vi "MAIN - PECT - Autonics - Pulses - encoder  - DATN.vi"() -> ()   [LabVIEW 2018]
uses:
  Control 1.ctl
  <vilib>/DAQmx/read.llb/DAQmx Read (Counter U32 1Chan 1Samp).vi
  <vilib>/DAQmx/write.llb/DAQmx Write (Analog 1D Wfm NChan NSamp).vi
  <vilib>/DAQmx/create/channels.llb/DAQmx Create Channel (AO-Voltage-Basic).vi
  <vilib>/DAQmx/configure/timing.llb/DAQmx Timing (Sample Clock).vi
  <vilib>/DAQmx/miscellaneous.llb/DAQmx Fill In Error Info.vi
  <vilib>/NI/Modbus Library/API/Wrapper/Create Serial Master.vi
  <vilib>/DAQmx/create/channels.llb/DAQmx Create Channel (CI-Count Edges).vi
  <vilib>/Instr/_visa.llb/VISA Configure Serial Port (Instr).vi
  <vilib>/DAQmx/create/channels.llb/DAQmx Create Channel (AI-Voltage-Basic).vi
  <vilib>/DAQmx/configure/trigger.llb/DAQmx Start Trigger (Digital Edge).vi
  <vilib>/Utility/file.llb/Write Delimited Spreadsheet (DBL).vi
  Global_data.vi
  <vilib>/NI/Modbus Library/API/Master/Modbus Master.lvclass
  <resource>/objmgr/daqmx.rc
  <vilib>/Platform/NI_3dgraph.lvlib
  <vilib>/NI/Modbus Library/API/Wrapper/API Main.lvlib
panel:
  in  "COM 2":refnum<visa-resource-name>="COM12"
  out "Record path 2":path=path "H:/ECT - HUY/Data Collection/PECT_default.tdms" caption="selected path"
  out "element":dbl
  out "Z UP Limit":bool
  out "X L Limit":bool
  out "Y Back Limit":bool
  out "Limit Sensor":bool[](array[boolean])
  out "exception status":u8=1
  out "Get data Count":u32
  out "Numeric":i32=2806
  in  "low cutoff freq: fl":dbl=40.0 format="%0.2f"
  out "Step Y Number":i16=40
  out "X complete":bool
  out "Y complete":bool
  out "Z complete":bool
  out "Init pulses":i32
  out "Enum":T1(ring)
  in  "Stop Scan":bool
  out "Count Y step":i32=40
  in  "file path (dialog if empty)":path=path "filename.csv"
  out "Init pulses":i32
  in  "2D Array In":dbl[][](array[numeric])
  out "Output":dbl[][](array[numeric])=[[-0.0001790493709009043, -0.00021608679972030288, -0.00017178819100872444, -0.00011604105280902267, -0.0001994752461753511, -0.00021272668316708356, -0.00020639924249934213, -0.00014664339243822874, -0.00017436953505067972, -0.00019232423942228908, -0.00020273889745070755, -0.00020023639620674223, -0.00021020175039261797, -0.00024359074063426845, -0.00025876701562411054, -0.0002315828160822644, -0.000218566532529974, -0.00022261110447328696, -0.00022419728135687593, -0.00021114867784790235], [-0.0001963216140493263, -0.00023418906975044163, -0.00019071104323735346, -0.00013561106555918905, -0.00021894092056332169, -0.0002380097564790417, -0.00022843365448356728, -0.00016484725168345368, -0.00018622702377611884, -0.0002031771821091096, -0.00021081005970256892, -0.00021079969316724172, -0.0002271961406782536, -0.00025867959672668146, -0.0002805477174689687, -0.00025169216832681383, -0.00024361837001232386, -0.0002460942661830067, -0.00025163155596480587, -0.00023850761662319413], [-0.0002081151685617141, -0.00024400248184640837, -0.00020530435414019364, -0.00015627208737854694, -0.00023343018819932046, -0.00025538735407167404, -0.0002426185756957697, -0.00017673621895774542, -0.0001884261364834142, -0.00020296298573773547, -0.00020689734150807198, -0.00020789870881424144, -0.00023303031169973065, -0.0002620433904484054, -0.0002927385048416735, -0.00026513120745070336, -0.0002623455059006857, -0.0002622931063832219, -0.0002723410056474345, -0.00026120095337865343], [-0.00021457669052360028, -0.00024580131506114853, -0.00021534259616615235, -0.00017707145978625594, -0.00024277432324072614, -0.0002634501756083648, -0.0002474815580328412, -0.00018035729110340779, -0.00017981645877632527, -0.00019103188878050962, -0.00019061251357036652, -0.00019092090894159974, -0.0002261842240830498, -0.00025290078244219645, -0.00029425058621379736, -0.0002719206490032662, -0.00027423707068698067, -0.00027095537529682294, -0.00028540039652625703, -0.00027818437178321], [-0.0002165532745462377, -0.00024080481503230104, -0.00022087843392969066, -0.00019612739674833984, -0.00024735703614447817, -0.00026179399751959966, -0.00024256467997271856, -0.0001746401468614477, -0.00016065367790241147, -0.00016820409511847725, -0.00016363767940926702, -0.0001613497984716203, -0.00020647740181520442, -0.00023164618907714658, -0.00028488226638064863, -0.00027270018072409613, -0.000279710414873696, -0.00027273738980523356, -0.0002908735183031882, -0.00028908854550584433], [-0.00021620251694465416, -0.00023191698381073642, -0.0002230430950540133, -0.00021189455575721262, -0.000248364593678687, -0.00025152551858054987, -0.00022906405584130745, -0.00016001345604591943, -0.00013303439830161627, -0.0001381008470128873, -0.00013039961934990015, -0.00012384473248759544, -0.00017604836265911004, -0.0002001991370624047, -0.0002659011078593801, -0.00026867397840984845, -0.0002805644526617879, -0.0002698382980896863, -0.00029061166615720457, -0.0002947373856622016], [-0.0002157254797925199, -0.00022212977202190273, -0.00022315741434436424, -0.0002226726523806592, -0.00024690632677282307, -0.00023481366928883914, -0.00020881322768553142, -0.00013812478894460224, -0.00010058736075877969, -0.00010585283298349471, -9.708551728018332e-05, -8.517212615390558e-05, -0.0001387897057735744, -0.00016136384157795173, -0.00023898033700647282, -0.0002608466807478317, -0.0002788558845781622, -0.00026484809900805505, -0.0002871755028366991, -0.0002961480206756994], [-0.00021603641939044876, -0.0002137231836458718, -0.00022219074041363376, -0.00022690682897293785, -0.00024332666516588709, -0.00021415534240340744, -0.00018362219034633118, -0.00011110986228331579, -6.715165937727641e-05, -7.697170186800155e-05, -7.038763051885923e-05, -5.229359285039217e-05, -9.933000506378957e-05, -0.00011790253758049707, -0.00020572727094640524, -0.0002493148562135129, -0.00027541277335358435, -0.00025964181137286095, -0.0002827092296243134, -0.0002940627952659853], [-0.0002169035043912259, -0.00020781952269694447, -0.00022081576894823676, -0.00022401076191313866, -0.00023740842840563013, -0.0001917459427821051, -0.00015533101101162725, -8.141641520546632e-05, -3.677306791602386e-05, -5.649535159940166e-05, -5.6193755228333385e-05, -3.1374570531067514e-05, -6.222214101951097e-05, -7.321569423801837e-05, -0.00016804225033060192, -0.00023388406793614126, -0.00027083358556014275, -0.0002553354757163593, -0.0002787410131176154, -0.00028917189047822194], [-0.00021821840400503695, -0.00020555322517243173, -0.00022034774503409873, -0.00021534561977678158, -0.00022979264904391533, -0.00017033179451306918, -0.00012640397324480395, -5.262818969476758e-05, -1.398636303178314e-05, -4.9120187782888784e-05, -5.9371588115307225e-05, -2.752973568791086e-05, -3.26114629992328e-05, -3.1644664187363905e-05, -0.00012894743083449733, -0.00021544938621673951, -0.00026614129881038454, -0.0002531053772280908, -0.0002768499554673797, -0.0002827767249597747], [-0.00021971567038365364, -0.00020713831401349483, -0.00022165114634856327, -0.0002038973398694431, -0.0002210396548240753, -0.0001527773117743509, -9.958363826534627e-05, -2.845518478239613e-05, -2.6082336154050964e-06, -5.736457030775313e-05, -8.184897875371244e-05, -4.306583216132521e-05, -1.5057604216061476e-05, 2.2469734134167307e-06, -9.237523956017249e-05, -0.00019543032274441964, -0.00026224558475180636, -0.00025371208640000836, -0.0002780424531135554, -0.0002765116974136287], [-0.00022052625489159868, -0.00021153638649906194, -0.00022415935129582384, -0.00019290682443156605, -0.00021179517790951077, -0.000140448560702563, -7.68519230142442e-05, -1.139633755409264e-05, -4.163431709398868e-06, -8.029008212839112e-05, -0.00012117111044296271, -7.601679390248275e-05, -1.1402969221721744e-05, 2.4607611376235503e-05, -6.186919659878845e-05, -0.0001751738305670672, -0.00025898183190682655, -0.0002563885732456842, -0.0002814375012646017, -0.00027118440513041776], [-0.00021988279893717967, -0.00021701712244094618, -0.00022686972936503732, -0.00018527605280643528, -0.00020245299908791797, -0.00013432743404399178, -6.010979957391232e-05, -3.243898764096996e-06, -1.8127979503059985e-05, -0.00011355463987814014, -0.0001706470877882284, -0.00012079385206513905, -2.117789106222904e-05, 3.3133968422815324e-05, -4.030060753122157e-05, -0.000156731644411396, -0.00025622278267901574, -0.00025973560929374966, -0.00028533901671389666, -0.0002663448542542593], [-0.00021869524322359803, -0.00022292426583044034, -0.00022957159776307474, -0.00018383638416337618, -0.0001945769406340673, -0.0001355721125065627, -5.1955433580346336e-05, -5.643698180804457e-06, -4.291334196600185e-05, -0.00015151877239863703, -0.00022183959462050186, -0.00017019364465732482, -4.275491119068702e-05, 2.5883392461202408e-05, -3.089693044187013e-05, -0.00014317907781097663, -0.00025452421274259167, -0.0002632516325736184, -0.00028859636972583796, -0.0002622101624978803], [-0.00021807632184133938, -0.0002284186202907209, -0.0002323572455590235, -0.0001900311787604277, -0.00018990549150125526, -0.00014456579006633455, -5.46658082891437e-05, -1.9712568408037506e-05, -7.552321975018862e-05, -0.00018753529480355913, -0.00026537002704973313, -0.00021653468959309443, -7.321263061649177e-05, 2.4565443021117017e-06, -3.6057369009415835e-05, -0.00013757609722403995, -0.0002547341878125775, -0.00026658745573897216, -0.000290396337119048, -0.0002587860129133193], [-0.00021824693795097824, -0.00023255751295601923, -0.00023399679294544822, -0.00020236475540265017, -0.00018868118663900764, -0.00016001554143172964, -6.873145959066136e-05, -4.4853397061619775e-05, -0.00011128138135851808, -0.00021465512057469716, -0.000292593471797456, -0.00025183562991200337, -0.0001079597385926145, -3.4452551596194855e-05, -5.556996295917865e-05, -0.00014129442097626788, -0.0002562315642660627, -0.00026846214110181395, -0.00028935633732405167, -0.0002549654006845474], [-0.0002190124687307584, -0.0002336622211642379, -0.0002332963769903964, -0.0002178223751308139, -0.00019078123902312172, -0.0001796474326783027, -9.356994101829101e-05, -7.90461361291862e-05, -0.00014567379324155125, -0.0002281437284970527, -0.0002977797118965701, -0.00027021284524483564, -0.00014255262148564225, -8.114311690595594e-05, -8.78966978550659e-05, -0.00015415177964126035, -0.0002578570700149576, -0.00026786253133153325, -0.00028423282585513746, -0.00024932257209576026], [-0.0002209894909040635, -0.00023258605736042274, -0.00023086429244803877, -0.00023391976265087818, -0.00019676517724666418, -0.00020170765223306072, -0.0001285461921752386, -0.00012121792800615701, -0.00017673068398968775, -0.00022815716173888757, -0.0002815327615322853, -0.0002711249085974501, -0.00017565725777078135, -0.00013480518097056665, -0.00013190373585706197, -0.00017625062963520528, -0.0002599023668556832, -0.0002652779776636336, -0.0002763846957686009, -0.00024273056924111434], [-0.00022448103990486967, -0.00022995484575597924, -0.00022743601940196714, -0.0002481970708736233, -0.00020664541522020206, -0.00022476654008557993, -0.0001720715687212734, -0.0001699835813927554, -0.00020468330736781067, -0.00021885354686507642, -0.0002498421058764067, -0.0002581606172256971, -0.0002075110135537385, -0.00019290046149774386, -0.0001853412547840414, -0.00020658123717641648, -0.0002627214515831056, -0.0002619127314163819, -0.00026816486335987447, -0.0002368600699934201], [-0.00022802990418745867, -0.00022622419022567952, -0.0002228884128917209, -0.00025791375153528303, -0.00021898606478551724, -0.00024649601851316205, -0.00022058652422207118, -0.00022214184915811137, -0.00023037764919299486, -0.000205995517291265, -0.0002113554698303403, -0.00023710405402949976, -0.00023905235376544837, -0.00025198658293546297, -0.00024399485024785734, -0.00024167752450870387, -0.0002651814590316536, -0.00025759189670814583, -0.00026058977742285817, -0.00023226638767936438], [-0.0002300235694701249, -0.00022125297023187392, -0.00021732519949127418, -0.0002611085228502331, -0.00023120009393905704, -0.00026436343821099103, -0.00026961587606469124, -0.0002743180137223314, -0.0002556005725403328, -0.00019656950892984765, -0.00017604240959999146, -0.00021504501881012845, -0.0002713622800732665, -0.0003089994852245627, -0.0003027606077411855, -0.00027720026736847807, -0.00026616966575180104, -0.0002522647713825805, -0.0002540660232651379, -0.00022905691282559034], [-0.00023031743114585324, -0.00021680314617144973, -0.00021203134821502073, -0.0002583345727852635, -0.00024209408782833487, -0.00027807224975191, -0.00031614712423959183, -0.00032422132876758214, -0.00028371709390885656, -0.00019828078315496482, -0.00015446067853002506, -0.00020121901701677415, -0.0003068498770553863, -0.0003622575261073985, -0.00035804543010948923, -0.00030981177381165636, -0.00026605710122575964, -0.0002471325457118192, -0.00024995322491891056, -0.0002283275116831034], [-0.00022925437043681916, -0.00021401448875409037, -0.0002088160831638262, -0.00025150958339171647, -0.0002509707154453953, -0.0002881907102463919, -0.0003576459341527987, -0.0003696771078116846, -0.0003171003697626006, -0.00021620692345035095, -0.00015457114485214422, -0.00020271610595858428, -0.0003466357604870324, -0.0004104672349350977, -0.00040669711287723287, -0.00033683898800164654, -0.00026552925347518835, -0.0002434535026422614, -0.0002489311645275244, -0.00023087596507603142], [-0.0002264612182456818, -0.00021276085301088522, -0.00020767484086169075, -0.00024205196843881532, -0.0002559667863855121, -0.0002942275945028369, -0.0003908887088360669, -0.00040764857374859945, -0.00035487226071887704, -0.0002503856107330272, -0.00017811286436661064, -0.0002216305231266466, -0.0003888450233332074, -0.00045060196307922067, -0.00044463481359120066, -0.00035502106061481575, -0.0002638439938361884, -0.00024050401004175898, -0.00024963464684412545, -0.00023542214933805396], [-0.00022185157032744967, -0.00021183543416352854, -0.00020739389445804599, -0.00023168051739573883, -0.00025599774849148493, -0.0002953195608101783, -0.00041319213849610147, -0.00043504694261567575, -0.00039361464277166015, -0.00029609294256662325, -0.0002216759940034561, -0.0002560863217725626, -0.0004293861275892121, -0.00047988354297975617, -0.0004689864061062383, -0.0003621240268398204, -0.00025980701284888767, -0.00023720275290790589, -0.0002498913303349351, -0.00023971721343348656], [-0.00021693350273486924, -0.00021145578995785362, -0.0002081366037133001, -0.00022290009811798493, -0.00025163705106371215, -0.00029243134032067367, -0.0004244182852297879, -0.0004511395398208171, -0.0004298355191403678, -0.00034709338188631655, -0.0002791656300998686, -0.0003018670029816817, -0.0004647697640870717, -0.0004975110739241333, -0.0004793376586334462, -0.0003591041475856944, -0.0002544362664846818, -0.00023447160214393973, -0.00024951846271172376, -0.00024363904996959392], [-0.00021329358353667366, -0.00021184599040914576, -0.00021003291024809193, -0.00021724072743727323, -0.0002443000969422626, -0.00028670062840463473, -0.00042560628093420323, -0.0004562722685524474, -0.0004597014113322034, -0.00039567051251991354, -0.00034218831377467486, -0.00035226127247373236, -0.0004915854197046193, -0.0005035696601653908, -0.00047688331048914394, -0.0003483540322680844, -0.0002492522603439124, -0.00023275086686351098, -0.0002491402431873957, -0.00024770821903495697], [-0.0002111396353729235, -0.00021141958914673055, -0.0002117295808062563, -0.00021403939548415504, -0.00023465741620782958, -0.0002780322951085844, -0.00041675502640222024, -0.00045031625597639555, -0.00047806778777350744, -0.0004331240508939618, -0.000399951477056998, -0.00039841333258215823, -0.0005057534016851654, -0.0004977962905883442, -0.00046237570541058336, -0.00033129712796658474, -0.00024399196409514382, -0.00023102257587082238, -0.000248294776308949, -0.0002506553417561917], [-0.0002099507444262268, -0.0002092158988426249, -0.00021186994635026286, -0.0002112926091797961, -0.0002232120564579377, -0.00026642921614820035, -0.0003983369808760436, -0.0004339299808601262, -0.00048159860180152763, -0.00045248659421314157, -0.00044336761498752885, -0.00043214549596420297, -0.0005048678971218534, -0.0004809285840771671, -0.00043700613799681556, -0.0003102589439363604, -0.00023838864446115195, -0.00022810695668517775, -0.00024679485465158024, -0.0002515946310250091], [-0.00021067038348659365, -0.00020606210782104627, -0.00021080963190575445, -0.0002083997893175182, -0.00021257105479688052, -0.00025352476878359037, -0.00037331291966480676, -0.00040993579354319746, -0.0004706887564761208, -0.00045244163459400716, -0.00046794050450717044, -0.0004492170481778541, -0.0004901664343216188, -0.0004559537249311319, -0.00040456079458894845, -0.0002889715853185166, -0.00023366889282603123, -0.00022448506679441718, -0.00024621160093700467, -0.00025164985053700503], [-0.00021366771338320652, -0.00020303500058891939, -0.00020923510335117343, -0.0002050845727041466, -0.0002047091969661673, -0.000241372618557922, -0.00034476877382140676, -0.0003817668060293851, -0.00044809290861421314, -0.0004352568307386161, -0.0004727370419142802, -0.0004488493531815277, -0.0004648618686007768, -0.00042650700417049686, -0.0003688275214315945, -0.00027044749710170533, -0.0002307677151872061, -0.00022096729112685773, -0.00024799835519775937, -0.00025155341466853894], [-0.0002173084769872, -0.00020026823278414523, -0.0002070542311710319, -0.00020015250188109603, -0.0002000513255038163, -0.00023053307114026707, -0.0003145428960598818, -0.0003514169088703672, -0.0004168005893498, -0.0004049406521434125, -0.00045892801090032485, -0.00043201284544968493, -0.00043222145004994, -0.0003943985377895462, -0.00033206395965079336, -0.0002553862802279327, -0.00022864313887302132, -0.00021671670797258902, -0.0002513135661791916, -0.0002504859997362087], [-0.00021973461338017225, -0.00019724665283585296, -0.00020386728125797345, -0.00019303995213347785, -0.00019775389133368237, -0.00022113133999670208, -0.00028392228670897843, -0.00032062204951827534, -0.0003801517417093541, -0.0003667313828948429, -0.0004294578127631808, -0.000401957035489061, -0.0003950886551043458, -0.0003608958802723376, -0.0002961293070477822, -0.00024331685442430598, -0.00022617809942428353, -0.00021102885268738103, -0.0002543656101950207, -0.0002472402816616325], [-0.0002206887087533825, -0.00019500358276167314, -0.00020086006895508185, -0.00018551371218804118, -0.00019833298545421894, -0.0002139552840322318, -0.00025547719890561295, -0.00029169894301897276, -0.00034299697181030576, -0.0003275896561808281, -0.00039026103052590584, -0.0003647320171096934, -0.00035746465701116427, -0.0003281200463100698, -0.00026407214123304323, -0.00023474498730902127, -0.0002235404145244195, -0.0002051469041781228, -0.000256505003176994, -0.00024213742773926926], [-0.0002200062764148962, -0.00019375515469029908, -0.00019918211441145514, -0.00017991991813800373, -0.00020152554963176646, -0.00020951090642230656, -0.00023129959162584632, -0.0002663889238850078, -0.00030955488127189235, -0.00029309743662717797, -0.0003476285707827778, -0.00032647388485934105, -0.00032274144912027534, -0.0002972445447394015, -0.0002388416732305998, -0.0002294946477340975, -0.00022115126064498232, -0.00020067986068869094, -0.00025731397996606176, -0.00023589062632908483], [-0.00021686501048460982, -0.0001927440667472552, -0.00019806643691439203, -0.00017708949207530245, -0.0002058442692531113, -0.00020618400807497113, -0.00021149103316543856, -0.0002446761750965164, -0.00028122237605033434, -0.0002654526859166579, -0.0003058249429885723, -0.00029101730155135785, -0.000291745117435337, -0.00026848333783359955, -0.00022112253118916798, -0.00022569318997046374, -0.00021784905484434, -0.00019767179850903316, -0.000255268465696977, -0.0002284943150350112], [-0.00021043663370824, -0.00019038513747410106, -0.00019675034047064027, -0.00017654974493035679, -0.0002090745294200981, -0.00020230231875758425, -0.00019566018647480983, -0.00022577217944666841, -0.00025804974232601294, -0.00024379879870907277, -0.0002671600070910888, -0.00025998657099316445, -0.00026429413659799506, -0.00024140387303679157, -0.0002098830622664534, -0.00022164186657965684, -0.00021293451613360603, -0.00019578932957465926, -0.00024893013102892866, -0.00021929410847857517], [-0.0002021357888212106, -0.0001870778760571564, -0.00019551363356000266, -0.000178176974235068, -0.00021082247374670446, -0.00019815233667355887, -0.00018409509890723527, -0.00021030691659366246, -0.00024044554621526285, -0.00022741798909153496, -0.0002343581826668769, -0.00023512599364226318, -0.00024112221561539, -0.00021724126955392428, -0.000204939399155446, -0.00021717071560331536, -0.00020731246535632408, -0.0001957224564036516, -0.0002394008241276193, -0.00020983643831130536], [-0.00019382942194914182, -0.00018317870523813437, -0.0001941112103125784, -0.00018154963028758908, -0.0002110898918876586, -0.00019433174451707544, -0.00017680372114179353, -0.00019922649032049974, -0.00022822032632894076, -0.00021510680810691435, -0.00020900005958195828, -0.00021705235159035809, -0.00022264956117902177, -0.00019770591605515302, -0.00020531190524905422, -0.0002122949737994994, -0.00020212454072031719, -0.00019755405791488725, -0.00022795337113398761, -0.00020207182781544972], [-0.0001860175705082779, -0.0001783739737073655, -0.0001910117451761513, -0.00018471750733600224, -0.00020913083625901524, -0.00019010122188476558, -0.00017207907477439187, -0.0001915344510088294, -0.00021925744913525898, -0.0002041423647054525, -0.00019054980596271143, -0.00020373106516728863, -0.00020773161302148867, -0.00018257527716223493, -0.00020792284781900178, -0.00020584489308989734, -0.000196989713765576, -0.00019930193401179568, -0.00021503376289837978, -0.00019561464459860213], [-0.00017879376008740275, -0.0001717064584350822, -0.00018476309314842052, -0.00018559894976801113, -0.00020480590122671713, -0.00018486588023933215, -0.00016786158341463436, -0.00018632062834771958, -0.0002113369243466768, -0.0001927692658922637, -0.0001773979918470673, -0.000192720077801755, -0.00019471455939610964, -0.00017140872935831122, -0.0002092132971061693, -0.00019705222472525888, -0.00019122525071702326, -0.00019850372670889883, -0.0002003325890270278, -0.0001897144334209195], [-0.00017343641024908027, -0.0001645933515064986, -0.00017635294578014458, -0.00018396783905104928, -0.00019949500913999697, -0.00018033933777524512, -0.00016440626646809994, -0.0001839362261671692, -0.00020391295827511952, -0.00018227037554012504, -0.00016925239197810617, -0.00018410608388137045, -0.00018403838738988154, -0.00016503978419010398, -0.00020830391074392815, -0.00018691686106615292, -0.00018556973370605252, -0.00019506772040221027, -0.00018574873069300904, -0.00018561174053887373], [-0.00017072220231029167, -0.00015819074237620814, -0.00016763614819010307, -0.00018045455462836063, -0.00019466693943955872, -0.00017771660432387183, -0.00016193896298990346, -0.00018494468575313595, -0.00019698459277234757, -0.00017454903012389424, -0.00016588496465524613, -0.00017817091981232706, -0.00017615332756484511, -0.00016375340095344665, -0.00020522285615905828, -0.00017730056045200775, -0.00018138934379164674, -0.00018951734167179345, -0.00017358717597895645, -0.00018419831111197126], [-0.00016915541325304186, -0.00015219351624800453, -0.000159387643616336, -0.00017499789685608905, -0.00019022581352073735, -0.00017628500034547884, -0.00015987065781666518, -0.00018775833623527194, -0.00018928909091247247, -0.0001699845375634102, -0.00016548833479338235, -0.00017429041320676276, -0.00017007185805722504, -0.00016547036080744384, -0.00019907210230285348, -0.00016847439743328252, -0.0001782680546483853, -0.00018176685618924958, -0.00016420877832335964, -0.00018438800922252266], [-0.00016699278247163732, -0.00014632730804036223, -0.00015232752566938373, -0.00016791096343255624, -0.00018508281548767526, -0.0001747089667313538, -0.00015781921803309854, -0.00019041650760125324, -0.0001799236005517093, -0.00016849412127567173, -0.00016551579334978146, -0.0001714686137914978, -0.00016480792515188684, -0.0001678295020885283, -0.00018984750127565286, -0.00016082647855846302, -0.00017569466438790288, -0.00017270321628911137, -0.0001574938738205245, -0.00018481938214680652], [-0.00016410001152501047, -0.00014186259211697652, -0.00014802534339525275, -0.0001607067167921014, -0.00017926766205520264, -0.00017362990827877317, -0.00015709070779591425, -0.00019241246169750953, -0.00016995278281397436, -0.00017066850882714937, -0.000165319202652333, -0.0001703036409766573, -0.00016109745107906193, -0.00016983565748885515, -0.00018004226780877347, -0.00015609624105985404, -0.00017472749272075955, -0.00016484129434302108, -0.00015467782742988045, -0.00018573758749646646], [-0.00016084986376483854, -0.00014033310805317, -0.0001475633763562273, -0.0001551088133728666, -0.00017301756284093285, -0.00017348401648135253, -0.00015918266819851812, -0.00019316370053601255, -0.00016069312051794453, -0.00017571765849012586, -0.00016438158502175663, -0.00017070108696826125, -0.0001596368322853963, -0.0001707002480070413, -0.00017208685775431734, -0.00015536636226637715, -0.00017603568890164553, -0.00016091901728864863, -0.0001565167845689712, -0.0001870328244625366], [-0.00015639969111759348, -0.00014129264741064712, -0.00015004387540913482, -0.00015140032271324447, -0.00016517213699152912, -0.00017305218302528583, -0.00016357685144966633, -0.00019107583144396811, -0.00015203980741492103, -0.00018086043613242501, -0.00016068854804591332, -0.00017020492358917234, -0.00015921944021283184, -0.00016847929553197305, -0.0001660848191834801, -0.00015743309256275803, -0.00017859765998816737, -0.00016138241415626468, -0.00016150211035736994, -0.00018695987427767152], [-0.0001504756550961793, -0.00014427879543442088, -0.000153722090473438, -0.00014937719908233657, -0.0001550955403737276, -0.00017103835956116913, -0.0001691974521458063, -0.000184640068940407, -0.00014319975198578104, -0.00018196067900595574, -0.00015228770627697188, -0.00016604089893557626, -0.00015756368737504176, -0.0001616084349536709, -0.0001612433447031117, -0.00016013398959609758, -0.00018075365158499827, -0.00016507700159299442, -0.00016674765418513843, -0.00018358679723059178], [-0.00014464095866733445, -0.00014888851792758603, -0.00015847136364592444, -0.0001497133019401787, -0.00014464187544306444, -0.00016794480540712094, -0.00017567288627944044, -0.0001741000659076595, -0.00013436338150374372, -0.00017652875428644799, -0.00013900091737155222, -0.00015657036525163273, -0.00015343911368784907, -0.00015071842497925772, -0.00015741003278019194, -0.00016256346628940217, -0.00018202343394861827, -0.0001717513783275823, -0.00017089798421427577, -0.0001768366253569898], [-0.00014021021504910525, -0.0001550240847418352, -0.00016372606648647203, -0.0001522709920078521, -0.0001358951182032081, -0.00016434583840006442, -0.00018207259631463843, -0.00015999238209924403, -0.00012533789422008133, -0.00016301045477310448, -0.00012087633606610963, -0.00014015025580808166, -0.00014529433732743229, -0.00013644834938181596, -0.00015362968705793373, -0.00016368063193316143, -0.0001822704530242622, -0.00018047156328695156, -0.00017338649061151255, -0.00016766064947300145], [-0.0001371883010907824, -0.00015998602159566187, -0.00016734360622347455, -0.00015560208178362796, -0.0001298119700644633, -0.00015933515494750972, -0.0001858539978381677, -0.00014170567666968968, -0.00011371780323028192, -0.00013914038658818968, -9.647965896794272e-05, -0.00011427184123393407, -0.00012966121739446494, -0.0001180767767005736, -0.00014713504793646345, -0.00016115426427446705, -0.0001803058414129692, -0.00018818343053249136, -0.00017271968582245265, -0.0001560928612509508], [-0.00013512164576080093, -0.0001614900884085481, -0.00016759861043179163, -0.000157979487867152, -0.00012671329854465826, -0.00015213002775576329, -0.00018404700490480715, -0.00011851980504043111, -9.675349740125017e-05, -0.00010372273216048208, -6.52605838859649e-05, -7.744379778600909e-05, -0.00010362010717435838, -9.453986064667831e-05, -0.00013461268718219753, -0.00015307911859663466, -0.00017501861748123876, -0.00019230678326665612, -0.00016836300504778634, -0.000142559856841612], [-0.0001346116757000703, -0.0001593100492798174, -0.00016448382508829802, -0.0001589892764972834, -0.00012773083849505762, -0.00014372431447308605, -0.00017597402246963614, -9.147320172413903e-05, -7.327284950731094e-05, -5.856542512870308e-05, -2.8501290426535472e-05, -3.1721359869363655e-05, -6.641378896274364e-05, -6.570773037198677e-05, -0.00011457455983197515, -0.00013994496313747898, -0.00016751755682483868, -0.00019234482792972706, -0.0001618195614770581, -0.00012966197619128372], [-0.0001358810317147463, -0.00015426651546611957, -0.00015855271914321997, -0.00015870014973728107, -0.00013282044152148828, -0.00013535896029822497, -0.00016136206945210722, -6.217036253441596e-05, -4.28250031337396e-05, -6.911738209184823e-06, 1.1299140246548087e-05, 1.8919184375547002e-05, -1.9148134360130742e-05, -3.169628646025775e-05, -8.617115885197618e-05, -0.00012248153230588754, -0.00015926364746193453, -0.00018897323032828796, -0.00015519428865971158, -0.00011944154031763923], [-0.00013731686752789865, -0.00014627964208726446, -0.00015027761599318602, -0.0001561476147983465, -0.00014009720845709235, -0.0001267299036625518, -0.00013922967793058953, -3.039275564033217e-05, -4.800175297657583e-06, 4.779986232539453e-05, 5.1773779457146146e-05, 6.996490226551452e-05, 3.588152175987118e-05, 8.456214243815832e-06, -4.783196571215599e-05, -0.0001002032683363515, -0.00014956492442800076, -0.0001818339405597301, -0.00014877456642661824, -0.00011212799639204532], [-0.0001376237380223827, -0.00013620350359520167, -0.0001406759823552109, -0.00014998399133876739, -0.00014698075062368442, -0.00011719445859587237, -0.0001092923113923984, 3.4081056138387383e-06, 4.000069373872109e-05, 0.00010125505621800049, 8.941129165612044e-05, 0.00011539334598236785, 9.465593105455368e-05, 5.506887886252282e-05, 6.908492349612383e-07, -7.254467161760779e-05, -0.00013791887622742298, -0.00017074905773294298, -0.00014176288017819783, -0.00010725469375568245], [-0.00013684129874163772, -0.00012698036323311075, -0.000132538051196774, -0.00014153492407491426, -0.00015275428679373433, -0.00010805310205338516, -7.428502884131334e-05, 3.711880536450517e-05, 8.707049226566906e-05, 0.00014701132803420988, 0.00011778600817575861, 0.00014679779218529886, 0.00014938321354322943, 0.000104728249110864, 5.593465342915854e-05, -4.108305711105972e-05, -0.0001252784085827366, -0.0001581946848339174, -0.00013534108131697462, -0.00010508260295318504], [-0.00013486006254005353, -0.00012096183850079587, -0.0001284688841031844, -0.00013319707694759222, -0.00015681708165782987, -0.00010022993223313646, -3.777363450107804e-05, 6.886985228148068e-05, 0.0001305497962792463, 0.000178931463008139, 0.0001302367976741374, 0.00015665895648558567, 0.00019134426189420899, 0.000152542215341403, 0.00011270759217153759, -7.922193309237158e-06, -0.00011291844425178992, -0.0001470663246446076, -0.0001305050341417497, -0.00010547597809917701], [-0.0001311917136155357, -0.00011854515329906903, -0.00012830876444580586, -0.00012558771260558557, -0.0001578354397061294, -9.311920335685654e-05, -2.2467428044768006e-06, 9.730838899234956e-05, 0.00016601561593673417, 0.00019310586813440014, 0.00012301885372871697, 0.0001412577706695825, 0.0002141013235983872, 0.00019401821707107705, 0.00016632126846071252, 2.5995111192238587e-05, -0.0001004789302455518, -0.00013803753706143063, -0.0001268936652260872, -0.0001073229082476819], [-0.00012502312180468454, -0.00011885542800798773, -0.0001306913781935863, -0.00011893601811575026, -0.000154286146253884, -8.596917367130995e-05, 2.9223055931967487e-05, 0.00012115187445066455, 0.00018960122856041817, 0.0001882953455529194, 9.544702246854463e-05, 0.00010118693214517666, 0.00021364861223296082, 0.00022463720363575038, 0.00021152984273965086, 5.8667624762502243e-05, -8.783296028221609e-05, -0.00013123195884452363, -0.00012400711212480833, -0.00010945628234779702], [-0.0001175920332645141, -0.00012148737676645482, -0.00013456166538736332, -0.00011480034659066586, -0.00014734510054162375, -7.994882108361412e-05, 5.2326165625653925e-05, 0.00013784480361868356, 0.00019766883933897833, 0.00016453875269898527, 4.889895892876313e-05, 4.00079406305022e-05, 0.00018837645832830117, 0.00023897285383033678, 0.00024170411497220073, 8.584659561846307e-05, -7.671413863280171e-05, -0.00012811153417364302, -0.0001235341461005221, -0.0001119768155519521], [-0.00011073888193134651, -0.0001258082596827005, -0.00013809825972990568, -0.00011467686350870136, -0.00013829246388562255, -7.649994609324785e-05, 6.32311393845477e-05, 0.00014402391747898, 0.0001885336120149815, 0.00012482410366557, -1.1157888753554612e-05, -3.4046454265641846e-05, 0.00014121391719891692, 0.00023386620967224755, 0.0002514772885735539, 0.0001029067884977912, -6.943047489586622e-05, -0.0001292679444411457, -0.0001268980133788157, -0.0001153221424620033], [-0.0001047296327158706, -0.00012976066616450684, -0.0001386300101499649, -0.00011766051924777879, -0.00012778594145599134, -7.579233846657582e-05, 6.042314947392671e-05, 0.00013852499167196775, 0.00016471695179091743, 7.605424596430002e-05, -7.455380871402087e-05, -0.00010798154346389373, 8.038151411852296e-05, 0.0002103319053651572, 0.00023973892810755758, 0.00010767759168635489, -6.63601107989166e-05, -0.00013354374606004867, -0.00013345454360122293, -0.00011859203794866574], [-9.95799413894792e-05, -0.00013100088621080877, -0.00013450100391171511, -0.00012167540813057785, -0.00011658134532758699, -7.746443078980939e-05, 4.430580123484379e-05, 0.00012109722076506825, 0.00013044586732132747, 2.6667987409374067e-05, -0.00012944174678540012, -0.0001680972211710232, 1.6810185072864067e-05, 0.00017168769132371552, 0.00020771637388542104, 9.880088373222067e-05, -6.738213989441501e-05, -0.00013845368909545623, -0.00014119522952489236, -0.00012061112048289066], [-9.657607873522073e-05, -0.0001295733477046073, -0.00012678719732973735, -0.00012540393435989984, -0.00010736999655015268, -8.297224301626743e-05, 1.5047283961667351e-05, 9.078985883825309e-05, 8.9043074027996e-05, -1.714903043647034e-05, -0.00016688788682481769, -0.0002045664848381347, -4.037690713844244e-05, 0.00012110947595051977, 0.00015688544821593556, 7.470254902255773e-05, -7.331717117388045e-05, -0.0001432173403470762, -0.00014938412487555328, -0.00012185824697459602], [-9.648024881366533e-05, -0.00012618216368176505, -0.00011745312447093009, -0.00012799814353481667, -0.00010265822171590805, -9.284721177416078e-05, -2.559555604009396e-05, 4.761410115322086e-05, 4.351312901748616e-05, -5.183177973138928e-05, -0.0001816447248019215, -0.0002121404980918208, -8.494162415797861e-05, 6.216843859732299e-05, 9.03882717625485e-05, 3.558141340474774e-05, -8.495694364270799e-05, -0.0001472992804255214, -0.00015723401108144394, -0.00012252351822082674], [-9.798274395027458e-05, -0.00012012058928547419, -0.00010773306872560381, -0.0001278954727353815, -0.00010248893268937145, -0.00010567994414527326, -7.29133422679145e-05, -5.343614721634374e-06, -3.34998281340676e-06, -7.545898315405343e-05, -0.0001724715863591561, -0.00019089947508595453, -0.0001129926387609722, -7.860923886791882e-07, 1.3593592848294006e-05, -1.541821269138155e-05, -0.00010092692719796022, -0.00014873599166442125, -0.0001624429621619912, -0.00012176291289599933], [-9.956054467338306e-05, -0.00011125253368178371, -9.84869306676333e-05, -0.00012352211607181453, -0.00010588061072737236, -0.0001193775915704267, -0.00012156932428064073, -6.392611006315711e-05, -5.023683125419259e-05, -8.968279518152197e-05, -0.00014341854747669872, -0.00014706836363469894, -0.0001255587348114838, -6.415241069209279e-05, -6.85002889604519e-05, -7.401802233430489e-05, -0.00011911506258907752, -0.00014613492164287922, -0.00016308904972539041, -0.0001187178378218301], [-0.00010046649651081381, -0.00010103445879613634, -9.11728416933405e-05, -0.00011520486639218612, -0.00011167871735503869, -0.00013310879396772127, -0.0001675627054012769, -0.0001252935222823444, -9.881491628845052e-05, -0.0001006492300604199, -0.00010497717222184011, -9.378473155756926e-05, -0.0001296546307104473, -0.00012725380185244634, -0.00015274883191985188, -0.00013663899179380823, -0.00013882945491881446, -0.00014046307570532608, -0.00015991326050426857, -0.00011396952604226379], [-0.0001003908235543971, -9.096601183869457e-05, -8.625232294776249e-05, -0.00010453770268752278, -0.00011844702690064039, -0.00014539622919146865, -0.00020748140420947386, -0.00018631100758152372, -0.0001508429979253656, -0.00011541775088221191, -6.990052883895995e-05, -4.638242344691228e-05, -0.0001343830594482849, -0.0001901775080197718, -0.00023601955119829932, -0.00019894139653670734, -0.00015898819130751723, -0.0001334199910609183, -0.00015444472833785888, -0.0001085005950533062], [-9.82123928779978e-05, -8.092596930924303e-05, -8.178698781297414e-05, -9.219155657304995e-05, -0.00012268080467640885, -0.0001534844794750488, -0.00023703525866675644, -0.00024212010321908277, -0.00020587160050468747, -0.00013855929073426643, -4.878143641363214e-05, -1.7119304092788612e-05, -0.00014732834405463066, -0.00025145212939360617, -0.00031325051547472296, -0.00025477349707582995, -0.00017647672967285172, -0.00012531745519792428, -0.0001470238897666662, -0.00010203628781936189], [-9.296292003102904e-05, -7.062624132176537e-05, -7.527188690815978e-05, -7.838447685164229e-05, -0.00012145371849307807, -0.00015490988650294045, -0.0002534847895567776, -0.00028833462643155887, -0.0002612997299488093, -0.00017173774379877424, -4.856910627587703e-05, -1.4358685621180395e-05, -0.000172757474707394, -0.00030870698201744193, -0.00037893276344845225, -0.0002983875395885117, -0.00018822634806106749, -0.00011593176872355324, -0.0001375920237718202, -9.395020697693622e-05], [-8.541932390006973e-05, -6.126544170090287e-05, -6.63930839994685e-05, -6.521844037912783e-05, -0.00011453874798678272, -0.00014981734594458201, -0.00025712887368429214, -0.0003227312783483441, -0.0003145060844013739, -0.00021495735149216696, -7.252843584162373e-05, -4.158287122739933e-05, -0.00021256164470404536, -0.0003607488714504198, -0.00042963696623985956, -0.0003270717570537929, -0.0001931942002099795, -0.0001068556010837031, -0.0001277457084613888, -8.522220142128008e-05], [-7.707818583529286e-05, -5.3661437228656045e-05, -5.537811085587312e-05, -5.468921195421125e-05, -0.00010310543687560084, -0.000139011996614348, -0.0002492776316964495, -0.00034388470011407525, -0.00036145113630563913, -0.00026486273472690544, -0.00011821358212680752, -9.531135234633163e-05, -0.0002642860691946126, -0.00040507882653841726, -0.00046233875609616795, -0.0003393811426188626, -0.00019098540199815467, -9.946751118664401e-05, -0.00011895321507680856, -7.635493534177348e-05], [-6.772956150725637e-05, -4.675188350633172e-05, -4.212379414546101e-05, -4.624638851629184e-05, -8.783301321514149e-05, -0.00012277528789541269, -0.00023102479110356268, -0.00035042058265023594, -0.00039579962921777734, -0.00031369873448511623, -0.0001765929198475763, -0.00016531958778844696, -0.000319405717586008, -0.00043738733207363337, -0.00047359016511180387, -0.000334247250694069, -0.00018051650046799553, -9.246291566412587e-05, -0.00011039688916631568, -6.726788734949182e-05], [-5.701933613285956e-05, -3.9502128986823246e-05, -2.7893505107297323e-05, -3.92097495182861e-05, -6.973464320232485e-05, -0.00010157601759623255, -0.00020395409588214002, -0.0003416468082047541, -0.0004123628122863418, -0.0003531332274445201, -0.00023606755337511089, -0.00023781706184499742, -0.0003678807213612998, -0.00045394839671960424, -0.00046226291379085, -0.00031282142563628275, -0.00016169332294851957, -8.447875845913472e-05, -0.00010094728702140371, -5.744919239702301e-05], [-4.5890334780158276e-05, -3.180105040159753e-05, -1.559471053136363e-05, -3.411402275537746e-05, -5.116874220684013e-05, -7.78360541527686e-05, -0.00017142251318347929, -0.00031927234103750965, -0.00040904133763754527, -0.0003769210963750977, -0.0002859293776891914, -0.0003004299637531047, -0.00040113091355390915, -0.00045338446779802713, -0.00043082625744443777, -0.00027912633366135656, -0.00013684639632967344, -7.547141691572473e-05, -9.095443749381968e-05, -4.72805382863619e-05], [-3.469938587103219e-05, -2.3583992532001663e-05, -7.502280703749684e-06, -3.0199265075516943e-05, -3.3101305170219614e-05, -5.3733106268060576e-05, -0.0001362383793520397, -0.00028576615598670425, -0.00038592639173447123, -0.0003805701400914404, -0.0003172411807605413, -0.0003426736937746297, -0.00041265612506535126, -0.0004355115649202247, -0.00038342323926192703, -0.00023784293355944008, -0.00010890291332864635, -6.500279994623576e-05, -8.068385700324421e-05, -3.680488753171618e-05], [-2.29178629788801e-05, -1.4130826072463257e-05, -4.680724047780027e-06, -2.626913664384445e-05, -1.5197842712501991e-05, -3.0564607996908313e-05, -0.00010025844724554159, -0.00024308773434895958, -0.000345121292687673, -0.0003621970758800122, -0.00032433394428275225, -0.0003577763916138392, -0.0003992871398899433, -0.00040129906027053415, -0.0003246747927500987, -0.0001927657463495422, -8.014709043894022e-05, -5.2274975672103596e-05, -7.011824607974435e-05, -2.5662043645893404e-05], [-1.0187643536187924e-05, -3.659629807393344e-06, -6.804671206559962e-06, -2.0754580528706268e-05, 3.690799992127e-06, -8.71330931921134e-06, -6.495975542112134e-05, -0.0001935547133350233, -0.00029030128542601764, -0.0003228209364162203, -0.00030596028673975095, -0.00034404579224587076, -0.0003614636089203753, -0.0003527993682758898, -0.0002594055150362262, -0.00014676106529186786, -5.2854601797436285e-05, -3.638703467989668e-05, -5.877755855961814e-05, -1.3659715191367133e-05], [3.128959488736538e-06, 6.380492219059189e-06, -1.2637659253623285e-05, -1.3151381848220886e-05, 2.407351549743933e-05, 1.11985573658345e-05, -3.227936749661091e-05, -0.00014023496557769195, -0.0002270053521084784, -0.0002666675708141216, -0.00026583527189333843, -0.0003053002904970237, -0.0003037398923508485, -0.00029391357333577277, -0.00019266402441533992, -0.00010200993270183256, -2.9563611422391695e-05, -1.7551869899976036e-05, -4.7015247696111095e-05, -1.0198652534987307e-06], [1.667738967411382e-05, 1.4524070598662467e-05, -1.9986920933261557e-05, -4.0341851117713795e-06, 4.624732240485728e-05, 2.905836410442217e-05, -3.5799150538071145e-06, -8.588815104646104e-05, -0.0001608861512834847, -0.0001997323070541783, -0.0002106996450962923, -0.000248673679556919, -0.00023309848178103276, -0.00022915160072008514, -0.00012838829039780314, -5.983116877330413e-05, -1.1642826071502077e-05, 3.3134606720816584e-06, -3.493825606996903e-05, 1.2054436207102615e-05], [3.004398987871068e-05, 2.0214585662908097e-05, -2.5697816131681206e-05, 6.551176488771987e-06, 7.009769597039056e-05, 4.583782142041255e-05, 2.0824397499502947e-05, -3.278598496370133e-05, -9.631182502277749e-05, -0.00012843801015309, -0.00014798193943661025, -0.00018221675989681108, -0.0001566658951171196, -0.00016230452589776484, -6.842467332343616e-05, -1.981533706373398e-05, 1.559079493233112e-06, 2.5944748713247617e-05, -2.1499170110364507e-05, 2.5296178129442792e-05], [4.295340180268149e-05, 2.3187882335507642e-05, -2.730529661305707e-05, 1.8193506416065014e-05, 9.470782640946286e-05, 6.248449397097504e-05, 4.079094050257574e-05, 1.6577291772514394e-05, -3.710447523691887e-05, -5.9043790254117295e-05, -8.515168032477254e-05, -0.0001138886685537327, -8.140204314424984e-05, -9.708657371826357e-05, -1.443089744099929e-05, 1.8069257856270088e-05, 1.128094326186685e-05, 4.961627384511211e-05, -5.901923490377048e-06, 3.811537668805924e-05], [5.427341691318678e-05, 2.294834567218365e-05, -2.4269795002248434e-05, 2.906807135103287e-05, 0.000117192737121765, 7.837702855726693e-05, 5.5482667941942135e-05, 5.919704543974787e-05, 1.3004926536165987e-05, 2.305322343175778e-06, -2.9283795754201855e-05, -5.156276832292417e-05, -1.4138934868429542e-05, -3.8228354859320274e-05, 3.16079449810408e-05, 5.240275570747577e-05, 1.808500670089433e-05, 7.173748660962986e-05, 1.0941141723883052e-05, 4.9380316809238475e-05], [6.23362612884315e-05, 1.9584549567694745e-05, -1.738418622310861e-05, 3.706949316328867e-05, 0.00013451801808737028, 9.209319951961233e-05, 6.42809380241114e-05, 9.213606552491149e-05, 5.125902265078544e-05, 5.0919614513839084e-05, 1.4690896680097723e-05, -7.200695462741824e-07, 3.989579609767549e-05, 1.0421253604699782e-05, 6.766188254592187e-05, 8.090649597976979e-05, 2.2249777539933707e-05, 8.948588388116643e-05, 2.7399396416622618e-05, 5.789300145506854e-05], [6.674725407563274e-05, 1.4253594094066138e-05, -7.830736353749146e-06, 4.1482014158822356e-05, 0.00014453777003205215, 0.00010233511042052022, 6.76321318176503e-05, 0.00011373711017685813, 7.691996279594535e-05, 8.448629499516191e-05, 4.4914181156711225e-05, 3.619756792041379e-05, 7.829740595200266e-05, 4.697303627080457e-05, 9.30047408217588e-05, 0.00010207532947874992, 2.4742668153367176e-05, 0.00010110391899965585, 4.210028311419506e-05, 6.284725232370489e-05], [6.742413840521953e-05, 8.652276420495486e-06, 2.5888186730767954e-06, 4.2367381588115025e-05, 0.00014621140070691582, 0.00010803832750986599, 6.627173015242432e-05, 0.0001238916934743501, 9.057359638555904e-05, 0.00010274705629527078, 6.18346305165194e-05, 5.890217367737413e-05, 0.00010079344564996665, 7.060702567748822e-05, 0.0001073905845654019, 0.0001146192508746785, 2.6299059248519746e-05, 0.00010576240639711271, 5.3722464578607326e-05, 6.393009133981095e-05]]
  out "No.data":i32
  in  "Tab Control 2":T2(tab)
  out "Waveform Chart":dbl(graph)
  out "Record path":path=path "H:/ECT - HUY/Data Collection/PECT_default.tdms" caption="selected path"
  out "Feature extraction scan":dbl[](graph)=[-0.00020273889745070755, -0.00021081005970256892, -0.00020689734150807198, -0.00019061251357036652, -0.00016363767940926702, -0.00013039961934990015, -9.708551728018332e-05, -7.038763051885923e-05, -5.6193755228333385e-05, -5.9371588115307225e-05, -8.184897875371244e-05, -0.00012117111044296271, -0.0001706470877882284, -0.00022183959462050186, -0.00026537002704973313, -0.000292593471797456, -0.0002977797118965701, -0.0002815327615322853, -0.0002498421058764067, -0.0002113554698303403, -0.00017604240959999146, -0.00015446067853002506, -0.00015457114485214422, -0.00017811286436661064, -0.0002216759940034561, -0.0002791656300998686, -0.00034218831377467486, -0.000399951477056998, -0.00044336761498752885, -0.00046794050450717044, -0.0004727370419142802, -0.00045892801090032485, -0.0004294578127631808, -0.00039026103052590584, -0.0003476285707827778, -0.0003058249429885723, -0.0002671600070910888, -0.0002343581826668769, -0.00020900005958195828, -0.00019054980596271143, -0.0001773979918470673, -0.00016925239197810617, -0.00016588496465524613, -0.00016548833479338235, -0.00016551579334978146, -0.000165319202652333, -0.00016438158502175663, -0.00016068854804591332, -0.00015228770627697188, -0.00013900091737155222, -0.00012087633606610963, -9.647965896794272e-05, -6.52605838859649e-05, -2.8501290426535472e-05, 1.1299140246548087e-05, 5.1773779457146146e-05, 8.941129165612044e-05, 0.00011778600817575861, 0.0001302367976741374, 0.00012301885372871697, 9.544702246854463e-05, 4.889895892876313e-05, -1.1157888753554612e-05, -7.455380871402087e-05, -0.00012944174678540012, -0.00016688788682481769, -0.0001816447248019215, -0.0001724715863591561, -0.00014341854747669872, -0.00010497717222184011, -6.990052883895995e-05, -4.878143641363214e-05, -4.856910627587703e-05, -7.252843584162373e-05, -0.00011821358212680752, -0.0001765929198475763, -0.00023606755337511089, -0.0002859293776891914, -0.0003172411807605413, -0.00032433394428275225, -0.00030596028673975095, -0.00026583527189333843, -0.0002106996450962923, -0.00014798193943661025, -8.515168032477254e-05, -2.9283795754201855e-05, 1.4690896680097723e-05, 4.4914181156711225e-05, 6.18346305165194e-05]
  in  "3D Surface":refnum<k7>(container)
  in  "View Mode":bool caption="Scan"
  out "Hall sensors signal lf":dbl[][](graph)=[[0.019023592427, -1.240089336102, -1.360639755342, -1.299913532044, -1.209001369365, -1.121407388206, -1.040965236869, -0.965870848645, -0.895061113312, -0.830372318078, -0.763718364285, -0.704087388671, -0.653959991749, -0.602318456821, -0.555863619915, -0.516786141333, -0.476903269132, -0.439823146985, -0.410861345938, -0.374489959081, -0.350263842724, -0.318531493265, -0.297269206671, -0.275813625079, -0.253745945739, -0.232999104156, -0.219790710486, -0.2038439905, -0.191440985495, -0.172627075683, -0.159450894869, -0.151268131906, -0.139831593012, -0.133130747358, -0.11969683992, -0.112577191054, -0.10658508809, -0.097274777443, -0.093086748381, -0.085806020591, -0.081779069424, -0.072694267268, -0.071534505276, -0.064801442333, -0.062868505631, -0.060484550355, -0.055297836735, -0.051206453854, -0.045117702849, -0.045729799459, -0.037836973923, -0.03944775467, -0.033326787638, -0.038674579835, -0.033294572147, -0.031458281988, -0.026625939622, -0.026883664603, -0.026497077221, -0.023790965388, -0.025111805642, -0.021568087884, -0.024080905804, -0.020730481844, -0.018861975695, -0.017412273188, -0.019925091347, -0.014770592585, -0.016155864175, -0.01438400515, -0.013095380443, -0.012579930449, -0.013804123864, -0.013449752224, -0.010775855975, -0.011355737138, -0.013417536657, -0.010485915357, -0.013610830346, -0.008875134527, -0.009390584385, -0.009841603068, -0.010067112387, -0.014190711431, -0.001046738733, -0.008166390931, -0.00662004123, -0.009229506261, -0.006426747503, -0.007071059886, -0.009519446818, -0.006426747516, -0.006587825607, -0.004815966536, -0.006040160087, -0.006684472463, -0.010453699225, -0.008230822129, -0.00732878484, -0.004912613394, -0.005556925813, -0.005460278957, -0.005331416334, -0.009970465505, -0.003817282364, -0.003044107424, -0.003430694975, -0.004912613424, -0.003946144842, -0.007328784837, -0.005234769549, -0.006458963064, -0.000209132668, -0.004397163544, -0.001916560848, -0.005975728785, -0.002045423251, -0.004397163532, -0.002045423315, -0.00768315657, -0.003237401238, -0.005556925809, -0.003559557418, -0.002850813838, 0.000402963758, -0.002915245029, -0.003301832496, -0.002947460665, -0.00278638226, -0.005234769595, -0.000724582741, 0.002239254105, -0.002367579548, -0.002496441994, -0.001916560833, -0.00181991401, -0.005556925778, -0.001594404681, -0.002238717023, -0.004751535108, -0.004815966488, -0.002238717028, -0.006104591168, 4.8592146e-05, -0.00233536393, -0.004332732277, -0.003334048045, -0.003623988624, -0.002496442022, 0.00120835439, -1.5839306e-05, -0.000660151653, 0.000886198253, -0.00658782531, -0.000692367315, -0.003495126164, 0.000950629297, -0.001626620085, -0.006040159934, -0.006265669365, -0.001852129635, 0.00256141024, -0.004075007299, -0.002142070103, -0.002432010763, -0.002754166961, -0.001916560852, -0.00046685795, -0.002850813808, -0.000660151663, -0.002979676309, -0.002013207698, -0.001401110967, -0.002109854539, -0.00426830105, -0.00304410736, -0.001529973409, -0.001497757828, -0.002850813731, -0.001497757833, -0.00124003276, 0.002400332231, -0.002979676099, 0.001337216769, -0.003334048113, -0.000370211114, 0.001015060622, -0.000950092214, -0.000466858002, -0.002528657632, -0.002754166879, -0.000531289236, 0.00336680099, -0.000756798578, 0.000338532492, -0.002045423332, -0.003269616827, -0.000176917394, -0.000370211141, -0.003817282335, -0.001626620272, 0.000789551231, -0.002560873231, -0.005170338333, 0.003399016514, -0.002818598151, 0.000918413707, -0.002818598188, 0.000660688683, -0.00307632305, -0.001401110961, -0.005234769553, -0.000885661014, -0.003720635535, -0.002786382584, 0.00072511993, 0.001498294898, -0.003527341796, -0.001143386018, -0.0024642264, -0.005299200869, 0.000467394948, -0.001207817259, -0.001368895323, -0.003656204303, 0.005847403897, 0.000757335553, -0.005718003738, -0.003849497979, 0.000628473066, -0.00069236725, 0.000725119947, -0.000692367341, -0.00020913293, -0.002818598205, -0.002818598201, 8.0807522e-05, 0.002561410549, -0.00049907358, -0.005363632017, -0.003044107452, 0.000402963715, 1.637639e-05, -0.00352734181, -0.001143385997, -0.003237401115, -0.001272248467, 0.000435179376, 0.000950629262, -0.000176917428, -0.021278147315, 1.235166367438, 1.353752742414, 1.284617617828, 1.20530232852, 1.1214768634, 1.039391084729, 0.960559130021, 0.888975746498, 0.822418040907, 0.760338340873, 0.70122250384, 0.64374968366, 0.599839685248, 0.551709440149, 0.511955282752, 0.471685681175, 0.435571908263, 0.400778983191, 0.371881529791, 0.346044567877, 0.315697416016, 0.293178672267, 0.275137906117, 0.254519889081, 0.237348948166, 0.214959073762, 0.198464663974, 0.18197025527, 0.17153238773, 0.159064935553, 0.150366713193, 0.137641536952, 0.12324114809, 0.118118862337, 0.108550819411, 0.102204339923, 0.096469957749, 0.085194487084, 0.085001193347, 0.075755307879, 0.075529798507, 0.06696044151, 0.064061035017, 0.057456831639, 0.052173468964, 0.049725081467, 0.045150462709, 0.040028178493, 0.036967694184, 0.039319434703, 0.035131403667, 0.031201097652, 0.028237260385, 0.027270791752, 0.025563363689, 0.029397022794, 0.022953898227, 0.022148507717, 0.021761920205, 0.021761920351, 0.020505510977, 0.014771130366, 0.018250417508, 0.016961792619, 0.014835561693, 0.012741546251, 0.013579152429, 0.012322743184, 0.01145292145, 0.010873040304, 0.008489084303, 0.006749440937, 0.007973634425, 0.008972318628, 0.020151139308, 0.006491715868, 0.006556147116, 0.006588362742, 0.003463447636, 0.004011113199, 0.007168243915, 0.003817819515, 0.003882250626, 0.007973634392, 0.005331953547, 0.006137344066, 0.001433863584, 0.002593625858, 0.002368116497, 0.004687641266, 0.002947997683, 0.004268838105, 0.002174822801, 0.001143923004, 0.000241885654, 0.004075544481, 0.000660688687, 1.6376284e-05, 0.004623209934, 0.003076860204, 0.001466079161, 0.000596257439, 0.000757335776, -0.006201237808, 0.003785603856, 0.001884882274, 0.001498294796, 0.001111707336, -0.000370211077, 0.00513865994, 0.00246476336, -0.003978360414, 0.002432547781, 0.000370748137, -0.00388171345, -0.00037021114, -0.001433326567, 0.001079491715, 0.000886198121, -0.002367579519, -0.001175601632, 0.000982844965, 0.000241885638, 0.000757335534, 0.002174822789, -0.000821229802, 0.000918413686, -0.00362398861, -0.004429379072, 0.002335901012, -0.00159440457, -0.000950092291, -0.002109854581, 0.000982844855, -0.000531289252, -0.000466858012, -0.001723266993, -0.002496442, -0.002496442016, -0.00220650142, 0.002368116789, -0.001078954757, -0.002786382491, -0.007489862324, -0.001433326594, -0.000885660918, -0.005041475904, 0.004397700696, -0.000402426748, 0.001111707375, 0.001981529107, -0.002883029443, -0.001497757665, 0.000725119925, -0.000595720318, 0.001433863598, -0.003140754406, 0.000789551156, -0.001948776438, -0.001626620307, -0.003334048051, 0.001208354309, -0.002947460477, -0.000885661041, 0.003463447649, -0.001497757743, -0.001272248473, 0.001369432346, -0.005363632058, -0.003398479319, -0.001401110948, -0.007361000196, 0.004043329054, -0.00268973567, 1.6376302e-05, -0.001497757753, -0.002915245039, 8.0807617e-05, -0.002045423336, 0.000757335587, -0.003108538123, -0.001884345243, 0.000531826212, -0.007328784565, -0.002625304479, -0.001240032863, -0.002206501421, -0.003011891914, -0.002721951354, -0.002174285743, 0.001401648029, -0.002625304507, 0.001272785479, -0.001240032878, -0.002979676301, -0.004687104119, -0.001465542214, -0.001465542209, 1.6376292e-05, 0.002561410251, -0.003559557415, -0.003881713557, -0.00220650106, -0.002593088866, 0.003076860421, -0.001240032779, -0.002786382549, -0.003044107542, -0.001755482788, 0.001594941705, -0.001658835879, 0.000821766889, -0.003366263734, -0.000434642325, -0.0008212298, -0.003076323158, -0.002303148292, -0.001723267164, -0.001336679741, -0.003237401193, -0.002657520008, -0.002174285813, -0.001240032856, -0.007006628042, 0.002947997818, -0.003785066771, -0.001272248479, -0.003462910571, 0.000145238783, -0.00024134863, 0.003560094558, -0.001980992109, -0.00384949802, -0.000660151675, -0.003334048121, -0.001304464104, 0.000789551204, -0.005170338248, -0.002496442018, -0.005202553783, -0.003849497681, -0.000692367311, -0.003108538743, -0.002754166931, -0.002786382581, -0.004912613332, -0.002238717063, -0.00500926027, -0.002625304467], [0.01583424586, -1.425328478161, -1.516756053374, -1.41447185543, -1.298560480895, -1.197274923311, -1.093830905428, -0.997925297361, -0.91335953559, -0.844676016538, -0.770676921619, -0.703733017634, -0.643908739109, -0.58943223361, -0.539788054237, -0.493011053039, -0.457541711548, -0.420493802852, -0.381674033221, -0.35036048944, -0.324555807603, -0.296882619655, -0.272882006439, -0.254229179608, -0.230003053874, -0.213895256448, -0.19746530225, -0.186093196192, -0.167214854818, -0.152331246921, -0.145114951889, -0.135321408381, -0.123594928303, -0.112351681801, -0.10896904307, -0.101656100073, -0.089865187445, -0.085870451861, -0.076592356172, -0.071244564752, -0.064028267664, -0.064285992638, -0.061902037308, -0.05375148726, -0.051270885092, -0.047308364587, -0.042798178576, -0.044827762273, -0.041638416419, -0.03484092169, -0.039447754627, -0.030427382332, -0.029944148007, -0.031748222632, -0.028848817174, -0.02791456429, -0.022373478259, -0.028848817016, -0.019925091386, -0.023823181, -0.022341262675, -0.020827128636, -0.02002173814, -0.015962570467, -0.01663909842, -0.011033580875, -0.015930354828, -0.010485915039, -0.014029633409, -0.012934302411, -0.013997417804, -0.013707477154, -0.01744448863, -0.009229506238, -0.008939565645, -0.008778487567, -0.008263037689, -0.011226874506, -0.008778487661, -0.011645677629, -0.009744956198, -0.011194658993, -0.008198606528, -0.005975728857, -0.006072375431, -0.009068428238, -0.012128911894, -0.00349512595, -0.007876450276, -0.004397163547, -0.002045423137, -0.00533141645, -0.009422800026, -0.005266985227, -0.010163759081, -0.002754166916, -0.003172970021, -0.004332732289, -0.004493810364, -0.001143385966, -0.005750219535, -0.005750219297, -0.00961609376, -0.004139438595, -0.010131543521, -0.007489862862, -0.00336626366, -0.008134175265, -0.004461594788, -0.005685788259, -0.007876450339, -0.00571800392, -0.003011891789, -0.003366263705, -0.00494482898, -0.003430694846, -0.005943513145, -0.00658782541, -0.006104591327, -0.004977044557, -0.004139438578, 0.001305001231, -0.006845550453, -0.003495126174, -0.00075679847, -0.006555609836, -0.003495126125, -0.005589141318, -0.002142070099, -0.00922950619, -0.006169022524, -0.002238717057, -0.004364947916, -0.003817282372, -0.006523394249, -0.005975728783, -0.001143385833, -0.001014523524, -0.001240032865, 0.002754704343, -0.004236085363, -0.00932615295, 0.000821766976, -0.003076323148, -0.002528657488, -0.002625304429, 0.001466079178, -0.003044107524, -0.005234769599, 0.002658057198, -0.00288302938, -0.006942197319, -0.006297885026, -0.001433326563, -0.003849497972, -0.007199922294, -0.001207817179, -0.006555609878, -0.008263037555, -0.005041475872, -0.005395847709, -0.005395847684, -0.003430694924, -0.003785066737, 0.005815188357, -0.002432010714, -0.002947460587, -0.004171654208, -0.001336679608, -0.005331416433, 0.002561410541, -0.002013207728, -0.005009260272, -0.006555609918, -0.000209133029, -0.002109854576, -0.003140754361, -0.006587825628, -0.001078954732, -0.007167706612, -0.0076187254, -0.000241348429, 0.000209670021, -0.003849498023, -0.00114338598, -0.000821229818, 0.000435179464, -0.002528657535, -0.000209133029, -0.00214207017, -0.00368841986, -0.003785066684, -0.000112486116, -0.004042791729, -0.003076323148, -0.001304464086, 0.001208354238, -0.002432010745, -0.004977044527, -0.000112486146, -0.001723267116, -0.007006628521, -0.004590457193, -0.000692367295, -0.004912613389, -0.006007944381, -0.003688419896, 0.000531826287, 0.001208354231, -0.006974412924, -0.005589141378, -0.004429379132, -0.002883029419, -0.003108538709, -0.000756798563, -0.000660151492, -0.005299200725, -0.002979676308, -0.000756798448, -0.004751535293, -0.003720635545, 0.000886198123, -0.002109854597, -0.002560873171, 0.000274101241, -0.002045423337, -0.001626620268, -0.007457647292, -0.006040159924, -0.001207817244, -0.009455015596, -0.00120781723, -0.000692367337, 0.004043328855, -0.007135490928, -0.00069236728, -0.004493810379, -0.003752851151, -0.000176917382, -0.003076323164, 8.0807579e-05, -0.003108538687, -0.002303148302, -0.00362398861, -0.001529973396, 0.001079491746, -8.0270575e-05, 0.000467395007, -0.004880397786, -0.001111170374, -0.022244615487, 1.421180453883, 1.5051026997, 1.405749073783, 1.293315884603, 1.18184923562, 1.087779165259, 1.000023427189, 0.906855482273, 0.832018328264, 0.761401459629, 0.699547286946, 0.640495897497, 0.585342622398, 0.536084831264, 0.49610516685, 0.450262255867, 0.410024880772, 0.378711250946, 0.347300978449, 0.318049159122, 0.295530414968, 0.268920285118, 0.244017587485, 0.229005095445, 0.211318705969, 0.190893988012, 0.177041262271, 0.160289129745, 0.152074142294, 0.13123062551, 0.128588943409, 0.115767121119, 0.11260998912, 0.0988539143, 0.089801322278, 0.086869699806, 0.083100471296, 0.073725723377, 0.069215535391, 0.063191213206, 0.057875634746, 0.053784250249, 0.049918375223, 0.050659334659, 0.046439087874, 0.039641590951, 0.032876310408, 0.032972956899, 0.036033441088, 0.028269476108, 0.030814510127, 0.027786241652, 0.020763235976, 0.021729704649, 0.022245154672, 0.022341801416, 0.01776718317, 0.019539042381, 0.01680071452, 0.015930892745, 0.014191249212, 0.017155086459, 0.01296705561, 0.008263574987, 0.013643583697, 0.016800714596, 0.008714593701, 0.008070281284, 0.009713277906, 0.01122741226, 0.010164296604, 0.010132081084, 0.00581518784, 0.010454237204, 0.022116292076, 0.009681062313, 0.003850035167, 0.001369432386, 0.00201374471, 0.003141291394, 0.008231359553, 1.6376293e-05, 0.005589678482, -0.002238717039, 0.002110391583, -0.00046685797, 0.006749440955, 0.003044644515, 0.001079491761, 0.004526563128, 0.002722488329, 0.005042013264, -0.00346291027, -0.001046739106, -0.001626620295, 0.001240569888, -0.00291524493, 0.001691588569, 0.001627157312, 0.002947997679, 0.002754703968, -0.003946144803, 0.000274101237, -0.005846866021, -0.002657519905, 0.000499610573, -0.003140754188, -8.0270532e-05, 0.000757335668, -0.00446159468, -0.001111170408, 0.003431232106, 0.000789551216, 0.00558967864, 0.001691588611, 0.002786919577, -0.001594404665, -0.004558241601, -0.003946144725, 0.004075544433, 0.001981529096, -0.004912613265, -0.001336679677, 0.004301053819, -0.000789014043, -0.001078954751, -0.002818598188, -0.001336679743, -0.006136806859, -0.005492494572, 0.000467394985, -0.001948776437, -0.00101452353, -0.000466857972, -0.002947460655, -0.000950092285, 0.001562726062, -0.002593088875, 0.00211039176, 0.00033853256400000003, -0.002496441946, 0.0008539824, -0.004171654179, -0.00645896303, 1.6376293e-05, 0.002786919646, -0.001240032676, -0.005041475756, 0.002529194612, -0.004171654007, -0.000627936, -0.003301832475, 0.000531826274, -0.003398479296, -0.008037528393, 0.004977581758, -0.000756798558, -0.001529973447, -0.000531289232, -0.000273564208, 0.001594942162, 0.005364169546, -0.000499073623, 0.001272785502, -0.003108538627, -0.00777980337, -0.000627936033, -0.002399795171, -0.000434642383, 4.8591945e-05, -0.001465542199, -0.002818598217, -0.00107895476, 0.002142607245, -0.000434642376, -0.001594404592, -0.006007944418, 0.001176138738, -0.005846866133, -0.008295253379, -0.001014523504, 0.000306316894, -0.000950092305, -0.003462910401, -0.002883029432, -0.005943513134, 0.000467394956, -0.003913929194, 0.000950629256, -1.5838898e-05, -0.004075007319, -0.000337995521, -0.001401110947, -0.003462910467, -0.00285081381, -0.002689735718, -0.004719319722, -0.003301832422, 0.004945366217, -0.000273564275, -0.006265669166, -0.009358368757, -0.000499073609, -0.005041475885, -0.009358368788, -0.004429379127, -0.002270932658, -0.00030577989, -0.003301832461, -0.002432010756, 0.004236622741, -0.000434642352, -0.002174285793, 0.000789551281, 0.000757335826, -0.006201238027, -0.001401110916, -0.002947460678, -0.003849498008, -0.004268301019, 0.001756019834, -0.002238717076, -0.003752851107, 0.002271469711, -0.000273564244, -0.001980992037, -0.01225777437, -0.003849498007, -0.002077638973, -0.000660151373, -0.004203869732, -0.000144701808, -0.00204542324, -0.003849497963, -0.003688419882, 0.001079491973, -0.001304464102, -0.001143386011, -0.00156218908, -0.002303148251, -0.000885661008, -0.004364947701, -0.002560873235, -0.001336679743, -0.003334048044, -0.000692367236, -0.002206501458, -0.004075007336, 0.000209670042], [0.017767183157, -1.557347572873, -1.626610874127, -1.501195970196, -1.371689672172, -1.244696153819, -1.133778146403, -1.028658907289, -0.93458957034, -0.848509665605, -0.776862305559, -0.703378646582, -0.639462992642, -0.573711040411, -0.529607936096, -0.48247656253, -0.441079554351, -0.40013355913, -0.365469596842, -0.336314495589, -0.307223822948, -0.277843207225, -0.255839959194, -0.234062218707, -0.213734178577, -0.192922902963, -0.181067562734, -0.161609340244, -0.147756631086, -0.139606083743, -0.128266190734, -0.120083427318, -0.110483176586, -0.103395742926, -0.095148547327, -0.088222191265, -0.078460861586, -0.073177501434, -0.068925040717, -0.062610780813, -0.060001316204, -0.056167658295, -0.050401063438, -0.050239985363, -0.044151234412, -0.048629204648, -0.040317576266, -0.035581880875, -0.034454334306, -0.030427382367, -0.025884980317, -0.030073010503, -0.025595039917, -0.025820549234, -0.026883664578, -0.024241984018, -0.01828209491, -0.018894191628, -0.021342578521, -0.020988206756, -0.017637782421, -0.015382689372, -0.015124964375, -0.011710108938, -0.013063164869, -0.011452383385, -0.014931670692, -0.013063164889, -0.010872502868, -0.010550346602, -0.017444488869, -0.013063164882, -0.008230822124, -0.011484599599, -0.010228190495, -0.009906034312, -0.007779803295, -0.004493810316, -0.005943513235, -0.011033580909, -0.012161127394, -0.010453699795, -0.011967833825, -0.006169022423, -0.008037528426, -0.007554294056, -0.004815966518, -0.008552978292, -0.006587825594, -0.007232137939, -0.009068428223, -0.005718003919, -0.003785066752, -0.010131543553, -0.007199922348, -0.008907350102, -0.005556925756, -0.00500926029, -0.004654888426, -0.003269616856, -0.007071059712, -0.004107222808, -0.004815966393, -0.005621356955, -0.004429379113, -0.004719319672, -0.005105907094, -0.002528657625, -0.004848182193, -0.002657520098, -0.005234769518, -0.004526025969, -0.001916560834, -0.003752851133, -0.000756798559, -0.005460278954, -0.005009260246, -0.011387952359, -0.009100643344, -0.000499073412, -0.004590457137, -0.001143385816, -0.005138122737, -0.003269616821, -0.007135491049, -0.003334048069, -0.007489862845, -0.005460278884, -0.002786382573, -0.007232137836, -0.00040242675, -0.002335363912, -0.001240032811, -0.001691051516, -0.001111170317, 0.000596257784, -0.000434642223, -0.00768315628, -0.005428063176, -0.005395847579, -0.005331416449, -0.004300516647, -0.001819914017, -0.00133667972, -0.003623988557, -0.005879081953, -0.002689735718, -0.001304464007, -0.004590457218, -0.000337995267, -0.004912613437, -0.005009260243, -0.009293937357, -0.009100643354, -0.00037021095, -0.003301832394, 1.6376444e-05, -0.000789014209, 0.000596257436, -0.004558241574, -0.006233453748, -0.006394531897, -0.001723267055, -0.006297884981, -0.004751535292, -0.001272248466, -0.003591773057, 0.001756019731, -0.000499073613, -0.000917876682, -0.009906034241, -0.001433326347, -0.00433273225, -0.003913929101, -0.00446159468, -0.003044107441, -0.003978360443, -0.002142070217, -0.001980992069, -0.002786382515, -0.002303148288, -0.001787698383, -0.001465542207, -0.000789014188, -0.001658835867, -0.000982307681, -0.005589141414, -0.005428063214, -0.006974412527, -0.000305779822, -0.003140754378, 0.004172191387, -0.003044107529, 0.001788235365, -0.000337995506, -0.007071059866, 0.000950629375, -0.002560873222, 0.000209670017, -0.002915245033, -0.003398479348, -0.002850813758, -0.003849498011, -0.002464226391, -0.000917876656, 1.6376278e-05, 0.000918413798, -0.004493810344, -0.005041475899, -0.004493810326, -0.007522078431, -0.002786382471, -0.000370210981, -0.002528657608, -0.001884345239, -0.005395847692, -0.002109854557, 0.000274101322, -0.0029796763, -0.006362316247, -0.007876450258, -0.004300516658, -0.005170338365, -0.006072375668, -0.00520255401, -0.002689735733, -0.000434642042, 0.000177454504, -0.002077638961, -0.004558241524, -0.000627936072, -0.00127224846, -0.004010576062, -0.000209133056, -0.004010576104, -0.001980991999, -0.010163759124, -0.00236757947, 0.001015060631, -0.003785066733, -0.003430694957, 0.001820451154, -0.000724582973, -0.001207817235, -0.00181991394, -0.008617409196, -0.005782435088, -0.001175601542, -0.0006923673, -0.005105907083, -0.023629887299, 1.554425158807, 1.623560385771, 1.4978541357, 1.365124925156, 1.243478042613, 1.126889113748, 1.024056382486, 0.928891050565, 0.842810598067, 0.764945189029, 0.70196346543, 0.637177680593, 0.578641758236, 0.52793426267, 0.478418758102, 0.434766516403, 0.397879572996, 0.362087967895, 0.327713856832, 0.292953162578, 0.274944612111, 0.248624425161, 0.226814431482, 0.208515944797, 0.193696748831, 0.177298987353, 0.162254283629, 0.150463360447, 0.14083088501, 0.123498873318, 0.114156339419, 0.107133331723, 0.094118216538, 0.087352934255, 0.080136633372, 0.074337820178, 0.070504160474, 0.066283913283, 0.059196475415, 0.056812519175, 0.048114300192, 0.046181362701, 0.037998594312, 0.038095241036, 0.031136666396, 0.031233313283, 0.035195834945, 0.03374613197, 0.029525885214, 0.023082760742, 0.024854620047, 0.0220196452, 0.017316164447, 0.014835561656, 0.01489999289, 0.014964424115, 0.013579152406, 0.018218201843, 0.011485137039, 0.008650162678, 0.011517352722, 0.012838193124, 0.016059755425, 0.013965740025, 0.007264890896, 0.004687641216, 0.00713602842, 0.004301053745, 0.004365484962, 0.0007895512, 0.005009797336, 0.007587046944, 0.002947997698, 0.005493031658, 0.020569942235, 0.007039381529, 0.000467394976, 0.001949313474, 0.001820451138, 0.001788235452, 0.000789551467, 0.002690272858, 0.003463447596, 0.005493031665, -0.002013207682, 0.003205722663, 0.001884882242, 0.002239254034, 0.002690272695, 0.002110391565, 0.001176138608, -0.000821229764, -0.000885660992, 0.001820450971, -0.000853445369, -0.000692367274, 0.001788235372, -0.002270932681, 0.001240569813, -0.003978360228, 0.002786919587, -0.002947460663, -0.003140754332, -0.001078954763, -0.000466858004, -0.000627936119, 0.000274101373, 0.000531826222, -0.000885661055, -0.002560873043, -0.002432010774, -0.000402426744, 0.003785603829, -0.002303148245, -0.004944828945, -0.001852129602, -0.006040159967, -0.001111170394, 0.003205722677, -0.005750219492, -0.001916560846, -0.000821229632, -0.001207817116, 0.000370748114, 0.000821766847, -0.00191656082, -0.004236085407, -0.001497757785, -0.001787698318, -0.000176917407, 1.6376292e-05, 0.001143923055, -0.000821229816, 0.002658057259, -0.000853445419, -0.002270932694, -0.004977044517, -0.00191656069, -0.001433326467, 0.000628473123, -0.003398479357, -0.004654888354, -0.0036562043, 4.8591926e-05, -0.005073691529, -0.002206501423, 0.001530510488, 8.0807574e-05, -0.005428063286, 0.001176138594, -0.000499073584, -0.002464226378, -0.004493810391, -0.003559557388, 0.00410776035, -0.001562189064, -0.003334048021, -0.002818598197, 0.00272248833, -0.000756798443, -0.005331416436, -0.004558241589, -0.002721951358, -0.00159440466, -0.003591772966, -0.004526025988, 0.000241885638, 0.001498294831, -4.8054939e-05, -0.006716688078, -0.003398479308, -0.001723267, -0.008939565381, -0.001626620139, -0.002657520005, -0.001111170346, -0.003527341819, -0.003044107407, -0.001658835867, -0.00162662031, -0.000209133003, 0.000531826283, 0.000660688794, 0.002722488392, -0.002560873234, -0.007618725347, -0.003205185437, -0.003011891793, -0.000176917265, -0.00069236731, -0.003334048061, -0.002786382542, 0.002690272791, -0.000660151686, -0.006491178704, -0.004912613399, -0.002367579543, -0.003044107416, -0.001143385991, -0.00201320765, 0.000241885663, -0.003269616885, -0.001143386006, 4.8591941e-05, -0.002657520111, -0.001304464032, 0.00056404214, -0.000917876633, -0.003205185584, -0.005846866338, -0.004622672735, -0.000466857989, -0.004010576034, 0.000499610629, -0.000595720453, -0.002689735632, -0.000337995529, 0.002529194635, -0.00365620425, -0.007747587855, -0.002754166955, -0.004171654146, -0.004364947852, -0.003656204256, -4.8054914e-05, 0.000725120025, -0.000853445359, -0.002399795148, -0.00101452353, -0.000337995501, -0.000305779896, -0.002109854594, -0.000821229798, -0.004010576069, -0.004783750853, -0.006169022494, 0.001466079216, -0.002625304502, 0.000274101249, -0.004139438485, -0.00114338598, -0.00024134846, -0.000337995428, -0.004010576039, -0.010808071469, -0.003172969992, -0.000821229806, -0.00359177293, -0.00111117038], [0.018830298789, -1.652383263437, -1.714333640582, -1.562695344243, -1.41576047536, -1.282484943572, -1.156651161861, -1.052949410855, -0.948152308163, -0.859269654705, -0.779020747132, -0.705891459377, -0.637143472797, -0.581990439336, -0.519846620026, -0.471845424735, -0.445009854088, -0.387988286202, -0.351971268505, -0.32542562832, -0.290632795721, -0.267437571799, -0.244467855275, -0.222851191976, -0.202104348285, -0.179327920386, -0.169341084483, -0.154682985865, -0.142602134913, -0.125237924071, -0.118182706513, -0.107519340742, -0.106456225543, -0.093698844816, -0.086385901624, -0.076076906321, -0.069408274852, -0.058970416554, -0.061998683735, -0.056554245568, -0.050239985403, -0.064124914495, -0.043829078236, -0.042830394207, -0.039093382847, -0.040414223089, -0.035034215326, -0.028913248311, -0.029460913891, -0.027527976915, -0.023307731175, -0.023597671726, -0.020215031872, -0.016252510997, -0.023629887034, -0.019764013242, -0.01628472657, -0.01531825811, -0.016155864183, -0.014899455027, -0.013127596121, -0.014448436432, -0.011387952723, -0.01522161104, -0.006201238109, -0.009422800008, -0.024080905866, -0.011226874619, -0.009809387424, -0.012612146138, -0.009455015634, -0.004526025616, -0.004236085254, -0.009680524978, -0.007038844195, -0.011581246335, -0.006942197344, -0.008391900151, -0.00826303774, -0.005943513205, -0.011871186912, -0.008295253347, -0.010582562243, -0.005170338384, -0.003752851132, -0.007264353592, -0.005750219484, -0.002947460495, -0.004912613012, -0.006781118993, -0.005685788189, -0.019506288146, -0.006040160036, -0.006297884988, -0.006942197373, -0.003591773058, -0.001078954727, -0.002206501445, -0.002625304484, 0.000950629273, -0.002689735711, -0.001594404667, -0.004912613401, -0.006716688016, -0.005653572662, -0.004042791638, -0.002174285774, -0.005041475902, -0.001562188887, -0.003527341823, -0.004526026016, -0.005911297369, -0.004364947835, -0.008810703104, -0.003913929226, -0.004042791673, -0.017283410625, -0.002947460667, -0.003172970026, -0.007232137805, -0.007618725297, -0.004075007318, -0.003913929225, -4.8054742e-05, 0.003399016531, -0.008230822061, -0.005556925644, -0.004461594713, -0.004526025999, -0.003495126167, -0.004429378936, -0.004880397781, -0.005299200828, -0.002464226371, -0.005556925769, -0.003495126169, -0.003849497889, -0.001014523402, -0.004364947763, -0.001787698295, -0.003849497877, -0.014899454823, -0.000112486146, -0.00172326705, -0.000821229793, -0.002786382567, -0.002142070186, -0.002786382579, -0.004139438556, -0.000305779888, -0.003076323154, -0.003334048108, -0.005460278907, -0.00413943852, -0.003495126109, -0.001175601407, -0.00162662028, -0.003430694942, 0.000402963996, -4.8054934e-05, -0.003688419928, -0.001852129487, -0.004912613439, -0.004977044631, -0.000112486165, -0.001884345244, -0.017347841706, -0.003462910567, -0.001819913987, -0.002560873227, -0.003752851129, -0.000853445379, 0.000467394988, -0.005331416358, -0.002013207699, -0.002335363921, -0.003591773066, -0.001884345234, -0.003269616739, -0.001240032866, -0.00220650134, 0.001723804291, -0.004139438434, -0.000692367233, -0.001240032754, -0.006748903659, -0.00436494789, -0.002013207714, -0.001691051452, 0.000274101259, -0.003495125992, -0.018668682225, -0.003656204282, 0.002207038537, -0.001433326552, -0.002915244946, 4.8591991e-05, -0.005750219267, -0.001819913977, -0.001046739159, -0.004880397819, -0.005073691429, -0.005911297555, 0.000370748103, 0.0020137447, -0.002045423278, -0.001691051551, 0.000531826271, -0.002303148279, -0.003172970036, -0.003140754367, -0.001852129583, -0.003076323072, -0.010453699221, -0.001046739128, -0.002947460681, -0.012708792985, -0.000853445361, -0.00529920065, -0.000917876642, -0.00362398863, -0.002528657614, -0.005202553941, -0.001787698358, -0.002657520119, -0.002013207745, -0.003623988679, -0.001497757795, 0.002303685366, -0.001465542182, -0.000885660896, -0.000982307882, -0.000273564274, -0.007135490995, -0.00217428573, -0.003495126172, -0.003752851148, -0.002818598192, -0.002270932629, 0.002915782081, 0.000370748197, -0.014641730032, -0.00091787664, -0.000499073594, -0.00297967626, -0.000209132966, -0.003172970019, -0.004107222968, -0.006748903327, 0.000725119912, -0.023146653033, 1.651620404158, 1.708513635483, 1.562511337269, 1.416702454025, 1.278754341768, 1.16049017106, 1.046704062761, 0.943291488919, 0.853087416707, 0.770357429962, 0.701641308153, 0.632989639029, 0.573326168981, 0.522232086198, 0.472201132002, 0.413665251292, 0.38415569862, 0.351650092892, 0.318339099998, 0.286091228309, 0.262283860884, 0.237059007334, 0.215377877156, 0.199366701973, 0.182904508854, 0.166828904347, 0.15194527947, 0.13396895434, 0.12304785423, 0.118537665634, 0.104910453013, 0.094343725976, 0.086773052906, 0.075078779778, 0.065639601247, 0.065027503846, 0.068184635718, 0.053590956623, 0.054782934653, 0.049274062861, 0.031362175924, 0.037128772355, 0.036355597359, 0.030621216414, 0.032103135056, 0.02843055403, 0.025176776203, 0.02189078285, 0.023308270139, 0.024886835621, 0.020859882798, 0.021922998576, 0.019442395481, 0.016865145751, 0.009938787771, 0.015254364657, 0.009584415525, 0.009906571621, 0.009842140421, 0.008199143726, 0.009584415444, 0.007522615756, 0.007393753327, 0.010840824671, 0.011227412164, -0.005653572506, 0.00397889754, 0.004880934871, 0.006878303289, 0.004945366087, 0.004365484999, 0.010196512465, 0.003431231985, 0.0068460878, 0.019120239257, 0.004655425507, 0.001433863559, -0.000627936105, 0.001627157258, 0.001079491733, 0.00291578204, -0.000144701762, 0.000886198105, 0.000692904302, 0.002980213305, 0.003302369497, 0.002658057139, 0.001111707501, 0.006395069381, 0.005718541135, -0.01470616117, 0.001240569852, -0.000821229801, 0.000918413693, -0.002077638904, -0.000563504846, 0.004945366105, -0.003301832483, -0.003301832446, -0.000241348661, 0.001240569864, 0.001756019781, -0.000273564285, -0.006233453565, -0.001594404665, -0.000144701726, -0.004075007307, 0.000628473221, 0.003527878905, -0.000499073579, -0.001916560798, 0.001562726102, -0.000144701742, 0.000789551271, -0.002206501415, -0.011903402312, -0.000466858016, -0.004815966398, -0.00146554219, -0.001401110966, -0.001948776469, -0.00066015171, -0.000531289253, 0.001240569964, 0.000338532516, -0.003913929122, -0.005460278764, -0.002432010721, -0.001884345162, -0.002077638966, -0.001594404621, 0.000725119921, -0.002206501433, -0.000982307896, -0.002238717045, -0.003140754369, -0.00059572045, -0.004590457205, 0.000660688732, -0.001175601586, -0.015028317323, -0.006040159942, 0.003076860424, 0.0033668011, 0.000145238777, -0.000950092224, -0.002689735705, 0.000241885636, -0.002270932687, -0.003237401234, -0.002625304493, -0.000950092257, -0.00265752008, -0.001658835823, -0.002818598188, -0.002689735682, -0.002432010751, 0.000725119967, -0.000337995522, 0.002625841925, -0.007296568849, -0.003398479309, -0.002045423253, 0.000338532629, -0.003011891906, -0.014835023713, 0.002207038422, -0.001433326591, -0.003140754368, -0.003817282338, 0.00085398251, 0.001530510418, 0.001401647954, 4.8591924e-05, -0.004429379104, -0.005041475862, -0.003656204233, -0.002109854565, -0.000917876611, 0.002722488382, -0.001111170376, 0.00278691959, -0.001852129545, -0.001819913975, -0.003076323129, -0.004622672792, -0.003913929269, -0.003656204146, 0.002786919617, -0.001014523478, -0.01154903063, 4.8591949e-05, 0.000564041833, -0.002432010773, 0.000821766962, 0.004913151022, -0.004429379071, -0.00384949777, -0.005428063154, -0.002496441992, -0.005718003793, -0.001240032877, -8.0270489e-05, -0.000337995502, 0.000338532495, -0.002367579533, -0.002915245062, -0.000595720394, -0.000337995487, -0.004010576045, -0.004461594713, -0.005814650527, -0.005009260091, 0.003334585191, -0.001207817202, -0.007361000042, 0.000145238793, -0.002689735704, -0.001980992033, -0.000563504855, -0.001980992083, -0.000789014186, -0.001980992054, -0.000144701825, -0.0001124862, -0.004461594696, 8.0807615e-05, 0.002851350873, -0.001240032848, -0.001465542139, -0.001948776488, -0.002496441969, -0.01019597465, 0.001079491726, -0.006201237943, -0.00194877634, -0.001497757785, -0.002528657485, 0.00120835436, -0.001529973446, -0.015930354743, -0.001723267165, 0.001143923096, -0.000499073579, -0.003752851135, -0.002335363907, -0.00181991398, -0.002399795069, -0.005492494558], [0.010969687155, -1.713560468962, -1.764750870322, -1.610728638707, -1.446268551246, -1.308096270275, -1.176077116303, -1.064546998367, -0.95775253564, -0.862007975129, -0.786237028385, -0.703733017599, -0.636692455011, -0.576094991987, -0.519943266737, -0.47332734059, -0.424971767716, -0.38425127943, -0.349426237515, -0.31753281021, -0.282965485782, -0.263732778758, -0.235898507601, -0.210738128112, -0.193921586593, -0.17836145244, -0.159160954547, -0.146113635646, -0.139058418071, -0.125076846147, -0.108292515258, -0.094053216266, -0.092184711334, -0.085967098699, -0.076978943444, -0.072049955051, -0.061193293736, -0.062707427622, -0.050497710274, -0.051045375784, -0.044473390522, -0.040607516774, -0.039641048307, -0.035646312005, -0.03745038641, -0.028558876597, -0.028494445413, -0.026013842947, -0.024886296371, -0.025659471081, -0.020794913069, -0.022147968958, -0.019538503974, -0.023211084213, -0.018378741699, -0.012064480396, -0.00884291866, -0.016381373469, -0.014351789573, -0.010904718356, -0.012418852481, -0.008585193849, -0.014061849, -0.013932986509, -0.008230822135, -0.013610830378, -0.007908665968, -0.008295253402, -0.009873818677, -0.008359684608, -0.011033580847, -0.009616093678, -0.012579930423, -0.00481596653, -0.006716688065, -0.007973097136, -0.005138122753, -0.002689735696, -0.008649624875, -0.002270932573, -0.006877766156, -0.000370210931, -0.004268300919, -0.007522078501, -0.004300516496, -0.011098011964, -0.000853445389, -0.005234769566, -0.002496441877, -0.003978360488, -0.007328784792, -0.004654888432, -0.003044107508, -0.008649624972, -0.00210985457, -0.00114338584, -0.005073691536, -0.003495126155, -0.00581465074, -0.001787698384, -0.007489862771, -0.001723267133, -0.005653572641, -0.005170338372, -0.004429379122, -0.003527341764, 0.001562726285, -0.005170338373, -0.004880397752, 0.000853982479, -0.002238717035, -0.003785066735, -0.004622672837, -0.002850813798, -0.002464226395, -0.001819913991, -0.007199922242, -0.002270932685, -0.005105907116, -0.002947460615, -0.000273564269, -0.001046739087, -0.00504147588, -0.000563504855, 0.001723804448, -0.003591773063, -0.004815966562, -0.003752851081, -0.006781119307, -0.00088566106, -0.000112486158, -0.002174285367, -0.003946144794, -0.001304464058, -8.0270446e-05, 0.000177454459, -0.00178769836, -0.002399795126, -0.002206501439, -0.00288302943, -0.003495126209, -0.003140754395, -0.000402426722, -0.000789014183, -0.003978360464, -0.004364947924, -0.001819913974, -0.006813334891, -0.001207817252, -0.000756798582, -0.006330100549, -0.003495126144, -0.001014523449, -0.002850813786, 0.002078175998, -0.000724582947, 0.003978897805, -0.005138122593, -0.002625304373, -0.000144701725, -0.001594404677, -0.001980992108, -0.0005312892, -0.005202554004, -0.001207817248, -0.007071059458, -0.004590457241, -0.002367579532, -0.003237401241, 4.859193e-05, -0.000789014185, -0.00059572042, -0.005105907063, -0.002496442003, -0.002464226256, -0.000821229793, 0.001820451048, -0.003720635544, -0.00330183244, -0.002109854539, 0.00011302321, -0.00114338566, 0.001756019783, -0.002947460656, -0.000144701748, -0.002818598196, 0.002496979051, -0.00217428583, -0.00594351314, -0.002013207646, -0.005266985231, -0.006072375518, -0.000370211066, -0.000627936096, -0.003366263715, -0.001272248437, -0.000209132946, -0.001497757762, -0.001658835918, -0.003785066486, -0.002432010786, -0.000756798446, -0.003076323126, -0.003752851065, -0.000917876423, -0.003011891876, -0.005589140478, -0.004042791682, -0.001852129562, 0.001015060549, -0.002593088882, 0.000435179513, -0.003559557403, 0.000306316888, -8.027053e-05, -0.005750219435, -0.000176917095, -0.004203869831, -0.00095009226, -0.002206501428, 0.000628473079, -0.002496441839, -0.00536363185, -0.000241348562, -0.001948776467, -0.001240032747, -0.002947460671, -0.001948776502, -0.003720635494, -0.000982307908, -0.00066015172, 0.000274101575, -0.000466857914, -0.001014523484, -0.00072458293, -0.002496442024, -0.001497757775, -0.005041475873, -0.00568578821, 0.00162715755, 0.000853982531, -0.002077638921, -0.001852129504, -0.003559557426, -0.003462910574, 0.00056404183, -0.000144701646, -0.00581465074, -0.000370211071, -0.005363632017, -0.023790965415, 1.70722500023, 1.761476547076, 1.603425472925, 1.447533001311, 1.305622322076, 1.179497483851, 1.062360924535, 0.954695863752, 0.866779103884, 0.775962965336, 0.702704426761, 0.632860776241, 0.570587834987, 0.514049302175, 0.464823741727, 0.41943185627, 0.379935446316, 0.343499530431, 0.313281241746, 0.28264415337, 0.252941322239, 0.229971564967, 0.213702663871, 0.194051121146, 0.168149745612, 0.158936072874, 0.145856524037, 0.127268102395, 0.120019584715, 0.108003153612, 0.099304933353, 0.08867377509, 0.084646821552, 0.077140579967, 0.06979541693, 0.062385822443, 0.05813335974, 0.052495625216, 0.047244478337, 0.041767822325, 0.04096243183, 0.038224103574, 0.035066972457, 0.031040019501, 0.029332591468, 0.023114976441, 0.024403601231, 0.025660010725, 0.021214254665, 0.015189933502, 0.016639636433, 0.017316164452, 0.01225831203, 0.011485137013, 0.013063702477, 0.014223465066, 0.008199143743, 0.012065018301, 0.008263575219, 0.004462131855, 0.008489084445, 0.005654109794, 0.003978897536, 0.008907887376, 0.004462131819, 0.004623209886, 0.007812556282, 0.003302369546, 0.003527878866, 0.007007165823, 0.005428600399, 0.000789551402, 0.003302369472, 0.004494347399, 0.014964424126, 0.006266206615, 0.003721172528, 0.002786919594, 0.000950629248, 0.001079491736, 0.007103813032, 0.004752072435, -0.000176917414, 0.005686325524, -0.000692367158, 0.003592310108, -0.004622672603, -4.8054925e-05, 0.000628473049, -1.5839313e-05, -0.001916560865, 0.001015060498, -0.001787698362, -0.00075679858, 0.004075544488, -0.002850813816, -0.001078954774, 0.001079491741, 0.001884882357, -0.004364947698, -0.000756798557, 0.004590994322, -0.002142070204, -0.001658835927, 0.000145238797, 0.001627157582, 0.001047276155, -0.001304463941, -0.002174285677, 0.003205722735, 0.002078176051, -0.00504147568, 0.00136943232, -0.002367579503, 0.001917097856, -0.005975728685, 0.002658057103, -0.001304464105, -0.005105907008, 0.001401647957, -8.0270539e-05, -0.005428063315, -0.000853445423, -0.000756798584, -0.002560873211, -0.000370211132, -4.8054852e-05, 0.002174822866, -0.004526025899, 0.000209670013, 0.003366801149, -0.000660151692, 0.000950629321, -0.005266984897, -0.00484818218, 0.002980213434, 0.00027410126, -0.001819914019, 0.000113023163, -0.002689735698, -0.003172969974, -0.002915244963, -0.003849497986, -0.006781119159, -0.001175601621, -0.002883029417, -0.00172326715, 0.001015060489, -0.000563504667, -0.001755482642, 0.00172380443, -0.0026253045, -0.000692367316, -0.000595720328, -0.002303148279, 0.001305001468, -0.008971780833, -0.001529973363, -0.001143385921, 0.000628473134, -0.002142070141, -0.001658835893, -0.000466857991, -0.002560873252, -0.006136806917, -0.004719319704, 0.001852666706, -0.000563504831, -0.003398479325, 0.001433863673, 0.000950629257, -0.005041475835, 0.00136943231, 0.000499610601, -0.003527341816, -0.002303148293, -0.004300516624, -0.001884345185, -0.000337995483, -0.004526025974, 0.000241886192, -0.000821229789, -0.001014523512, -0.004751535163, 0.001466079502, 0.001820451125, -0.002174285729, -0.004429379133, 0.001176138612, -0.00736100043, -0.004687104052, -0.001078954765, 0.000660688678, -0.001884345176, -0.000917876679, -0.003656204161, -0.002979676317, -0.001240032889, -0.003559557393, -0.00536363209, 0.003270154063, -0.000756798526, -0.004075007127, -0.002560873214, 0.000306316892, 0.00281913567, -0.000273564267, -0.001626620257, 0.001691588633, -0.003495126174, 0.001981529338, -0.006233453783, -0.003366263702, -0.00024134867, -0.001787698411, -0.00636231622, -0.002367579539, -0.000627936088, 0.001111707658, -0.00017691735, 0.001691588531, -0.00629788488, -0.002367579522, -0.005460278946, -0.006136806954, 0.000628473174, -0.002657520091, -0.001111170367, -0.001336679735, -0.000434642287, 0.000564042618, -0.003623988661, -0.001143385916, 0.003785603895, -0.004783750926, 0.002915782332, -0.005911297579, -0.001240032823, -0.001852129609, -0.00156218904, -0.001626620297, -0.000789014175, 0.001208354547, -0.003656204281, -0.006330100597, -0.003044107423, -0.003269616861, -0.001497757809, -0.001433326588], [0.018024908132, -1.747676665083, -1.789814514225, -1.634632530414, -1.469914725205, -1.327200064007, -1.19044523491, -1.070829024682, -0.968061504527, -0.87154377359, -0.779890566795, -0.711303671442, -0.634566228341, -0.572196909277, -0.51849356629, -0.469332610186, -0.419430688861, -0.383993554777, -0.344948271729, -0.307868134643, -0.286219259986, -0.254680197907, -0.228875508164, -0.208579683135, -0.183612594702, -0.166022877496, -0.157936761677, -0.133807274894, -0.131004517417, -0.117570610009, -0.106069638423, -0.09537405658, -0.090058481075, -0.084517396316, -0.075335947338, -0.062997368109, -0.06122550946, -0.05442801506, -0.053139390677, -0.048693635948, -0.040929672971, -0.037611464619, -0.037547033333, -0.036419486767, -0.028977679628, -0.029847501282, -0.029976363722, -0.022856712531, -0.024531924484, -0.020021737933, -0.021181500486, -0.020279463162, -0.009068428109, -0.014802808223, -0.015608198599, -0.013095380471, -0.015672629878, -0.010163759198, -0.013804124098, -0.006104591265, -0.009551662455, -0.010679209128, -0.011967833844, -0.009326153116, -0.010840287145, -0.007296569174, -0.009938249806, -0.004397163286, -0.008520762729, -0.007618725364, -0.00700662864, -0.009293937472, -0.006942197316, -0.008875134505, -0.00336626328, -0.006974413012, -0.007844234663, -0.003301832305, -0.005975728811, -0.006394531878, -0.001755482776, -0.005556925777, -0.002560873217, -0.006330100618, -0.003495126146, -0.004622672879, -0.004526025947, -0.002947460634, -0.004880397815, -0.004203869799, -0.003527341807, -0.004300516652, -0.003495126104, 0.001659373053, -0.003785066769, -0.006104591232, -0.007071059874, -0.0023031483, -0.007908665882, -0.005363631754, -0.004268301032, 0.00136943261, 0.006201775501, -0.006813334954, -0.004880397666, -0.004783750906, -0.002560873207, -0.001691051493, -0.004912613447, -0.001980992064, -0.000660151617, -0.006104591252, -0.004526026018, -0.001465542181, -0.00330183236, -0.002947460672, -0.003527341776, -0.003495126105, 0.000209670015, -0.004107222961, -0.002206501417, -0.006072375579, -0.001272248395, -0.002560873226, -0.000337995127, -0.004880397826, -0.004397163496, 0.002851351036, -0.001433326536, -0.001626619872, -0.005105907139, -0.001787698409, -0.002399795153, -0.003462910594, 0.000306316895, 0.003076860302, -0.00636231618, -0.003269616863, -0.000434642328, -0.006587825532, -0.002109854609, 0.001079491747, -0.0018843452, -0.001626620307, -0.000660151581, -0.004944829039, -0.003623988661, -0.001884345233, -0.002818598192, -0.001852129256, -0.001852129577, -0.005202553892, 0.004139975767, -0.002883029246, -0.003623988619, -0.006909981635, -0.003205185602, -0.000241348606, -0.003752851169, -0.001658835915, -0.003044107514, -0.002979676298, -1.5839145e-05, -0.000692367287, -4.8054803e-05, -0.003205185619, -0.002399795054, -0.007167706634, -0.001980992066, -0.00165883591, -0.008971781118, -0.006362316263, 8.0807675e-05, -0.005524710049, -0.005975728513, -0.002754166925, -0.001787698332, 0.003882250917, -0.000692367314, -0.002174285765, -0.000627936104, 0.00033853291, -0.000402426725, -0.003076323123, -0.005685788292, 0.000435179405, -0.002657520052, 0.001272785578, -0.000756798532, -0.001401110958, -0.00046685798, 0.000499610639, -0.003656204258, -0.002850813828, 0.000950629234, -0.00278638251, -0.008069744009, -0.003108538753, -0.005718003634, -0.001401110502, -0.002045423346, 0.000145238957, 0.003592310253, 0.000596257488, -0.000241348302, -0.006587825579, -0.001980992059, -0.001819913891, -0.002528657556, -0.002206501386, -0.001207817204, -0.00259308888, -0.003720635541, -1.5839248e-05, -0.004236085353, 0.001691588931, 0.004011113453, -0.00288302942, -0.000531289201, -0.001175601583, -0.006104591217, -0.003205185641, -0.001787698389, -0.001046739162, -0.003559557068, -0.000724582891, -0.001111170338, 0.005299738137, 0.00130500129, -0.000982307864, -0.003366263562, -0.004139438507, -0.001916560756, -0.002174285766, -0.000821229799, -0.000531289176, -0.001368895353, 0.002078176042, -0.003978360495, -0.003591773035, -0.00233536391, -0.000144701698, -0.004429379044, -0.002303148172, 0.00043517935, -8.0270392e-05, -0.002045423338, -0.001884345249, -0.003011891889, -0.002174285346, -0.022341262689, 1.741180538844, 1.79800936827, 1.629198161689, 1.463479838211, 1.314642748194, 1.190708576832, 1.071606849425, 0.962556506461, 0.86665024086, 0.782792698432, 0.70334874077, 0.632345325045, 0.570233462325, 0.515305713969, 0.463084095387, 0.416081426474, 0.373170156572, 0.336734241621, 0.306419306721, 0.272947241618, 0.248785503483, 0.226975509713, 0.206454143573, 0.183903194172, 0.168085314247, 0.151204319758, 0.142216157319, 0.123112285537, 0.114542927098, 0.102784221305, 0.093699413364, 0.089382519004, 0.075336504702, 0.072694823179, 0.060485100488, 0.057907850431, 0.051883528433, 0.052721134601, 0.0410268628, 0.034358229004, 0.03464816928, 0.034293797466, 0.032393075651, 0.026497616684, 0.026626479269, 0.022921682709, 0.027657379385, 0.018024908108, 0.014545621723, 0.01825041751, 0.012258312006, 0.016381911713, 0.010325374718, 0.012065018243, 0.009004534275, 0.010550884035, 0.015028855837, 0.007554831367, 0.005299737991, 0.00594405037, 0.004687641188, 0.001176138685, 0.00391446626, 0.000531826377, 0.004043328765, 0.008070281299, 0.003237938343, 0.005106444216, 0.00655614717, 0.005074228627, -0.001240032859, 0.002368116573, 0.0013372169, -0.001111170237, 0.014416758825, 0.001659372901, 0.009842140545, 0.001820451013, 0.001756019875, -0.000370211114, 0.001143923084, 0.005170875478, -0.001658835854, 0.004172191308, -0.001755482772, 0.001949313475, 0.000918413711, 0.000789551185, 0.000692904311, -0.003495126161, -0.001723267117, 0.000338532612, 0.001433863621, 0.005009797536, -0.000627936045, -0.002818598168, 0.003205722683, -0.003688419463, -0.00246422599, -0.001465542204, -0.002689735686, 0.004107760222, 0.003334585154, -0.00314075435, -0.001401110946, 0.000306316891, 0.003366800809, -0.004300516665, -0.001111170327, -0.001819914002, -0.002045423319, -0.005556925635, 0.002078176006, 0.001015060541, -0.001240032881, -0.000370211148, -0.00059572044, 0.001594941703, 0.000402963793, -0.003398479237, -0.006072375448, -0.003462910585, -0.003205185638, -0.004397163018, 0.000660688669, -0.007586509663, 0.00449434755, -0.00043464238, 0.000725120223, -0.005879081942, 0.004107760109, -8.027047e-05, 0.0005318262, -0.000917876672, -0.000660151714, -0.000563504849, -0.001562189002, 0.001659373028, -0.00626566921, -0.005395847638, -0.003398479284, 0.000467394978, 0.0008539824, 0.001917097968, -0.001368895338, -0.003752851144, -0.000756798566, -0.002754166799, -0.002496441752, -0.003623988681, -0.00404279169, 0.00401111329, -0.002174285795, -0.000176917265, -0.00500926002, -0.00359177293, -0.000982307738, -0.000176917371, -0.005492494436, -0.004300516676, -0.004236085422, -0.002915245021, -0.001755482756, -0.003108538786, -0.001014523459, -0.000209133036, -0.00662004083, -0.001078954776, -0.000982307854, -0.002109854535, -0.004300516668, 0.000274101258, 0.002303685332, -0.004042791423, -0.001852129581, -0.004075007243, 0.006556147215, -0.002077638958, -0.001078954755, -0.000112486195, -0.005299200757, 0.001079491752, -0.005492494548, -0.001529973429, -0.001884345201, -0.002496441993, -0.00146554208, 0.000628473151, -0.003205185597, 0.001949313824, -0.00075679856, 0.000209670102, -0.000595720394, -0.001819913988, -0.004558241503, -0.00491261334, 0.000660688699, -0.001046739016, -0.004332731908, -0.001465542186, -0.005975728786, 0.00265805728, -0.002270932643, -0.000982307891, -0.00297967622, -0.001562188886, -0.000434642301, -0.008714055773, -0.003946144854, -0.001304463908, -0.004977044538, -0.002754166929, 0.001820451035, -0.003495126177, -0.002689735692, -0.002754166958, -4.805493e-05, 0.000499610568, -0.002721951316, -0.001433326573, -0.004526025915, -0.000531289214, -0.003430694767, -0.002915244587, 0.000918413946, -0.003785066771, 0.002142607485, 0.001047276125, -0.004977044644, -0.00362398866, -0.002528657643, -0.000885660985, -0.001980992071, 0.001208354306, 0.002464763683, -0.005685788174, -0.002593088868, -0.002657520051, -0.006169022559, -0.003752851049, -0.003334048117, -0.007618724967, -0.002850813812, 0.004397700577, -0.002721951265, -0.004236085356, -0.002367579472, 0.000435179356, -0.001594404421], [0.016736283259, -1.776026288653, -1.822513226019, -1.652576556417, -1.484347266862, -1.335608310309, -1.199272285001, -1.077594283891, -0.978853705811, -0.876955983428, -0.784497389221, -0.707598883428, -0.640300597066, -0.570296191185, -0.514305542748, -0.469461472587, -0.419108533172, -0.37684169621, -0.341275695307, -0.307578194368, -0.292243575015, -0.249686781207, -0.228198980687, -0.201331173902, -0.187703976141, -0.16415437244, -0.150462742022, -0.137963087969, -0.124947983731, -0.114574558646, -0.105135385745, -0.091540398952, -0.082777752992, -0.07865415521, -0.07198552381, -0.06370611157, -0.058841554131, -0.054041427809, -0.049112438969, -0.043120334722, -0.045826446263, -0.0390611673, -0.041638416153, -0.029621991866, -0.031039479031, -0.038062483131, -0.025240668038, -0.025015158792, -0.022309047013, -0.020730481727, -0.022760065619, -0.013836339596, -0.016027001704, -0.012322205581, -0.014448436412, -0.018443172861, -0.015092748794, -0.01766999811, -0.011806755716, -0.012000049489, -0.008810703153, -0.007940881577, -0.008778487647, -0.0071032755, -0.004751535338, -0.008810703148, -0.006909981669, -0.013385320878, -0.007812019066, -0.006620041179, -0.019377425835, -0.008714056394, -0.006877766189, -0.008585193883, -0.0057502193, -0.003946144733, -0.005589141416, -0.009229506256, -0.005846866368, -0.00639453189, -0.011838971254, -0.005170338392, -0.001014523493, -0.008391900209, -0.006233453789, 0.00088619823, -0.003495126198, -0.00703884418, -0.007361000442, -0.003269616751, -0.002850813821, -0.003785066752, -0.010614777761, -0.007361000343, -0.007908665925, -0.017992153514, -0.003495126197, -0.005621356919, -0.005750219508, -0.005105906957, 1.637633e-05, -8.0270515e-05, -0.005073691444, -0.001884345221, -0.002077638977, -0.002528657624, -0.004526025963, -0.00268973567, -0.002399795112, -0.003881713569, -0.002013207638, -0.000917876629, -0.00607237556, -0.005492494569, 0.000402963747, -0.003817282349, -0.001755482763, -0.002786382354, -0.003108538665, -0.001787698376, -0.013804123979, -0.003301832437, 0.001272785498, -0.006426747526, -0.004815966427, -0.002560873265, -0.000627936089, -0.004848182134, -0.006781119271, 0.000596257578, -0.003269616826, -0.003881713579, -0.00465488842, -0.004558241629, -0.001207817082, -0.005299200804, -0.000789014148, -0.00539584767, -0.001691051542, -0.002464226338, -0.001562189049, -0.001916560823, -0.00352734158, -0.001529973287, -0.003623988594, -0.012000049367, -0.000692367259, 0.000467394966, -0.000789014177, -0.003591773011, -0.001658835895, -0.00043464233, -0.006458962943, -0.005718003908, 0.000306316862, -0.003656204264, -0.000627936037, -0.000337995473, -0.001111170204, -0.006136806929, -0.000241348635, -0.000241348643, -0.002850813753, -0.000434642334, 0.003914466299, -0.004526025985, -0.002496441999, -0.012966517643, -0.004075007232, -0.000337995529, -0.01393298637, -0.004300516587, -0.001465542189, -0.001046739112, -0.007457647113, -0.001852129591, -0.000950092287, -0.004558241551, -0.008939565643, -0.001014523494, -0.00497704464, -0.001401110966, -0.003817282323, -0.001723267147, 0.0027224884, 0.0015949418, -0.003334047407, -0.001014523538, -0.002206501452, 0.001176138659, -0.000370211136, 0.003656741488, -0.010936933443, -0.00629788465, 0.002174822852, -0.007876450193, -0.002657520046, 0.000209670019, -0.00346291047, -0.002335363827, -0.000241348632, 0.002271469716, -0.005492494559, -0.000724582955, 0.000435179469, 0.000370748098, -0.002303148278, -0.000370211007, 1.6376393e-05, 0.003109075916, 0.001917098083, 0.004204406919, -0.005943513114, -0.003366263732, -0.003237401145, -0.003011891903, -0.001014523519, -0.003076323027, 0.000274101328, -0.002013207671, -0.012676577289, -0.003011891892, -0.000305779897, -0.003011891908, -0.005782435093, -0.002528657547, 0.005267522692, -0.005589141328, -0.004622672882, -0.002593088824, -0.001980992101, -0.00049907352, -0.002721951186, -0.000402426516, -0.005589141367, -0.003623988449, -0.003849497957, -0.003430694946, 0.001240569832, 0.002819135209, -0.001143385962, -0.002432010688, -0.00468710389, -0.004171653992, -0.000660151668, -0.012289989848, -0.005782434952, -0.004815966529, -0.001562189003, -0.005879081953, -0.020794913047, 1.771914495127, 1.817242258522, 1.647625636528, 1.483389224317, 1.331233889502, 1.197022871079, 1.074989504908, 0.969289598624, 0.873383329659, 0.786690801016, 0.701705739801, 0.629864716137, 0.573132874922, 0.516787635385, 0.459347076608, 0.418175445159, 0.369723080362, 0.337894005425, 0.301715820945, 0.266053092273, 0.246337114126, 0.218921598183, 0.207162888179, 0.180971570415, 0.163736202971, 0.146565268075, 0.13406560126, 0.122822344824, 0.111031423048, 0.100561342738, 0.091251025452, 0.082037355442, 0.07159949187, 0.065381875786, 0.063223428987, 0.05839108479, 0.048726397148, 0.046471303307, 0.047405556491, 0.038030809818, 0.035099188023, 0.028301691692, 0.026755341822, 0.026723126079, 0.015125502464, 0.01944239545, 0.020344432862, 0.019506826742, 0.015383227201, 0.012193880774, 0.017896045832, 0.008102496851, 0.008521300043, 0.012773761871, 0.006974950178, 0.00971327795, 0.007039381476, 0.004139975606, 0.006298422154, 0.007683693862, 0.006556147171, 0.006266206562, 0.008038065823, 0.006459500253, 0.002045960324, 0.005299737916, -0.002593088642, -0.000176917277, 0.00072512006, -0.008520762611, 0.003560094455, -1.5839336e-05, -0.002689735533, 0.00162715736, 0.010776393408, 0.003495663209, 0.002271469654, 0.005170875573, 0.000660688703, 0.001562726015, 0.000306316884, 0.00433326959, -0.000756798482, -0.00088566104, 0.000950629274, 0.007458184574, -0.002464226375, 0.002851350901, 0.004977581747, -0.004268300959, 0.000241885618, -0.007683156529, 0.000499610685, 0.000596257441, -0.012869870941, -0.001240032773, 0.001852666757, -0.001755482742, 0.000338532524, 0.003237938423, 0.000982844877, -0.00465488834, 0.001208354438, -0.004332732289, -0.00439716343, -0.001980992089, 0.001272785514, -0.001626620296, -0.000499073601, 0.00011302319, 0.000145238779, -0.003044107473, -0.000627936068, 0.006105128423, 0.002754704251, -0.001819914024, -0.005331416306, 0.002690272893, -0.001175601605, -0.017605566811, -0.004010576067, -0.000756798598, 0.001530510569, -0.0031085386, -0.000692367314, -0.00043464232, -0.00243201077, -0.001948776439, 0.000531826343, -0.004944829054, 0.000564041886, -0.001916560853, -0.002721951342, -0.001755482724, 0.001369432409, 0.001337216768, -0.000466857914, 0.000338532547, 0.001594941687, -0.004268301024, -0.000144701788, -0.013546398954, -0.001111170311, 0.003044644539, -0.01138795252, -0.001884345101, -0.000176917422, -0.002625304487, -0.00459045693, -0.002464226377, -0.001497757785, -0.000370211149, -0.001948776482, 0.000306316881, -0.003076323116, -0.002850813822, 0.001079491784, -0.00017691741, -0.004107222904, -0.004332732246, 0.005267522609, -0.004010576099, -0.005331416449, 0.000692904471, -0.004654888454, -0.001240032869, -0.01093693355, 0.000757335615, 0.000145238936, -0.012515499095, -0.003559557329, -0.000144701823, -0.001980992119, -0.005266984899, -0.003720635472, 0.000628473076, -0.002496442015, -0.001691051542, -0.001143385984, -0.001368895318, -0.003269616796, 0.001530510483, -0.001755482733, 0.002496979324, -0.00194877647, 0.004204406837, 0.000789551196, -0.000337995397, -0.006169022139, -0.003140754237, -0.003140754355, -0.011420168147, 0.001949313631, -0.000305779871, -0.012193343063, -0.005621356895, -0.00330183249, 0.000628473056, -0.001529973401, -0.004912613443, -0.00017691742, -0.002270932657, -0.001626620302, 0.000370748149, -0.000789014142, -0.002979676268, -0.002335363916, -0.004622672856, -0.005621356935, 0.000113023148, 0.000338532643, -0.006555609732, 0.000113023288, 0.004268838148, -0.00117560164, -0.001562188997, -0.009648309123, -0.001626620228, -0.000563504846, -0.01583370792, -0.006684472351, -0.002142070113, -0.004880397743, -0.005943512973, -0.001304464111, -0.001240032853, -0.002270932685, -0.005395847667, -0.002174285534, 0.000596257577, -0.005170338311, -0.004944828915, -0.000531289242, 0.002496979125, -0.003366263629, -0.00101452346, -0.002883029441, -0.003656204215, -0.002528657596, -0.005041475746, -1.58393e-05, -0.009358368634, -0.001948776242, -0.001562189054, -0.01232220539, -0.008069743697, -0.004558241429, -0.003269616814, -0.002335363743], [0.022180723367, -1.804730281325, -1.842583469148, -1.668716514748, -1.496073706684, -1.347077029179, -1.205457663136, -1.07318075768, -0.977693947084, -0.877986880501, -0.798833304932, -0.710627144902, -0.636177006101, -0.572132478138, -0.515755243204, -0.464113687924, -0.416885658358, -0.376197384821, -0.335348028089, -0.307352685237, -0.274750510615, -0.250685464505, -0.225170714774, -0.204391655619, -0.179746723037, -0.165700721597, -0.148497590178, -0.137415422661, -0.12121097352, -0.108002574686, -0.099787594935, -0.090863871365, -0.068763962634, -0.077429962007, -0.069569352924, -0.067217613074, -0.056167658313, -0.050433279017, -0.049048007658, -0.046760699013, -0.038900089196, -0.036322839863, -0.035839605794, -0.033777806275, -0.022985574942, -0.025272883751, -0.02652929278, -0.024274199678, -0.017831076233, -0.018958622856, -0.018572035487, -0.018153232344, -0.013804123813, -0.012032265108, -0.009841603029, -0.015962570398, -0.00858519389, 0.004043328786, -0.016961254379, -0.008037528431, -0.017283410658, -0.013353105445, -0.007167706726, -0.012741008594, -0.00935836878, -0.005814650732, -0.005879081999, -0.007167706711, -0.004075007246, -0.003688419893, -0.012257774124, -0.006684472444, -0.005846866349, -0.004719319666, -0.007940881598, -0.005234769594, -0.006748903649, -0.007232137871, -0.003462910452, -0.005943513162, -0.008456331446, -0.001626620199, 0.010164296733, -0.007554294146, -0.003817282292, -0.011710108877, -0.00674890358, -0.000337995134, -0.004203869702, -0.006909981716, -0.003205185607, -0.002174285746, -0.005138122737, 0.003946682538, -0.002883029386, -0.003785066699, -0.006877766177, -0.00517033827, -0.00104673873, -0.005685788235, -0.002786382565, -0.006555609963, -0.005073691441, -0.003011891928, -0.000466857854, -0.003205185626, -0.000917876566, 0.010679746623, -0.006007944409, -0.002754166931, -0.010002681036, -0.00507369147, -0.003752851111, -0.001304464047, -0.005234769603, -0.003978360336, -0.000885660985, -0.002142070205, -0.00562135695, -0.003591773038, -0.004848182139, -0.000531289061, -0.001078954737, -0.002754166957, -0.005460278869, 0.001466079219, -0.006297884966, -0.006297884624, -0.00159440465, 0.001949313449, -0.007328784716, -0.000917876666, 0.009294474922, -0.006942196984, -0.003108538776, -0.006587825378, -0.002238716988, -0.00133667962, -0.005846866235, -0.002593088845, -0.002657519964, -0.002142070105, -0.00426830098, 0.001756019784, -0.002786382532, -0.00349512614, -0.003398479216, -0.002238717019, -0.002206501357, -0.00484818217, -0.000660151338, -0.003205185621, -0.001723267069, 0.00140164795, -0.001272248435, -0.003913929213, -0.001304464095, 0.012483821392, -0.001723267106, -0.004139438574, -0.011838971321, -0.007135491008, -0.002850813714, -0.005073691415, -0.003044107489, -0.004397163429, -0.00372063541, -0.001111170289, -0.003011891902, -0.001755482705, -0.005943513166, -0.001594404649, -0.002657520018, -0.003688419866, -0.003881713607, -0.003366263649, -0.004687104062, -0.001465542188, 0.000596257457, 0.005557462904, -0.002270932682, -0.003205185553, 0.011613999568, -0.006201238166, -0.001272248485, -0.013675261471, -0.003527341784, -0.004912613402, -0.003559557352, -0.003172969955, -0.000756798445, -0.001884345214, -0.003076323154, -0.001336679728, -0.003527341741, -0.002496441924, -0.003172970007, -0.004912613378, -0.001594404659, -0.004622672876, 0.000564041857, -0.003656204158, -0.005202553839, -0.002915245059, 0.003431232043, -0.003205185601, -0.002883029441, 0.009906571812, -0.00504147591, -0.002045423349, -0.009906034265, -0.004107222966, -0.000982307895, -0.002399795103, -0.001691051548, -0.005363632041, 0.000274101276, -0.003366263654, -0.001626620297, 0.001337216722, -0.00278638255, -0.003785066779, 0.00101506053, -0.002915245054, -0.002528657612, -0.002818598164, -0.003430694951, -0.007908665856, -0.002335363898, -0.000112485941, -0.001980992034, -0.003978360477, 0.012580468234, -0.005943513155, -0.002689735701, -0.011742324377, -0.002077638971, -4.8054954e-05, -0.003076323009, -0.006716687853, -0.003913929254, -0.000660151665, -0.006877765763, -0.002850813803, 0.001659372975, -0.004364947883, -0.003076323154, -0.000982307867, -0.009873818087, -0.00314075438, -0.021020422313, 1.788376815825, 1.841565263797, 1.667116237115, 1.497467545748, 1.342090617902, 1.205366760183, 1.0958653239, 0.973155488511, 0.876733766264, 0.776832789923, 0.703767545057, 0.634374914165, 0.57045897234, 0.511890851449, 0.462375350292, 0.413922976591, 0.372880215441, 0.335477830774, 0.301941330664, 0.268147109417, 0.247754602824, 0.22069345868, 0.198625742172, 0.176783537053, 0.160417992218, 0.141410766275, 0.13435554199, 0.117925568518, 0.116862452633, 0.095696782461, 0.08567772157, 0.089608028596, 0.06770140089, 0.066187266435, 0.048823044053, 0.049435140999, 0.047921006432, 0.046342441177, 0.037450928552, 0.035292481855, 0.034390444362, 0.028656063406, 0.025917735515, 0.025176776291, 0.018218201829, 0.017090655162, 0.018411495693, 0.015093286559, 0.013128133917, 0.014223464825, 0.013353643083, 0.013385858663, 0.013321427416, 0.011968371339, 0.004655425718, 0.005621894163, 0.021761920389, 0.003624525831, 0.010196512313, -0.003011891828, -0.002818597796, 0.006395068992, 0.006362853428, 0.001949313506, 0.005106444318, 0.007554831537, 0.004429916192, 0.001272785492, -0.000337995442, 0.0010794918, 0.003044644642, 0.004301053747, -0.001658835701, -0.001433326487, 0.018089339541, 0.001466079262, 0.000789551144, 0.004301053919, 0.001466079167, -0.003495126194, 0.002819135191, 0.010937471576, -0.003366263713, -0.000950092307, -0.008198606524, 0.003817819487, 0.000918413639, 0.001466079221, -0.003881713407, 0.002561410352, 0.001176138713, 0.00275470412, -0.001465542178, -0.000273564214, -0.003430694944, 0.001884882258, 0.002529194603, 0.002432547817, -0.001078954748, -0.002270932662, 0.000467394982, -0.001368895336, 0.000209670007, 0.004043328757, -0.00220650143, 0.002271469816, 0.016124186892, -0.002399795129, -0.003656204224, -0.0106147778, -0.000370211162, 0.00198152911, -0.001594404544, -0.001658835906, -0.003913929182, 0.00053182636, -0.002432010731, -0.000176917255, -0.000853445323, -0.000789014076, -0.002367579484, 0.002432547817, 4.8591916e-05, -0.002303148269, -0.003237401238, -0.000273564242, -0.002142070199, 0.003270153983, 0.001691588502, -0.00819860633, -0.001787698341, 0.014996639846, -0.007715372226, 0.001272785481, -0.009229506249, -0.002303148303, -0.000627936084, -0.002077638892, -0.003172970011, -0.00268973571, -0.001143385815, -0.003205185555, -0.000692367285, 0.002625841662, -0.002142070189, -0.001368895305, -0.000499073614, -0.002689735703, -0.00204542334, 0.000241885683, -0.002625304459, -0.0025608731549999998, 0.004172191588, 0.000306316874, -0.001014523351, 0.001015060499, 0.011291843382, -0.004268301033, -0.001143385994, -0.009132859242, -0.004977044531, -0.002464226384, -0.001175601499, -0.001240032876, -0.000885661038, 0.001111707361, 0.00143386365, 8.0807677e-05, -0.000853445413, 0.006362853635, 0.001788235383, -0.001143385928, -0.004268301011, -0.006104591281, -0.000627936087, -0.008939565526, 0.000145238762, -0.001401110942, -0.000917876669, -0.004075007317, -0.001336679574, 0.010615315481, -0.001916560855, -0.002850813797, -0.013030949208, -0.002947460685, -0.005524709904, -0.004010576037, -0.003849497986, 0.000564042035, 0.001111707527, -0.004461594744, -0.000563504805, 4.8591944e-05, -0.000176917179, -0.00275416695, 0.003205722631, 0.001852666617, -0.003817282412, -0.004654888416, -0.001755482766, -0.001980992097, -0.001626620305, 0.002722488352, 0.001691588671, -0.001852129622, 0.013450290104, -0.002560873255, -0.001111170363, -0.01026040596, -0.000756798578, -0.002625304504, -0.003849497988, -0.001529973416, 0.000628473103, 0.001466079196, -0.00201320768, -0.001819914009, -0.000241348588, -0.005266985108, -4.8054935e-05, 8.080772e-05, -0.00152997337, 0.000982844953, -0.002464226386, -0.004815966481, -0.002270932641, -0.001014523506, -8.0270578e-05, -0.000112486179, -0.000789014192, 0.011710646525, -0.00359177307, -0.002528657529, -0.010131543559, -0.004300516652, -0.000950092216, -0.004880397702, -0.004042791703, -0.002303148277, 0.000660688724, -0.005524710155, 0.000982845016, 0.000435179407, -0.003656204263, -0.003817282388, 0.000113023239, -0.002367579476, -0.001852129584]]
  in  "Open":bool
  in  "Filter lf":bool=TRUE caption="Scan"
  in  "Low cutoff freq: fl":dbl=10.0
  in  "Tab Control":enum32{"MOTOR", "DAQ        "}(tab)
  in  "COM":refnum<visa-resource-name>="COM9"
  in  "Encoder":bool=TRUE
  out "Motor Pulses X":i32
  in  "Motor counter X":tag="Dev1/ctr0"
  in  "Motor Counter X":tag="/Dev1/PFI8"
  out "Motor Pulses Y":u32
  in  "Motor Counter Y":tag="/Dev1/PFI10"
  in  "Motor counter Y":tag="Dev1/ctr1"
  in  "Y Auto Distance":i16=270
  in  "X Auto Distance":u16=270
  in  "Y Step":dbl=1.0
  in  "X Step":dbl=1.0
  out "No. X":i32
  out "No. Y":i32
  out "Get data":bool
  out "Completed":bool
  out "PLC Connceted":bool
  in  "No. Samples":dbl=500.0
  in  "Sample Rate 3":dbl=100000.0
  in  "Sample Clock Source 3":tag="OnboardClock"
  in  "Physical Channel 2":tag="Dev3/ai1:2"
  in  "Min Voltage  3":dbl=-10.0
  in  "Max Voltage 3":dbl=10.0
  in  "Terminal Configuration 2":i32(ring)=10083 items=["default"=-1, "RSE"=10083, "NRSE"=10078, "Differential"=10106, "Pseudodifferential"=12529]
  out "Actual Sample Rate 3":dbl=100000.0 format="%0.2f"
  in  "DAQ Pulser":bool=TRUE
  out "Sample per Channel AO":dbl=20000.0
  in  "Pulser Cycles":i32=10
  out "Actual Sample Rate 2":dbl=400000.0 format="%0.2f"
  in  "Physical Channel(s)":tag="Dev1/ao0:1"
  in  "Min Voltage 2":dbl=-10.0
  in  "Max Voltage 2":dbl=10.0
  in  "Sample Clock Source":tag="OnboardClock"
  in  "Sample Rate 2":dbl=400000.0 format="%#_6p"
  in  "Tab Control 5":enum32{"CONTROL", "DATA PROCESSING"}(tab)
  in  "Edge 2":i32(ring)=10280 items=["Rising"=10280, "Falling"=10171]
  in  "Pulser Trigger 2":tag="/Dev3/PFI0"
  in  "Save CSV":bool
  in  "Scan":bool
  in  "Exit":bool
  in  "Open tdms":bool
  in  "Save Scan mode":bool caption="Save Process"
  in  "Open csv":bool
  in  "Tab Control 3":enum32{"Basic", "Gaussian", "Chirp"}(tab)
  in  "Pulse Basic":T4={"Basic amp"=1.13, "Duty cycle %"=50.0, "Basic freq (Hz)"=200, "Basic Type"=2} {"Basic Type" items=["Sine Wave", "Triangle Wave", "Square Wave", "Sawtooth Wave"]; "Duty cycle %" format="%#.2f"; "Basic amp" format="%0.2p"}
  in  "Pulse Gaussian":T5={"Gauss amp"=2.1, "Gauss Nor. Band"=0.5, "Gauss atten (dB)"=6.0, "Gauss freq (Hz)"=1000.0}
  in  "Pulse chirp":T6={"Chirp amp"=1.6, "Chirp f2"=1500.0, "Chirp f1"=500.0} {"Chirp f1" format="%0.2f"; "Chirp f2" format="%0.2f"; "Chirp amp" format="%0.2f"}
  in  "X Distance":u32=100
  in  "Z Distance":i16=1
  in  "Y Distance":u32=100
  in  "Home":bool
  in  "Up Z":bool
  in  "Down Z":bool
  in  "Stop Button":bool
  in  "Y BW":bool
  in  "Y FW":bool
  in  "X LEFT":bool
  in  "X RIGHT":bool
  in  "Speed (mm/s)":i16=6
  in  "Min":dbl=-0.8
  in  "Max":dbl=0.6
  in  "ColorMapAutoScale":bool=TRUE
  in  "Plot style":i32(ring)=5 items=["cwLine"=1, "cwPoint"=2, "cwLinePoint"=3, "cwHiddenLine"=4, "cwSurface"=5, "cwSurfaceLine"=6, "cwSurfaceNormal"=7, "cwContourLine"=8, "cwSurfaceContour"=9]
  in  "ViewMode":i32(ring) items=["cwViewXYPlane", "cwViewXZPlane", "cwViewYZPlane", "cwViewUserDefined"]
  in  "Cursor":bool=TRUE
  in  "Return":bool caption="Scan"
  in  "Trim data":bool caption="Scan"
  in  "Abs":bool caption="Scan"
  in  "DiffY":bool caption="Scan"
  in  "DiffX":bool caption="Scan"
  in  "Odd":bool caption="Scan"
  in  "Backdata 2":bool caption="Scan"
  in  "Backindex":i32
  in  "Filter":bool caption="Scan"
  in  "Inverse":bool caption="Scan"
  in  "X-min":dbl
  in  "X-max":dbl=319.0
  in  "Y-min":dbl
  in  "Y-max":dbl=55.0
  in  "Line Row":dbl
  in  "Line Col":dbl=167.0
  in  "Repair Line Row":bool
  in  "Repair Line Col":bool
  # "PHENIKAA NON-DESTRUCTIVE TESTING SYSTEM"
  # "Developed by ICSLab"
  # "Power Spectal Density"
  # "Magnetic Sensors Signal"
  # "LIFT-OFF DATA COLLECTION"
  # "Feature Extraction"
  # "PLC CONNECT SETTING"
  # "ENCODER SETTING"
  # "SCAN SETTING"
  # "Step > S*P/f"
  # "GRADUATION PROJECT\nPham Phuong Huy\nFaculty of Electrical and Electronics Engineering\nSchool of Engineering – Phenikaa University"
  # "Pulser Channel"
  # "Pulser Timming"
  # "Sensor Channel"
  # "DAQ Timming"
  # "Trigger Settings"
  # "Data Processing"
  # "Time gate = %T/2"
  # "MANUAL MOVE (mm)"
  # "3D Surface"
  # "Process"
  # "Repair line"
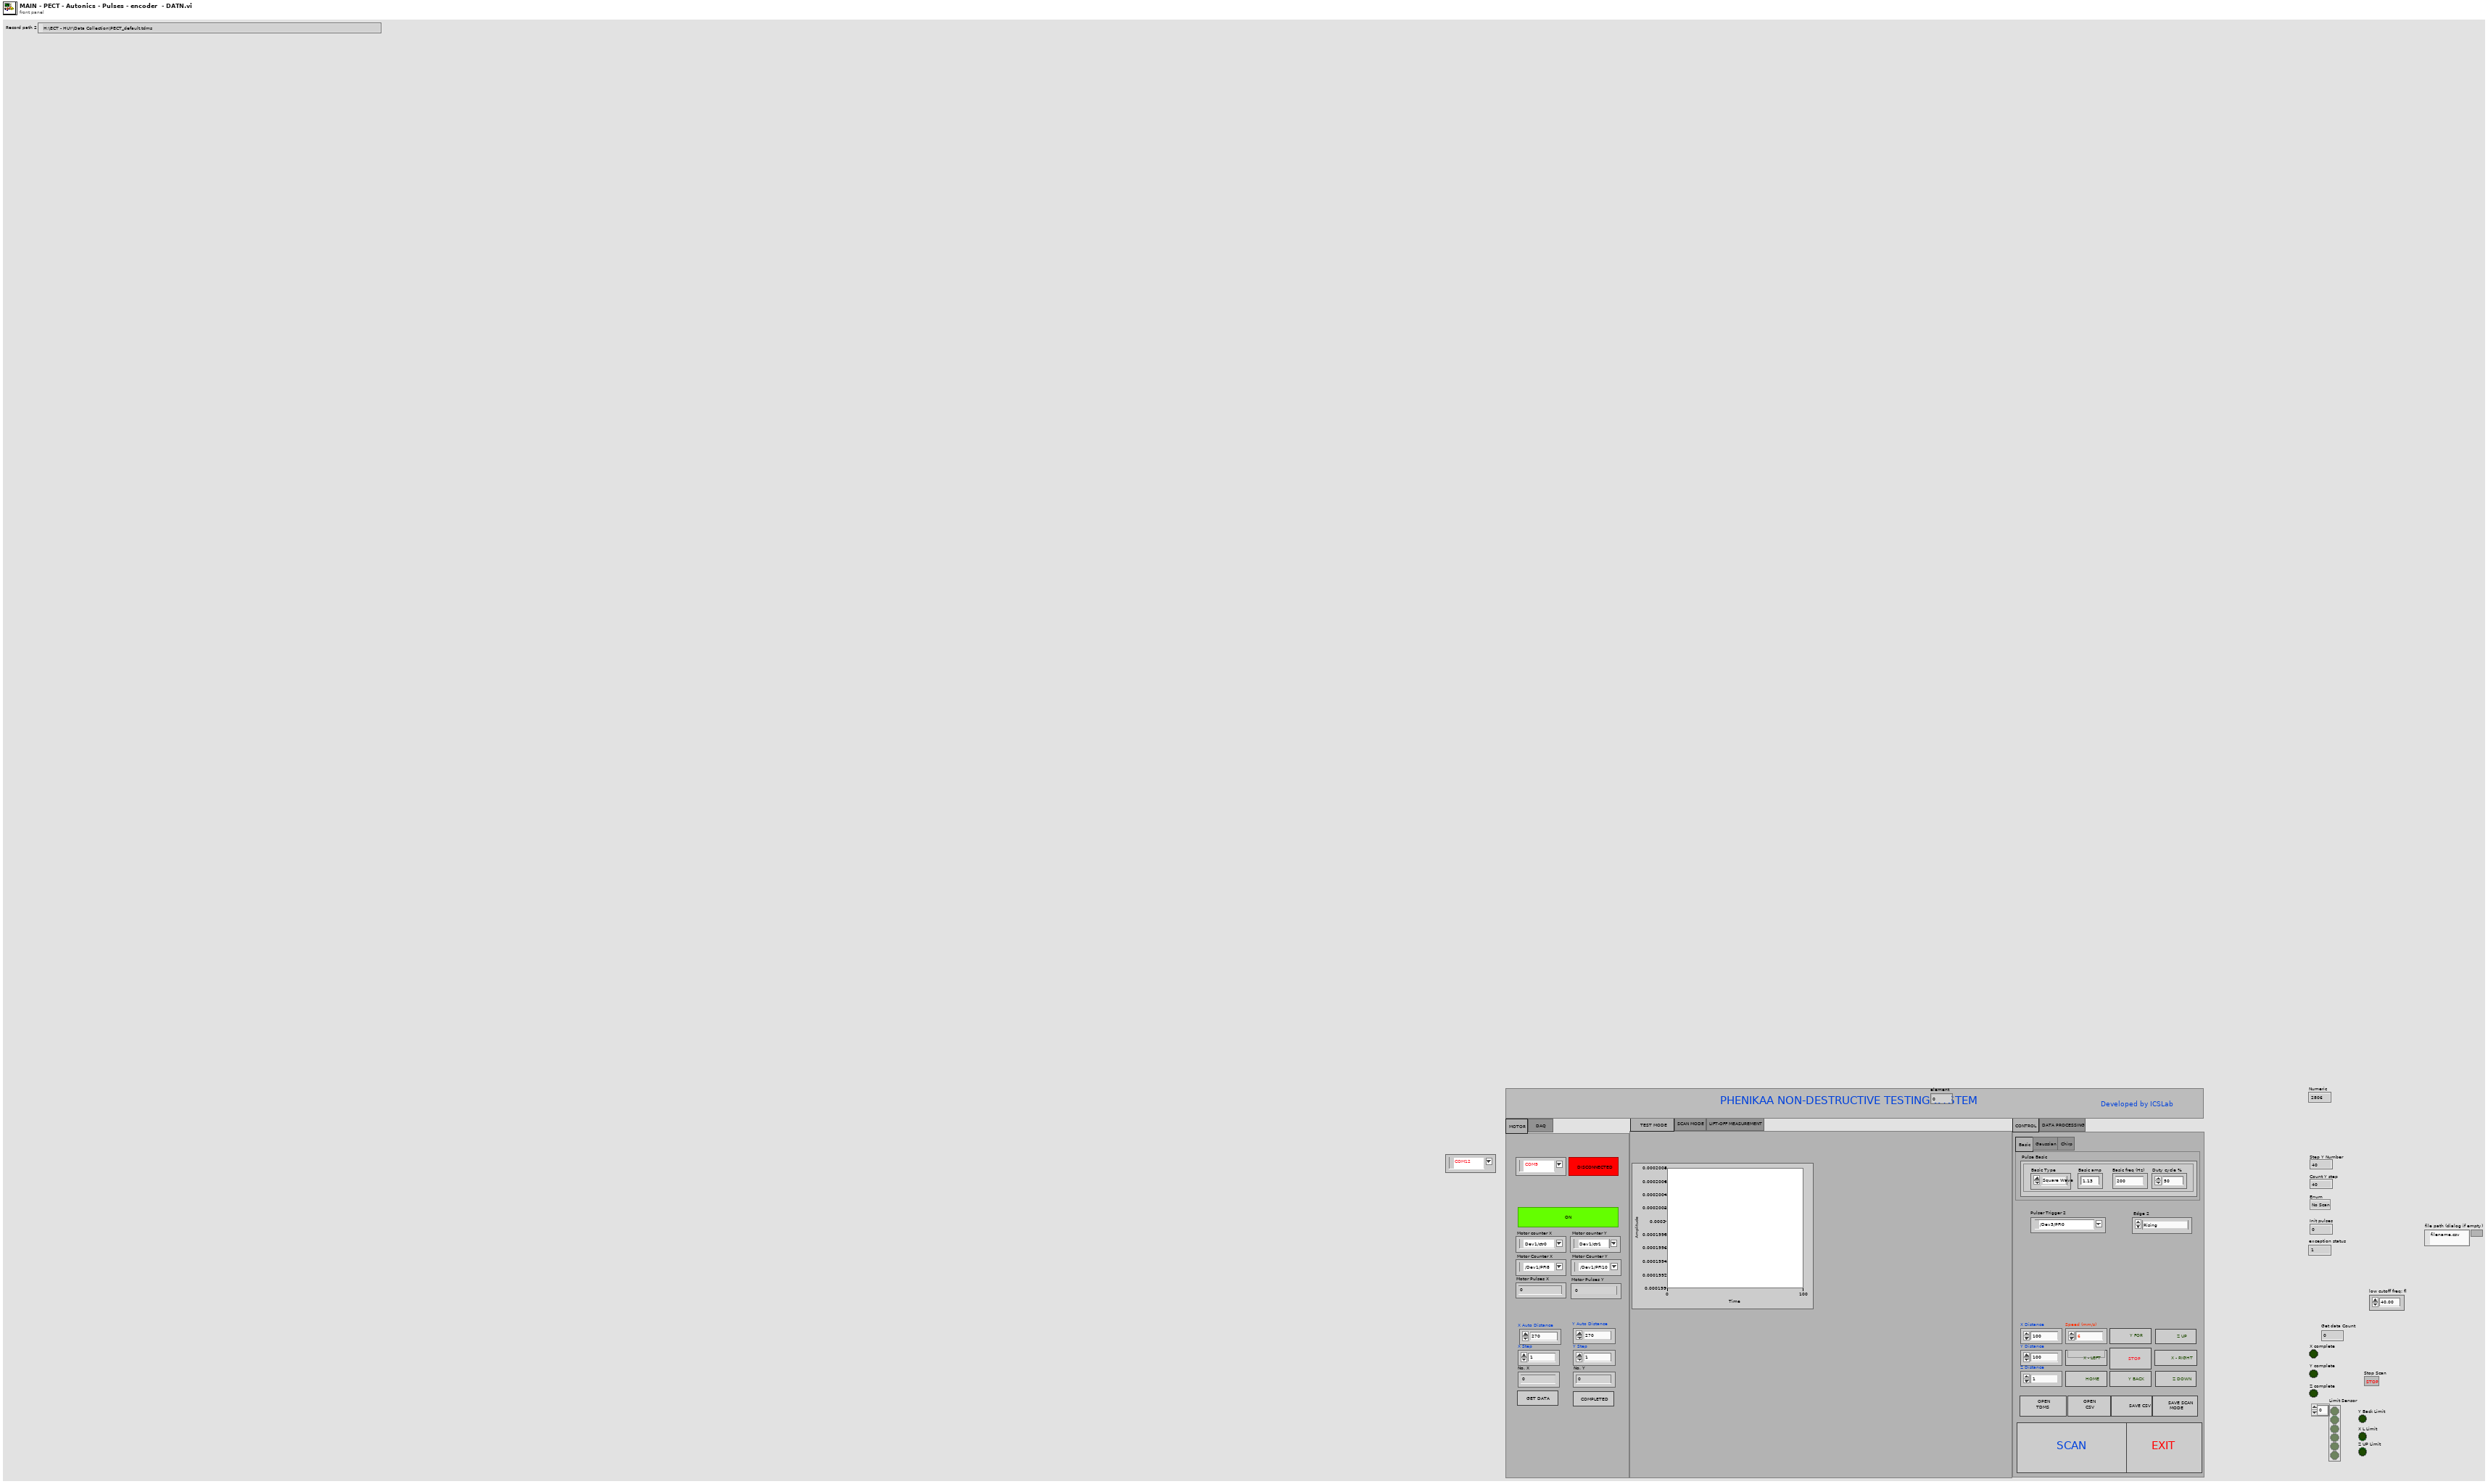
[diagram p1: front panel]
types:
  T1 = enum16{"No Scan", "Move X", "Wait X", "Move Y", "Wait Y"}
  T2 = enum32{"TEST MODE           ", "SCAN MODE", "LIFT-OFF MEASUREMENT"}
  T3 = typedef "Control 1.ctl" = dbl
  T4 = cluster{"Basic amp":T3, "Duty cycle %":dbl, "Basic freq (Hz)":u16, "Basic Type":u16}
  T5 = cluster{"Gauss amp":dbl, "Gauss Nor. Band":dbl, "Gauss atten (dB)":dbl, "Gauss freq (Hz)":dbl}
  T6 = cluster{"Chirp amp":dbl, "Chirp f2":dbl, "Chirp f1":dbl}
  T7 = enum16{"open", "open or create", "create or replace", "create", "open (read-only)"}
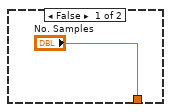
[diagram p2: hidden frame]
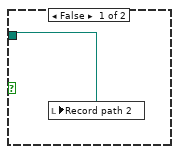
[diagram p3: hidden frame]
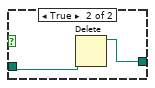
[diagram p4: hidden frame]
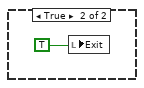
[diagram p5: hidden frame]
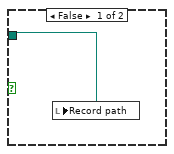
[diagram p7: hidden frame]
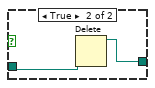
[diagram p8: hidden frame]
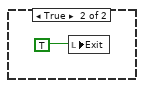
[diagram p9: hidden frame]
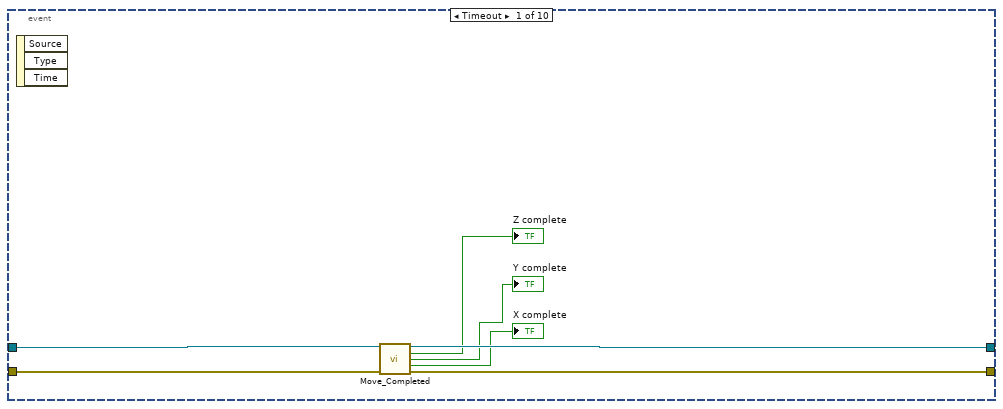
[diagram p11: hidden frame]
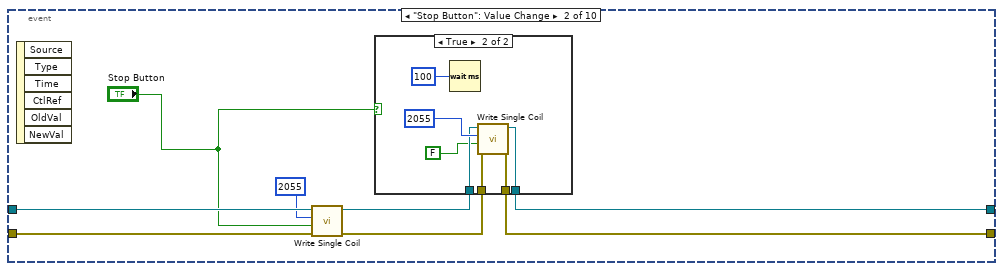
[diagram p12: hidden frame]
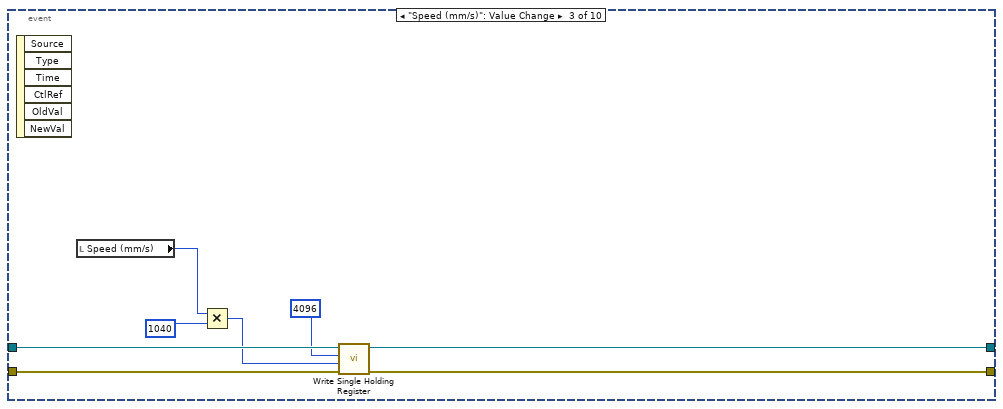
[diagram p14: hidden frame]
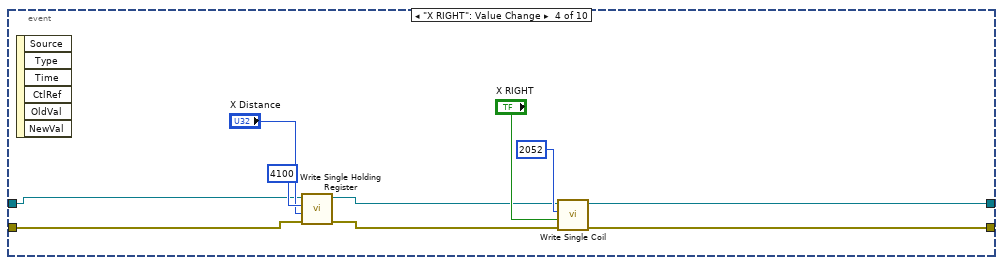
[diagram p15: hidden frame]
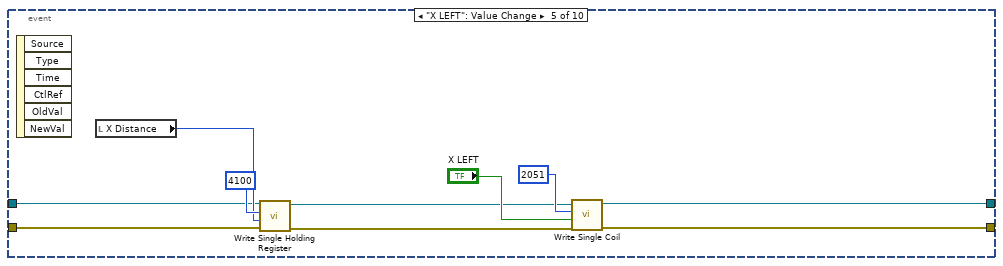
[diagram p16: hidden frame]
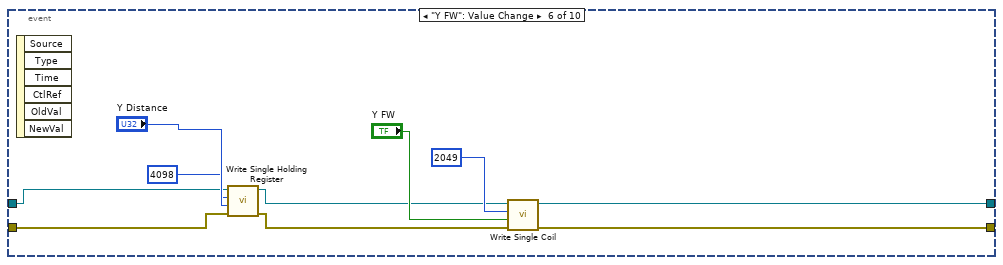
[diagram p17: hidden frame]
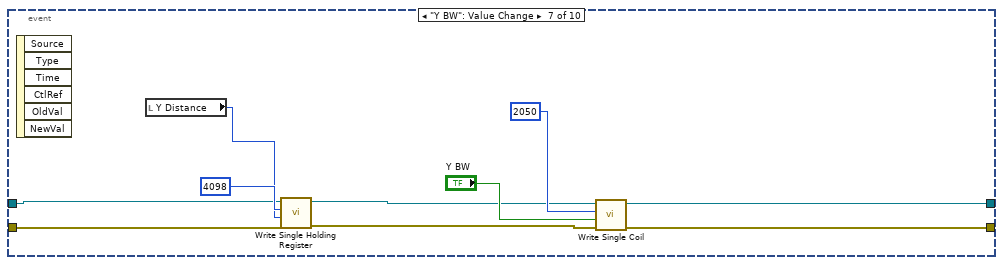
[diagram p18: hidden frame]
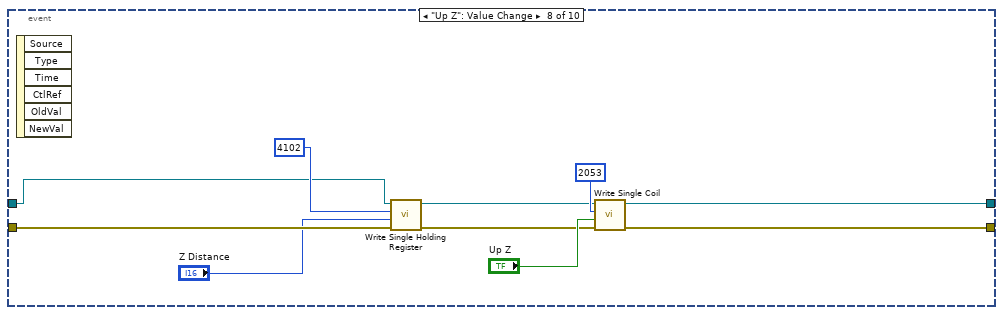
[diagram p19: hidden frame]
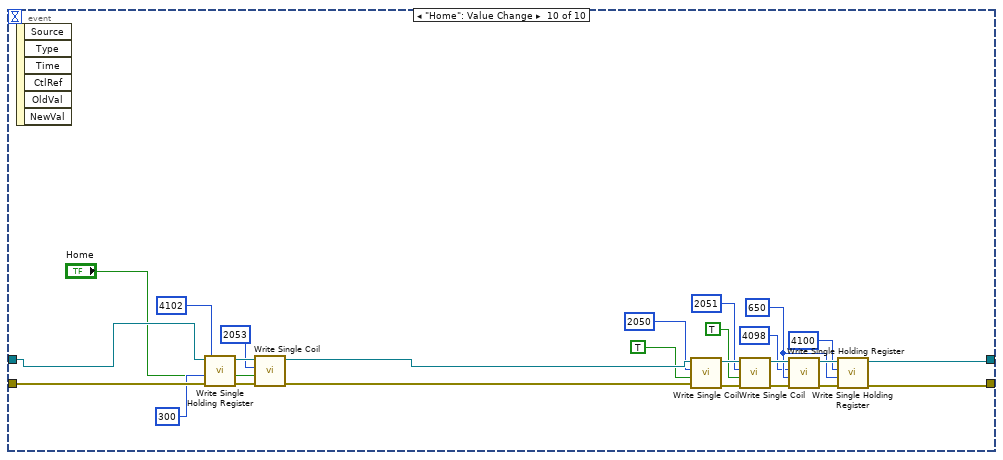
[diagram p20: hidden frame]
diagram:
  w11 = 10123 items=["Finite Samples"=10178, "Continuous Samples"=10123, "Hardware Timed Single Point"=12522] ("sample mode")
  w62 = u16 0 items=["None", "XON/XOFF", "RTS/CTS", "XON/XOFF & RTS/CTS", "DTR/DSR", "XON/XOFF & DTR/DSR"] ("flow control (none)")
  w61 = u16 2 items=["None", "Odd", "Even", "Mark", "Space"] ("parity (even)")
  # "Count Y step"
  n1 = flat-sequence {
    tunnel: [w133] -> w78
    tunnel: [TRUE ("disable buffering (T)")] -> _
    tunnel: [w127] -> _
    frame #0 {
      w86 = FALSE ("Exit")
      n2 = local write "Scan"(w86) -> ()
      n3 = local write "Exit"(w86) -> ()
    }
    frame #1 {
      n4 = disable-structure shown="Enabled" {
        frame Enabled {
          n5 = call "File Dialog"("prompt"="Choose New File For Recording\n" ("button label"), "default name"="PECT_default", "pattern (all files)"="*.tdms") -> ("selected path"=w112:path, "exists"=w108:bool, "cancelled"=w109:bool)  [unwired: 9 in, 1 out]
          n6 = case shown="False" w109 {
            tunnel: w112 -> [w113 _]
            tunnel: w108 -> [w114 _]
            frame False {
              n7 = case shown="True" w114 {
                tunnel: w113 -> [w115 w116]
                frame False {
                  n8 = local write "Record path"(w115) -> ()
                }
                frame True {
                  n9 = Two Button Dialog(message="Existing File\nDo you want to Replace?", 1:"No" ("F button name (\"Cancel\")"), 2:"Replace" ("T button name (\"OK\")")) -> (T button?=w117:bool)
                  n10 = case shown="False" w117 {
                    tunnel: w116 -> [_ w125]
                    tunnel: [path "" ("deleted path") w124] -> w118
                    frame False {
                      n11 = local write "Exit"(TRUE ("Exit")) -> ()
                    }
                    frame True {
                      n12 = Delete(path (use dialog)=w125) -> (deleted path=w124:path)  [unwired: 4 in, 2 out]
                    }
                  }
                  "Record path" <- w118
                }
              }
            }
            frame True {
              n13 = local write "Exit"(TRUE ("Exit")) -> ()
            }
          }
        }
        frame Disabled {
        }
      }
      n14 = disable-structure shown="Enabled" {
        frame Enabled {
          n15 = call "File Dialog2"("prompt"="Choose New File For Recording\n" ("button label"), "default name"="PECT_default", "pattern (all files)"="*.tdms") -> ("selected path"=w92:path, "exists"=w88:bool, "cancelled"=w89:bool)  [unwired: 9 in, 1 out]
          n16 = case shown="False" w89 {
            tunnel: w92 -> [w93 _]
            tunnel: w88 -> [w94 _]
            frame False {
              n17 = case shown="True" w94 {
                tunnel: w93 -> [w95 w96]
                frame False {
                  n18 = local write "Record path 2"(w95) -> ()
                }
                frame True {
                  n19 = Two Button Dialog(message="Existing File\nDo you want to Replace?", 1:"No" ("F button name (\"Cancel\")"), 2:"Replace" ("T button name (\"OK\")")) -> (T button?=w97:bool)
                  n20 = case shown="False" w97 {
                    tunnel: w96 -> [_ w105]
                    tunnel: [path "" ("deleted path") w104] -> w98
                    frame False {
                      n21 = local write "Exit"(TRUE ("Exit")) -> ()
                    }
                    frame True {
                      n22 = Delete(path (use dialog)=w105) -> (deleted path=w104:path)  [unwired: 4 in, 2 out]
                    }
                  }
                  "Record path 2" <- w98
                }
              }
            }
            frame True {
              n23 = local write "Exit"(TRUE ("Exit")) -> ()
            }
          }
        }
        frame Disabled {
        }
      }
    }
    frame #2 {
      n24 = local read "Record path"() -> (w132:path)
      n25 = local read "Record path 2"() -> (w129:path)
      n26 = local write "Completed"(FALSE ("Completed")) -> ()
      n27 = TDMS Open(6:FALSE ("disable buffering (T)"), 10:T7."create or replace" ("operation"), 11:w132) -> (3:w133:refnum<k34>)  [unwired: 4 in, 1 out]
      n28 = TDMS Open(10:T7."create or replace" ("operation (0:open)"), 11:w129) -> (3:w127:refnum<k34>)  [unwired: 5 in, 1 out]
    }
  }
  n29 = call-poly <vilib>:"Create Modbus Instance.vi"("flow control (none)"=w62, "serial type"=enum16{"RTU", "ASCII"}."ASCII", "parity (even)"=w61, "unit ID"=u8 1, "baud rate"=u32 9600, "VISA resource name"="COM") -> ("error out"=w46:errorcluster, "serial master instance"=w47:refnum<class "Modbus Master.lvclass">)  [unwired: 4 in]
  n30 = local write "Init pulses"(0 ("Init pulses")) -> ()
  n31 = Multiply(x="Speed (mm/s)", y=i16 1040 ("Speed (mm/s)")) -> (x*y=w51:i16)
  n32 = call-dynamic "Write Single Holding Register.vi"("error in"=w46, "register to write"=w51, "address"=u16 4096, "Modbus master in"=w47) -> ("error out"=w48:errorcluster, "Modbus master out"=w49:refnum<class "Modbus Master.lvclass">)  [unwired: 6 in]
  n33 = call-poly <vilib>:"DAQmx Create Virtual Channel.vi"("maximum value"="Max Voltage 3", "minimum value"="Min Voltage  3", "input terminal configuration"="Terminal Configuration 2", "physical channels"="Physical Channel 2", "name to assign"="Acquisition Task") -> ("task out"=w19:refnum<k21>, "error out"=w18:errorcluster)  [unwired: 9 in]
  n34 = local read "DAQ Pulser"() -> (w8:bool)
  n35 = call-poly "VISA Configure Serial Port"("VISA resource name"="COM 2", "termination char\n(0xA = '\\n' = LF)"=u8 10 ("termination char\n(0xA = '\\n' = LF)"), "Enable Termination\nChar (T)"=TRUE ("Enable Termination\nChar (T)"), "baud rate (9600)"=u32 9600, "data bits (8)"=u16 8, "parity (0:none)"=enum16{"None", "Odd", "Even", "Mark", "Space"}."None") -> ("VISA resource name out"=w35:refnum<visa-resource-name>, "error out"=w36:errorcluster)  [unwired: 8 in]
  n36 = case shown="True" w8 {
    tunnel: ["No. Samples" w140] -> w6
    tunnel: "Sample Rate 3" -> [_ w137]
    frame False {
    }
    frame True {
      n37 = local read "Pulse Basic"() -> (w139:T4)
      n38 = Unbundle By Name(w139) -> ("Basic freq (Hz)"=w138:u16)
      n39 = Divide(x=w137, y=w138) -> (x/y=w141:dbl)
      n40 = Round Toward -Infinity(1:w141) -> (0:w140:dbl)
      n41 = local write "No. Samples"(w140) -> ()
    }
  }
  n42 = VISA Open(error in (no error)=w36, VISA resource name=w35) -> (VISA resource name=w30:refnum<visa-resource-name>, error out=w29:errorcluster)  [unwired: 3 in]
  n43 = call-poly <vilib>:"DAQmx Timing.vi"("task/channels in"=w19, "sample mode"=w11, "samples per channel"=w6, "rate"="Sample Rate 3", "source"="Sample Clock Source 3", "error in"=w18) -> ("task out"=w17:refnum<k21>, "error out"=w16:errorcluster)  [unwired: 8 in]
  n44 = while {
    shift-right: [w154] -> w42
    shift-left: w49 -> [w156]
    shift-right: [w151] -> w43
    shift-left: w48 -> [w155]
    tunnel: [w149] -> w45
    tunnel: [w150] -> w44
    stop <- w161 stop-if-true
    n45 = call-dynamic "Read Exception Status.vi"("error in"=w155, "Modbus master in"=w156) -> ("error out"=w157:errorcluster, "exception status"=w159:u8)  [unwired: 7 in, 1 out]
    "exception status" <- w159
    n46 = call <vilib>:"Clear Errors.vi"("error in (no error)"=w157) -> ()  [unwired: 5 in, 2 out]
    n47 = Not Equal To 0?(x=w159) -> (x != 0?=→"PLC Connceted":bool)
    n48 = event shown="[8] \"Down Z\": Value Change" {
      selector: _ -> [_ _ _ _ _ _ _ _ _ _]
      dyn-events: _ -> [_ _ _ _ _ _ _ _ _ _]
      timeout: 100 -> [_ _ _ _ _ _ _ _ _ _]
      tunnel: w156 -> [w166 w176 w193 w195 w205 w215 w226 w236 w249 w277]
      tunnel: [w167 w171 w192 w202 w213 w222 w233 w243 w245 w255] -> w154
      tunnel: w155 -> [w165 w175 w191 w194 w204 w216 w225 w235 w248 w276]
      tunnel: [w168 w170 w190 w201 w212 w221 w232 w242 w244 w254] -> w151
      event Timeout {
        n49 = event-data() -> ()  [unwired: 1 in, 3 out]
        n50 = call "Move_Completed.vi"("serial master instance"=w166, "error in"=w165) -> ("Modbus master out"=w167:refnum<class "Modbus Master.lvclass">, "Z completed"=→"Z complete":bool, "Y completed"=→"Y complete":bool, "X completed"=→"X complete":bool, "error out"=w168:errorcluster)  [unwired: 9 in]
      }
      event "Stop Button": Value Change {
        n51 = event-data() -> ()  [unwired: 1 in, 6 out]
        n52 = call-dynamic "Write Single Coil.vi"("error in"=w175, "coil to write"="Stop Button", "address"=u16 2055, "Modbus master in"=w176) -> ("error out"=w173:errorcluster, "Modbus master out"=w172:refnum<class "Modbus Master.lvclass">)  [unwired: 6 in]
        n53 = case shown="True" "Stop Button" {
          tunnel: w172 -> [w177 w183]
          tunnel: w173 -> [w178 w182]
          tunnel: [w177 w181] -> w171
          tunnel: [w178 w180] -> w170
          frame False {
          }
          frame True {
            n54 = Wait (ms)(milliseconds to wait=u32 100 ("millisecond timer value")) -> ()  [unwired: 1 out]
            n55 = call-dynamic "Write Single Coil.vi"("error in"=w182, "coil to write"=FALSE, "address"=u16 2055, "Modbus master in"=w183) -> ("error out"=w180:errorcluster, "Modbus master out"=w181:refnum<class "Modbus Master.lvclass">)  [unwired: 6 in]
          }
        }
      }
      event "Speed (mm/s)": Value Change {
        n56 = event-data() -> ()  [unwired: 1 in, 6 out]
        n57 = local read "Speed (mm/s)"() -> (w186:i16)
        n58 = Multiply(x=w186, y=i16 1040 ("Speed (mm/s)")) -> (x*y=w188:i16)
        n59 = call-dynamic "Write Single Holding Register.vi"("error in"=w191, "register to write"=w188, "address"=u16 4096, "Modbus master in"=w193) -> ("error out"=w190:errorcluster, "Modbus master out"=w192:refnum<class "Modbus Master.lvclass">)  [unwired: 6 in]
      }
      event "X RIGHT": Value Change {
        n60 = event-data() -> ()  [unwired: 1 in, 6 out]
        n61 = call-dynamic "Write Single Holding Register.vi"("error in"=w194, "register to write"="X Distance", "address"=u16 4100, "Modbus master in"=w195) -> ("error out"=w196:errorcluster, "Modbus master out"=w197:refnum<class "Modbus Master.lvclass">)  [unwired: 6 in]
        n62 = call-dynamic "Write Single Coil.vi"("error in"=w196, "coil to write"="X RIGHT", "address"=u16 2052, "Modbus master in"=w197) -> ("error out"=w201:errorcluster, "Modbus master out"=w202:refnum<class "Modbus Master.lvclass">)  [unwired: 6 in]
      }
      event "X LEFT": Value Change {
        n63 = event-data() -> ()  [unwired: 1 in, 6 out]
        n64 = local read "X Distance"() -> (w206:u32)
        n65 = call-dynamic "Write Single Holding Register.vi"("error in"=w204, "register to write"=w206, "address"=u16 4100, "Modbus master in"=w205) -> ("error out"=w207:errorcluster, "Modbus master out"=w208:refnum<class "Modbus Master.lvclass">)  [unwired: 6 in]
        n66 = call-dynamic "Write Single Coil.vi"("error in"=w207, "coil to write"="X LEFT", "address"=u16 2051, "Modbus master in"=w208) -> ("error out"=w212:errorcluster, "Modbus master out"=w213:refnum<class "Modbus Master.lvclass">)  [unwired: 6 in]
      }
      event "Y FW": Value Change {
        n67 = event-data() -> ()  [unwired: 1 in, 6 out]
        n68 = call-dynamic "Write Single Holding Register.vi"("error in"=w216, "register to write"="Y Distance", "address"=u16 4098, "Modbus master in"=w215) -> ("error out"=w217:errorcluster, "Modbus master out"=w218:refnum<class "Modbus Master.lvclass">)  [unwired: 6 in]
        n69 = call-dynamic "Write Single Coil.vi"("error in"=w217, "coil to write"="Y FW", "address"=u16 2049, "Modbus master in"=w218) -> ("error out"=w221:errorcluster, "Modbus master out"=w222:refnum<class "Modbus Master.lvclass">)  [unwired: 6 in]
      }
      event "Y BW": Value Change {
        n70 = event-data() -> ()  [unwired: 1 in, 6 out]
        n71 = local read "Y Distance"() -> (w224:u32)
        n72 = call-dynamic "Write Single Holding Register.vi"("error in"=w225, "register to write"=w224, "address"=u16 4098, "Modbus master in"=w226) -> ("error out"=w227:errorcluster, "Modbus master out"=w228:refnum<class "Modbus Master.lvclass">)  [unwired: 6 in]
        n73 = call-dynamic "Write Single Coil.vi"("error in"=w227, "coil to write"="Y BW", "address"=u16 2050, "Modbus master in"=w228) -> ("error out"=w232:errorcluster, "Modbus master out"=w233:refnum<class "Modbus Master.lvclass">)  [unwired: 6 in]
      }
      event "Up Z": Value Change {
        n74 = event-data() -> ()  [unwired: 1 in, 6 out]
        n75 = call-dynamic "Write Single Holding Register.vi"("error in"=w235, "register to write"="Z Distance", "address"=u16 4102, "Modbus master in"=w236) -> ("error out"=w238:errorcluster, "Modbus master out"=w237:refnum<class "Modbus Master.lvclass">)  [unwired: 6 in]
        n76 = call-dynamic "Write Single Coil.vi"("error in"=w238, "coil to write"="Up Z", "address"=u16 2053, "Modbus master in"=w237) -> ("error out"=w242:errorcluster, "Modbus master out"=w243:refnum<class "Modbus Master.lvclass">)  [unwired: 6 in]
      }
      event "Down Z": Value Change {
        n77 = event-data() -> ()  [unwired: 1 in, 6 out]
        n78 = local read "Z Distance"() -> (w250:i16)
        n79 = call-dynamic "Write Single Holding Register.vi"("error in"=w248, "register to write"=w250, "address"=u16 4102, "Modbus master in"=w249) -> ("error out"=w246:errorcluster, "Modbus master out"=w247:refnum<class "Modbus Master.lvclass">)  [unwired: 6 in]
        n80 = call-dynamic "Write Single Coil.vi"("error in"=w246, "coil to write"="Down Z", "address"=u16 2054, "Modbus master in"=w247) -> ("error out"=w244:errorcluster, "Modbus master out"=w245:refnum<class "Modbus Master.lvclass">)  [unwired: 6 in]
      }
      event "Home": Value Change {
        w260 = u16 650 ("register to write")
        n81 = event-data() -> ()  [unwired: 1 in, 6 out]
        n82 = call-dynamic "Write Single Holding Register.vi"("error in"=w276, "register to write"=u16 300, "address"=u16 4102, "Modbus master in"=w277) -> ("error out"=w273:errorcluster, "Modbus master out"=w272:refnum<class "Modbus Master.lvclass">)  [unwired: 6 in]
        n83 = call-dynamic "Write Single Coil.vi"("error in"=w273, "coil to write"="Home", "address"=u16 2053, "Modbus master in"=w272) -> ("error out"=w275:errorcluster, "Modbus master out"=w278:refnum<class "Modbus Master.lvclass">)  [unwired: 6 in]
        n84 = call-dynamic "Write Single Coil.vi"("error in"=w275, "coil to write"=TRUE, "address"=u16 2050, "Modbus master in"=w278) -> ("error out"=w267:errorcluster, "Modbus master out"=w268:refnum<class "Modbus Master.lvclass">)  [unwired: 6 in]
        n85 = call-dynamic "Write Single Coil.vi"("error in"=w267, "coil to write"=TRUE, "address"=u16 2051, "Modbus master in"=w268) -> ("error out"=w265:errorcluster, "Modbus master out"=w266:refnum<class "Modbus Master.lvclass">)  [unwired: 6 in]
        n86 = call-dynamic "Write Single Holding Register.vi"("error in"=w265, "register to write"=w260, "address"=u16 4098, "Modbus master in"=w266) -> ("error out"=w263:errorcluster, "Modbus master out"=w264:refnum<class "Modbus Master.lvclass">)  [unwired: 6 in]
        n87 = call-dynamic "Write Single Holding Register.vi"("error in"=w263, "register to write"=w260, "address"=u16 4100, "Modbus master in"=w264) -> ("error out"=w254:errorcluster, "Modbus master out"=w255:refnum<class "Modbus Master.lvclass">)  [unwired: 6 in]
      }
    }
    n88 = call-dynamic "Read Discrete Inputs.vi"("error in"=w151, "number of inputs"=u16 6, "starting address"=u16 1024, "Modbus master in"=w154) -> ("error out"=w150:errorcluster, "discrete inputs"=w148:bool[], "Modbus master out"=w149:refnum<class "Modbus Master.lvclass">)  [unwired: 5 in]
    "Limit Sensor" <- w148
    n89 = Index Array(array=w148, index #1=4 ("index"), index #2=3 ("index"), index #3=0 ("index")) -> (element #1=→"Z UP Limit":bool, element #2=→"X L Limit":bool, element #3=→"Y Back Limit":bool)
    n90 = Unbundle By Name(w151) -> ("status"=w161:bool)
  }
  n91 = case shown="True" "Encoder" {
    frame False {
    }
    frame True {
      # "Counter pulses from Motor\nto pick up signal"
      n92 = call-poly <vilib>:"DAQmx Create Virtual Channel.vi"("counter"="Motor counter X") -> ("task out"=w284:refnum<k21>, "error out"=w283:errorcluster)  [unwired: 13 in]
      n93 = call-poly <vilib>:"DAQmx Create Virtual Channel.vi"("counter"="Motor counter Y") -> ("task out"=w281:refnum<k21>, "error out"=w280:errorcluster)  [unwired: 13 in]
      n94 = property class="DAQmx Channel"(reference=w284, error in=w283, "CI.CountEdges.Term"="Motor Counter X") -> (reference out=w297:refnum<k21>, error out=w298:errorcluster)
      n95 = property class="DAQmx Channel"(reference=w281, error in=w280, "CI.CountEdges.Term"="Motor Counter Y") -> (reference out=w293:refnum<k21>, error out=w292:errorcluster)
      n96 = call <vilib>:"DAQmx Start Task.vi"("task/channels in"=w293, "error in"=w292) -> ("task out"=w291:refnum<k21>, "error out"=w290:errorcluster)  [unwired: 12 in]
      n97 = call <vilib>:"DAQmx Start Task.vi"("task/channels in"=w297, "error in"=w298) -> ("task out"=w299:refnum<k21>, "error out"=w296:errorcluster)  [unwired: 12 in]
      n98 = while {
        tunnel: w299 -> [w326]
        tunnel: w296 -> [w325]
        tunnel: [w319] -> w304
        tunnel: [w324] -> w303
        shift-right: [w318] -> _
        shift-left: u32 0 ("data") -> [w317]
        tunnel: w291 -> [w313]
        tunnel: w290 -> [w312]
        tunnel: [w311] -> w286
        tunnel: [w310] -> w285
        shift-right: [w307] -> _
        shift-left: u32 0 ("data") -> [w308]
        i -> [w314]
        stop <- w320 stop-if-true
        n99 = local read "Scan"() -> (w315:bool)
        n100 = call-poly <vilib>:"DAQmx Read.vi"("task/channels in"=w313, "error in"=w312) -> ("task out"=w311:refnum<k21>, "data"=→"Motor Pulses Y":u32, "error out"=w310:errorcluster)  [unwired: 11 in]
        n101 = call-poly <vilib>:"DAQmx Read.vi"("task/channels in"=w326, "error in"=w325) -> ("task out"=w324:refnum<k21>, "data"=w316:u32, "error out"=w319:errorcluster)  [unwired: 11 in]
        "Motor Pulses X" <- w316
        n102 = case shown="True" w315 {
          tunnel: [w328 w341] -> w318
          tunnel: w317 -> [w328 w340]
          tunnel: w316 -> [_ w333]
          tunnel: w308 -> [w327 w330]
          tunnel: [w327 w329] -> w307
          frame False {
          }
          frame True {
            n103 = local read "Init pulses"() -> (w332:i32)
            n104 = Subtract(x=w333, y=w332) -> (x-y=w331:u32)
            n105 = local read "X Step"() -> (w339:dbl)
            n106 = Multiply(x=w339, y=10.0) -> (x*y=w337:dbl)
            n107 = To Long Integer(number=w337) -> (32bit integer=w336:i32)
            n108 = Add(x=w336, y=w340) -> (x+y=w335:u32)
            n109 = Greater Or Equal?(x=w331, y=w335) -> (x >= y?=w334:bool)
            n110 = case shown="True" w334 {
              selector: w334 -> [_ w345]
              tunnel: w330 -> [w342 w344]
              tunnel: [w342 w343] -> w329
              frame False {
              }
              frame True {
                n111 = Increment(x=w344) -> (x+1=w343:u32)
                "Get data" <- w345
              }
            }
            n112 = Select(t=w331, s=w334, f=w340) -> (s? t:f=w341:u32)
          }
        }
        "Get data Count" <- w307
        n113 = Wait Until Next ms Multiple(millisecond multiple=u32 10 ("milliseconds to wait")) -> ()  [unwired: 1 out]
        n114 = local read "Completed"() -> (w321:bool)
        n115 = Unbundle By Name(w319) -> ("status"=w322:bool)
        n116 = Compound Arithmetic op=OR(w322, w321) -> (w320:bool)
        "Numeric" <- w314
      }
      n117 = call <vilib>:"DAQmx Stop Task.vi"("task/channels in"=w303, "error in"=w304) -> ("task out"=w306:refnum<k21>, "error out"=w305:errorcluster)  [unwired: 12 in]
      n118 = call <vilib>:"DAQmx Stop Task.vi"("task/channels in"=w286, "error in"=w285) -> ("task out"=w287:refnum<k21>, "error out"=w288:errorcluster)  [unwired: 12 in]
      n119 = call <vilib>:"DAQmx Clear Task.vi"("task in"=w306, "error in"=w305) -> ("error out"=w300:errorcluster)  [unwired: 13 in]
      n120 = call <vilib>:"DAQmx Clear Task.vi"("task in"=w287, "error in"=w288) -> ("error out"=w289:errorcluster)  [unwired: 13 in]
      n121 = call <vilib>:"Simple Error Handler.vi"("error in (no error)"=w300) -> ()  [unwired: 4 in, 5 out]
      n122 = call <vilib>:"Simple Error Handler.vi"("error in (no error)"=w289) -> ()  [unwired: 4 in, 5 out]
    }
  }
  n123 = case shown="False" "DAQ Pulser" {
    frame False {
    }
    frame True {
      (unwired) 1 ("x")
      w378 = 10123 items=["Finite Samples"=10178, "Continuous Samples"=10123, "Hardware Timed Single Point"=12522]  # Sample Mode
      n124 = local read "Pulse Basic"() -> (w353:T4)
      n125 = Unbundle By Name(w353) -> ("Basic freq (Hz)"=w352:u16)
      n126 = call-poly <vilib>:"DAQmx Create Virtual Channel.vi"("maximum value"="Max Voltage 2", "minimum value"="Min Voltage 2", "physical channels"="Physical Channel(s)", "name to assign"="Pulser Task") -> ("task out"=w372:refnum<k21>, "error out"=w371:errorcluster)  [unwired: 10 in]
      n127 = Divide(x="Sample Rate 2", y=w352) -> (x/y=w369:dbl)
      n128 = Multiply(x="Pulser Cycles", y=w369) -> (x*y=w368:dbl)
      n129 = Round Toward -Infinity(1:w368) -> (0:w360:dbl)
      "Sample per Channel AO" <- w360
      n130 = call-poly <vilib>:"DAQmx Timing.vi"("task/channels in"=w372, "sample mode"=w378, "samples per channel"=w360, "rate"="Sample Rate 2", "source"="Sample Clock Source", "error in"=w371) -> ("task out"=w380:refnum<k21>, "error out"=w379:errorcluster)  [unwired: 8 in]
      n131 = property class="DAQmx Timing"(reference=w380, error in=w379) -> (reference out=w367:refnum<k21>, error out=w354:errorcluster, "SampClk.Rate"=w355:dbl)
      "Actual Sample Rate 2" <- w355
      n132 = call "waveform_generator.vi"("Sampling rate"=w355, "Pulse chirp"="Pulse chirp", "Pulse Gaussian"="Pulse Gaussian", "Cluster Basic"="Pulse Basic", "Tab Control"="Tab Control 3") -> ("Waveform Graph"=w351:waveform(dbl)[])  [unwired: 6 in]
      n133 = call-poly <vilib>:"DAQmx Write.vi"("task/channels in"=w367, "data"=w351, "timeout"=-1.0, "error in"=w354) -> ("task out"=w348:refnum<k21>, "error out"=w350:errorcluster)  [unwired: 9 in, 1 out]
      n134 = call <vilib>:"DAQmx Start Task.vi"("task/channels in"=w348, "error in"=w350) -> ("task out"=w347:refnum<k21>, "error out"=w349:errorcluster)  [unwired: 12 in]
      n135 = while {
        tunnel: w347 -> [w388]
        tunnel: w349 -> [w387]
        tunnel: [w385] -> w361
        tunnel: [w386] -> w364
        stop <- w382 stop-if-true
        n136 = call <vilib>:"DAQmx Is Task Done.vi"("task/channels in"=w388, "error in"=w387) -> ("task out"=w386:refnum<k21>, "error out"=w385:errorcluster)  [unwired: 11 in, 1 out]
        n137 = Unbundle By Name(w385) -> ("status"=w383:bool)
        n138 = local read "Exit"() -> (w381:bool)
        n139 = Wait Until Next ms Multiple(millisecond multiple=u32 100) -> ()  [unwired: 1 out]
        n140 = Compound Arithmetic op=OR(w383, w381) -> (w382:bool)
      }
      n141 = call <vilib>:"DAQmx Stop Task.vi"("task/channels in"=w364, "error in"=w361) -> ("task out"=w363:refnum<k21>, "error out"=w362:errorcluster)  [unwired: 12 in]
      n142 = call <vilib>:"DAQmx Clear Task.vi"("task in"=w363, "error in"=w362) -> ("error out"=w377:errorcluster)  [unwired: 13 in]
      n143 = call <vilib>:"Simple Error Handler.vi"("error in (no error)"=w377) -> ()  [unwired: 4 in, 5 out]
    }
  }
  n144 = while {
    shift-right: [w399] -> _
    shift-left: T1."No Scan" -> [w400]
    shift-right: [w397] -> _
    shift-left: 0 -> [w398]
    tunnel: w47 -> [w392]
    tunnel: [w391] -> _
    tunnel: w46 -> [w390]
    tunnel: [w389] -> _
    stop <- w394 stop-if-true
    # "AUTO SCAN"
    n145 = local read "Scan"() -> (w393:bool)
    n146 = case shown="True" w393 {
      tunnel: w400 -> [w403 w413]
      tunnel: [w403 w412] -> w399
      tunnel: w398 -> [w404 w410]
      tunnel: [w404 w409] -> w397
      tunnel: w392 -> [w402 w408]
      tunnel: [w402 w407] -> w391
      tunnel: w390 -> [w401 w406]
      tunnel: [w401 w405] -> w389
      frame False {
      }
      frame True {
        n147 = case shown="\"Move X\"" w413 {
          selector: w413 -> [w421 _ _ _ _]
          tunnel: [w420 T1."Wait X" w478 w505 w524] -> w412
          tunnel: w410 -> [w419 w457 w476 w504 w523]
          tunnel: [w419 w457 w476 w504 w522] -> w409
          tunnel: w408 -> [w417 w446 w472 w499 w520]
          tunnel: [w415 w451 w474 w502 w518] -> w407
          tunnel: w406 -> [w416 w445 w471 w498 w519]
          tunnel: [w414 w450 w473 w501 w517] -> w405
          frame "No Scan", Default {
            n148 = local read "Scan"() -> (w418:bool)
            n149 = case shown="True" w418 {
              tunnel: w421 -> [w424 _]
              tunnel: [w424 T1."Move X"] -> w420
              tunnel: w417 -> [w423 w440]
              tunnel: w416 -> [w422 w439]
              tunnel: [w423 w429] -> w415
              tunnel: [w422 w428] -> w414
              frame False {
              }
              frame True {
                n150 = call-dynamic "Write Single Coil.vi"("error in"=w439, "coil to write"=FALSE ("X LEFT"), "address"=u16 2049, "Modbus master in"=w440) -> ("error out"=w427:errorcluster, "Modbus master out"=w432:refnum<class "Modbus Master.lvclass">)  [unwired: 6 in]
                n151 = call-dynamic "Write Single Coil.vi"("error in"=w427, "coil to write"=FALSE ("X LEFT"), "address"=u16 2050, "Modbus master in"=w432) -> ("error out"=w426:errorcluster, "Modbus master out"=w431:refnum<class "Modbus Master.lvclass">)  [unwired: 6 in]
                n152 = call-dynamic "Write Single Coil.vi"("error in"=w426, "coil to write"=FALSE ("X LEFT"), "address"=u16 2051, "Modbus master in"=w431) -> ("error out"=w425:errorcluster, "Modbus master out"=w430:refnum<class "Modbus Master.lvclass">)  [unwired: 6 in]
                n153 = call-dynamic "Write Single Coil.vi"("error in"=w425, "coil to write"=FALSE ("X LEFT"), "address"=u16 2052, "Modbus master in"=w430) -> ("error out"=w428:errorcluster, "Modbus master out"=w429:refnum<class "Modbus Master.lvclass">)  [unwired: 6 in]
              }
            }
          }
          frame "Move X" {
            n154 = local read "Count Y step"() -> (w453:i32)
            n155 = Quotient & Remainder(x=w453, y=2) -> (x-y*floor(x/y)=w452:i32)  [unwired: 1 out]
            n156 = Equal?(x=w452, y=0) -> (x = y?=w454:bool)
            n157 = call-dynamic "Write Single Holding Register.vi"("error in"=w445, "register to write"="X Auto Distance", "address"=u16 4100, "Modbus master in"=w446) -> ("error out"=w447:errorcluster, "Modbus master out"=w448:refnum<class "Modbus Master.lvclass">)  [unwired: 6 in]
            n158 = case shown="True" w454 {
              tunnel: w448 -> [w464 w468]
              tunnel: [w463 w466] -> w451
              tunnel: w447 -> [w462 w467]
              tunnel: [w461 w465] -> w450
              frame False {
                n159 = call-dynamic "Write Single Coil.vi"("error in"=w462, "coil to write"=TRUE ("X LEFT"), "address"=u16 2051, "Modbus master in"=w464) -> ("error out"=w461:errorcluster, "Modbus master out"=w463:refnum<class "Modbus Master.lvclass">)  [unwired: 6 in]
              }
              frame True {
                n160 = call-dynamic "Write Single Coil.vi"("error in"=w467, "coil to write"=TRUE ("X LEFT"), "address"=u16 2052, "Modbus master in"=w468) -> ("error out"=w465:errorcluster, "Modbus master out"=w466:refnum<class "Modbus Master.lvclass">)  [unwired: 6 in]
              }
            }
            "Count Y step" <- w457
          }
          frame "Wait X" {
            n161 = local read "X complete"() -> (w475:bool)
            n162 = Wait (ms)(milliseconds to wait=u32 100) -> ()  [unwired: 1 out]
            n163 = case shown="False" w475 {
              tunnel: [T1."Wait X" T1."Move Y"] -> w478
              tunnel: [w480 w485] -> w474
              tunnel: [w479 w484] -> w473
              tunnel: w472 -> [w480 w483]
              tunnel: w471 -> [w479 w482]
              frame False {
              }
              frame True {
                n164 = call-dynamic "Write Single Coil.vi"("error in"=w482, "coil to write"=FALSE ("X LEFT"), "address"=u16 2051, "Modbus master in"=w483) -> ("error out"=w486:errorcluster, "Modbus master out"=w487:refnum<class "Modbus Master.lvclass">)  [unwired: 6 in]
                n165 = call-dynamic "Write Single Coil.vi"("error in"=w486, "coil to write"=FALSE ("X LEFT"), "address"=u16 2052, "Modbus master in"=w487) -> ("error out"=w484:errorcluster, "Modbus master out"=w485:refnum<class "Modbus Master.lvclass">)  [unwired: 6 in]
              }
            }
          }
          frame "Move Y" {
            n166 = local read "Y Step"() -> (w493:dbl)
            n167 = Divide(x="Y Auto Distance", y=w493) -> (x/y=w494:dbl)
            "Step Y Number" <- w494
            n168 = call-dynamic "Write Single Holding Register.vi"("error in"=w498, "register to write"=w493, "address"=u16 4098, "Modbus master in"=w499) -> ("error out"=w496:errorcluster, "Modbus master out"=w497:refnum<class "Modbus Master.lvclass">)  [unwired: 6 in]
            n169 = Greater Or Equal?(x=w504, y=w494) -> (x >= y?=w503:bool)
            n170 = case shown="False" w503 {
              tunnel: [T1."Wait Y" T1."No Scan"] -> w505
              tunnel: w497 -> [w509 w514]
              tunnel: w496 -> [w508 w513]
              tunnel: [w507 w514] -> w502
              tunnel: [w506 w513] -> w501
              frame False {
                n171 = call-dynamic "Write Single Coil.vi"("error in"=w508, "coil to write"=TRUE ("X LEFT"), "address"=u16 2050, "Modbus master in"=w509) -> ("error out"=w506:errorcluster, "Modbus master out"=w507:refnum<class "Modbus Master.lvclass">)  [unwired: 6 in]
              }
              frame True {
                n172 = local write "Scan"(FALSE ("X LEFT")) -> ()
              }
            }
          }
          frame "Wait Y" {
            n173 = local read "Y complete"() -> (w521:bool)
            n174 = case shown="False" w521 {
              tunnel: [T1."Wait Y" T1."Move X"] -> w524
              tunnel: w523 -> [w527 w536]
              tunnel: [w527 w535] -> w522
              tunnel: w520 -> [w526 w532]
              tunnel: w519 -> [w525 w531]
              tunnel: [w526 w530] -> w518
              tunnel: [w525 w529] -> w517
              frame False {
              }
              frame True {
                n175 = Increment(x=w536) -> (x+1=w535:i32)
                n176 = Wait (ms)(milliseconds to wait=u32 100) -> ()  [unwired: 1 out]
                n177 = call-dynamic "Write Single Coil.vi"("error in"=w531, "coil to write"=FALSE ("X LEFT"), "address"=u16 2050, "Modbus master in"=w532) -> ("error out"=w529:errorcluster, "Modbus master out"=w530:refnum<class "Modbus Master.lvclass">)  [unwired: 6 in]
              }
            }
          }
        }
        n178 = Wait Until Next ms Multiple(millisecond multiple=u32 100 ("milliseconds to wait")) -> ()  [unwired: 1 out]
      }
    }
    n179 = local read "Exit"() -> (w396:bool)
    n180 = Compound Arithmetic op=OR(w396, "Stop Scan") -> (w394:bool)
    "Enum" <- w400
  }
  n181 = property class="DAQmx Timing"(reference=w17, error in=w16) -> (reference out=w15:refnum<k21>, error out=w14:errorcluster, "SampClk.Rate"=→"Actual Sample Rate 3":dbl)
  n182 = local read "X Auto Distance"() -> (w58:u16)
  n183 = local read "Y Auto Distance"() -> (w57:i16)
  n184 = local read "Y Step"() -> (w81:dbl)
  n185 = local read "X Step"() -> (w82:dbl)
  n186 = Obtain Queue(max queue size (-1, unlimited)=10000, name (unnamed)="R", element data type=0.0 ("Waveform")) -> (queue out=w83:refnum<queue>)  [unwired: 2 in, 2 out]
  n187 = call-poly <vilib>:"DAQmx Trigger.vi"("task/channels in"=w15, "source"="Pulser Trigger 2", "edge"="Edge 2", "error in"=w14) -> ("task out"=w5:refnum<k21>, "error out"=w4:errorcluster)  [unwired: 10 in]
  n188 = Quotient & Remainder(x=w57, y=w81) -> (floor(x/y)=w69:dbl)  [unwired: 1 out]
  n189 = Quotient & Remainder(x=w58, y=w82) -> (floor(x/y)=w76:dbl)  [unwired: 1 out]
  n190 = Increment(x=w69) -> (x+1=w67:dbl)
  n191 = Build Array(w76, w67) -> (w74:dbl[])
  n192 = TDMS Write(0:w78, 5:"Freq_Sampling_SizeX_SizeY" ("group name in (Untitled)"), 9:w74) -> (4:w77:refnum<k34>)  [unwired: 3 in, 3 out]
  n193 = Obtain Queue(max queue size (-1, unlimited)=2 ("최대 큐 크기(-1,제한없음)"), name (unnamed)="2D data", element data type=dbl[][] [] ("initialized array")) -> (queue out=w71:refnum<queue>)  [unwired: 2 in, 2 out]
  n194 = property class="DAQmx Trigger"(reference=w5, error in=w4, "Start.Retriggerable"=TRUE) -> (reference out=w2:refnum<k21>, error out=w1:errorcluster)
  n195 = case shown="\"SCAN MODE\", Default" "Tab Control 2" {
    tunnel: [w570 w799 w821] -> w40
    tunnel: [w569 w798 w820] -> w41
    tunnel: w83 -> [w543 _ w819]
    tunnel: w76 -> [w555 _ _]
    tunnel: w67 -> [w556 _ _]
    tunnel: w77 -> [w563 _ _]
    tunnel: "Waveform" ("group name in (Untitled)") -> [w560 _ _]
    tunnel: w71 -> [w557 _ _]
    tunnel: w30 -> [w545 w799 w823]
    tunnel: w29 -> [w544 w798 w822]
    tunnel: w2 -> [w542 w797 w818]
    tunnel: w1 -> [w541 w796 w817]
    tunnel: [w540 w797 w816] -> w10
    tunnel: [w539 w796 w815] -> w9
    frame "SCAN MODE", Default {
      # "Column"
      # "Row"
      n196 = local read "3D Surface"() -> (w546:refnum<k7>)
      n197 = Initialize Array(0.0 ("element"), w555, w556) -> (w567:dbl[][])
      n198 = Matrix Size(0:w567) -> (1:w547:i32, 2:w548:i32)
      n199 = Decrement(x=w547) -> (x-1=w551:i32)
      n200 = Decrement(x=w548) -> (x-1=w550:i32)
      n201 = call "Surface_AxesScale.vi"("Y-axis Max"=w550, "X-axis max"=w551, "3D Surface"=w546, "Auto Scale"=FALSE) -> ()  [unwired: 8 in]
      n202 = while {
        tunnel: w557 -> [w788]
        tunnel: w556 -> [_]
        tunnel: w555 -> [_]
        tunnel: [w785] -> w554
        stop <- w786 stop-if-true
        n203 = local read "Output"() -> (w779:dbl[][])
        n204 = local read "No. Y"() -> (w783:i32)
        n205 = call "CursorPosition.vi"("Cursor No."=1.0, "Cursor"="Cursor", "3D Surface Analysis"="3D Surface") -> ("Cursor Y"=w781:dbl)  [unwired: 6 in, 2 out]
        n206 = Dequeue Element(queue=w788, timeout in ms (-1)=3000) -> (queue out=w785:refnum<queue>)  [unwired: 1 in, 3 out]
        n207 = Add(x=w783, y=w781) -> (x+y=w782:dbl)
        n208 = Index Array(array=w779, index (col)=w782) -> (element=→"Feature extraction scan":dbl[])  [unwired: 1 in]
        n209 = call <vilib>:"3D Surface.vi"("z matrix"=w779, "3D graph"="3D Surface") -> ()  [unwired: 8 in, 2 out]
        n210 = case shown="True" "Save CSV" {
          tunnel: w779 -> [_ w795]
          frame False {
          }
          frame True {
            n211 = call-poly <vilib>:"Write Delimited Spreadsheet.vi"("file path (dialog if empty)"="file path (dialog if empty)", "format (%.3f)"="%.3f", "2D data"=w795, "delimiter (\\t)"="," ("delimiter (\\t)")) -> ()  [unwired: 10 in, 2 out]
            n212 = local write "Save CSV"(FALSE) -> ()
          }
        }
        n213 = local read "Completed"() -> (w784:bool)
        n214 = local read "Exit"() -> (w787:bool)
        n215 = Compound Arithmetic op=OR(w784, w787) -> (w786:bool)
        n216 = Wait Until Next ms Multiple(millisecond multiple=u32 100 ("ms 배수")) -> ()  [unwired: 1 out]
      }
      n217 = while {
        tunnel: [w624] -> w570
        tunnel: [w623] -> w569
        tunnel: w543 -> [w622]
        tunnel: w545 -> [w617]
        tunnel: w544 -> [w616]
        tunnel: w542 -> [w615]
        tunnel: w541 -> [w614]
        tunnel: [w613] -> w540
        tunnel: [w612] -> w539
        stop <- w619 stop-if-true
        n218 = case shown="True" "Scan" {
          tunnel: [w628 w637] -> w624
          tunnel: [w627 w636] -> w623
          tunnel: w622 -> [_ w635]
          tunnel: w617 -> [w628 w634]
          tunnel: w616 -> [w627 w633]
          tunnel: w615 -> [w626 w632]
          tunnel: w614 -> [w625 w631]
          tunnel: [w626 w630] -> w613
          tunnel: [w625 w629] -> w612
          frame False {
          }
          frame True {
            n219 = while {
              tunnel: [w649] -> w637
              tunnel: [w648] -> w636
              tunnel: w635 -> [w642]
              tunnel: w634 -> [w646]
              tunnel: w633 -> [w645]
              tunnel: w632 -> [w639]
              tunnel: w631 -> [w638]
              tunnel: [w639] -> w630
              tunnel: [w638] -> w629
              stop <- w661 stop-if-true
              n220 = First Call?() -> (First Call?: T/F=w660:bool)
              n221 = case shown="True" w660 {
                tunnel: w646 -> [w668 w670]
                tunnel: w645 -> [w667 w669]
                tunnel: [w668 w670] -> w643
                tunnel: [w667 w669] -> w644
                frame False {
                }
                frame True {
                  n222 = local read "Motor Pulses X"() -> (→"Init pulses":i32)
                }
              }
              n223 = VISA Write(VISA resource name=w643, write buffer="SNAP? 2,3\n", error in (no error)=w644) -> (VISA resource name out=w656:refnum<visa-resource-name>, error out=w655:errorcluster)  [unwired: 1 out]
              n224 = flat-sequence {
                tunnel: w656 -> [w665]
                tunnel: [w665] -> w658
                tunnel: w655 -> [w664]
                tunnel: [w664] -> w657
                frame #0 {
                  n225 = Wait (ms)(milliseconds to wait=u32 10) -> ()  [unwired: 1 out]
                }
              }
              n226 = VISA Read(VISA resource name=w658, byte count=u32 1024, error in (no error)=w657) -> (VISA resource name out=w649:refnum<visa-resource-name>, read buffer=w653:string, error out=w648:errorcluster)  [unwired: 1 out]
              n227 = Unbundle By Name(w648) -> ("status"=w647:bool)
              n228 = local read "Completed"() -> (w663:bool)
              n229 = local read "Exit"() -> (w662:bool)
              n230 = Match Pattern(string=w653, regular expression=",") -> (before substring=w651:string, after substring=w650:string)  [unwired: 1 in, 2 out]
              n231 = Fract/Exp String To Number(string=w650) -> ()  [unwired: 3 in, 2 out]
              n232 = Compound Arithmetic op=OR(w647, w663, w662) -> (w661:bool)
              n233 = Fract/Exp String To Number(string=w651) -> (number=w641:dbl)  [unwired: 3 in, 1 out]
              n234 = Enqueue Element(queue=w642, element=w641, timeout in ms (-1)=1000) -> ()  [unwired: 1 in, 3 out]
            }
          }
        }
        n235 = local read "Completed"() -> (w620:bool)
        n236 = local read "Exit"() -> (w621:bool)
        n237 = Compound Arithmetic op=OR(w620, w621) -> (w619:bool)
      }
      n238 = while {
        shift-right: [w691] -> _
        shift-left: 0 -> [w693]
        shift-right: [w690] -> _
        shift-left: 0 -> [w692]
        tunnel: w543 -> [w689]
        shift-right: [w681] -> w553
        shift-left: w567 -> [w688]
        shift-right: [w684] -> _
        shift-left: TRUE ("Output Direction") -> [w685]
        tunnel: w557 -> [w683]
        tunnel: [w682] -> w558
        stop <- w686 stop-if-true
        n239 = local read "Scan"() -> (w680:bool)
        n240 = local read "Completed"() -> (w679:bool)
        n241 = Compound Arithmetic op=AND(invert w680, invert w679) -> (w678:bool)
        n242 = case shown="True" w678 {
          tunnel: w693 -> [w707 w750]
          tunnel: w692 -> [w706 w749]
          tunnel: [w705 w750] -> w691
          tunnel: [w700 w749] -> w690
          tunnel: w689 -> [w694 w744]
          tunnel: w688 -> [w704 w746]
          tunnel: [w697 w732] -> w681
          tunnel: [w703 _] -> w677
          tunnel: w685 -> [w702 w748]
          tunnel: [w701 w748] -> w684
          tunnel: w683 -> [w698 w734]
          tunnel: [w696 w744] -> w682
          frame False {
            n243 = Dequeue Element(queue=w694, timeout in ms (-1)=5000) -> (queue out=w696:refnum<queue>, element=w699:dbl)  [unwired: 1 in, 2 out]
            "element" <- w699
            n244 = call "EletoMatr_1channel.vi"("Input Array X"=w704, "Input data"=w699, "In Row"=w707, "In Column"=w706, "Input Direction"=w702) -> ("Completed"=w703:bool, "Out Array X"=w697:dbl[][], "Out Row"=w705:i32, "Output Direction"=w701:bool, "Out Column"=w700:i32)  [unwired: 6 in]
            n245 = Lossy Enqueue Element(queue=w698, element=w697) -> ()  [unwired: 1 in, 4 out]
          }
          frame True {
            n246 = Wait Until Next ms Multiple(millisecond multiple=u32 100 ("ms 배수")) -> ()  [unwired: 1 out]
            n247 = call "TDMS_Open.vi"("Input 2D"=w746, "Open"="Open tdms") -> ("Output 2D"=w712:dbl[][])  [unwired: 8 in, 1 out]
            n248 = case shown="True" "Open tdms" {
              tunnel: w712 -> [_ w751]
              frame False {
              }
              frame True {
                n249 = global write "Global_data.vi" "global 2d graph"(w751) -> ()
              }
            }
            n250 = call "RepairLine.vi"("Repair Line Col"="Repair Line Col", "Repair Line Row"="Repair Line Row", "Line Col"="Line Col", "Line Row"="Line Row", "Array In"=w712) -> ("Array Repaired"=w726:dbl[][])  [unwired: 6 in]
            n251 = call "CSV Open.vi"("2D Array In"=w726, "Open"="Open csv") -> ("2D Array Out"=w733:dbl[][])  [unwired: 9 in]
            n252 = call "Backdata.vi"("Backindex"="Backindex", "Array in"=w733, "Backdata"="Backdata 2") -> ("Array out"=w715:dbl[][])
            n253 = call "TrimXY.vi"("X-max"="Y-max", "X-min"="Y-min", "Y-max"="X-max", "Y-min"="X-min", "Array In"=w715, "Trim data"="Trim data") -> ("Array Trim Out"=w714:dbl[][])  [unwired: 5 in]
            n254 = global read "Global_data.vi" "global 2d graph"() -> (w709:dbl[][])
            n255 = call "Inverse.vi"(10:"Inverse"=w714, 11:"Inverse"="Inverse") -> ("Array out"=w710:dbl[][])  [unwired: 9 in]
            n256 = call "Return data.vi"("Array Return"=w709, "Array Input"=w710, "Return"="Return") -> ("Array out"=w708:dbl[][])  [unwired: 8 in]
            n257 = call "Abs.vi"("Input"=w708, "Abs"="Abs") -> ("Array out"=w738:dbl[][])  [unwired: 9 in]
            n258 = call "DiffX.vi"("Array in"=w738, "DiffX"="DiffX") -> ("Array out"=w742:dbl[][])  [unwired: 1 in]
            n259 = call "DiffY.vi"("Array in"=w742, "DiffY"="DiffY") -> ("Array out"=w740:dbl[][])  [unwired: 1 in]
            n260 = call "Odd.vi"("Odd"="Odd", "Array In"=w740) -> ("Array Out"=w730:dbl[][])  [unwired: 9 in]
            n261 = call "Filter_Lowpass - 2D.vi"("Filter"="Filter", "Input 2D"=w730, "low cutoff freq: fl"="low cutoff freq: fl") -> ("Output"=w729:dbl[][])  [unwired: 6 in]
            n262 = case shown="True" TRUE {
              tunnel: w729 -> [w752 w753]
              tunnel: [w752 w753] -> w732
              tunnel: w734 -> [_ w754]
              frame False {
              }
              frame True {
                n263 = local read "3D Surface"() -> (w758:refnum<k7>)
                n264 = Matrix Size(0:w753) -> (1:w759:i32, 2:w756:i32)
                n265 = Decrement(x=w759) -> (x-1=w757:i32)
                n266 = Decrement(x=w756) -> (x-1=w755:i32)
                n267 = Lossy Enqueue Element(queue=w754, element=w753) -> ()  [unwired: 1 in, 4 out]
                n268 = call "Surface_AxesScale.vi"("Y-axis Max"=w755, "X-axis max"=w757, "3D Surface"=w758, "Auto Scale"=FALSE) -> ()  [unwired: 8 in]
              }
            }
          }
        }
        "Output" <- w681
        n269 = local read "Exit"() -> (w687:bool)
        n270 = case shown="False" w677 {
          selector: w677 -> [w761 w762]
          tunnel: [w761 w762] -> w676
          frame False {
          }
          frame True {
            n271 = Wait (ms)(milliseconds to wait=u32 200) -> ()  [unwired: 1 out]
          }
        }
        "Completed" <- w676
        n272 = Compound Arithmetic op=OR(w676, w687) -> (w686:bool)
        "No. Y" <- w692
        "No. X" <- w693
      }
      n273 = while {
        tunnel: w543 -> [w581]
        shift-right: [w578] -> _
        shift-left: 0 -> [w579]
        tunnel: w563 -> [w577]
        tunnel: [w576] -> w562
        tunnel: [w575] -> w561
        tunnel: w560 -> [w574]
        stop <- w571 stop-if-true
        n274 = local read "Scan"() -> (w580:bool)
        n275 = case shown="True" w580 {
          tunnel: w581 -> [_ w585]
          tunnel: w579 -> [w584 w591]
          tunnel: [w584 w590] -> w578
          tunnel: w577 -> [w582 w589]
          tunnel: [w582 w588] -> w576
          tunnel: [_ w587] -> w575
          tunnel: w574 -> [_ w586]
          frame False {
            n276 = Wait Until Next ms Multiple(millisecond multiple=u32 100 ("ms 배수")) -> ()  [unwired: 1 out]
          }
          frame True {
            n277 = local read "Pulser Cycles"() -> (w592:i32)
            n278 = Increment(x=w591) -> (x+1=w590:i32)
            n279 = Quotient & Remainder(x=w590, y=w592) -> (x-y*floor(x/y)=w593:i32)  [unwired: 1 out]
            n280 = Equal To 0?(x=w593) -> (x = 0?=w594:bool)
            n281 = case shown="True" w594 {
              tunnel: w589 -> [w595 w602]
              tunnel: [w595 w600] -> w588
              tunnel: [_ w599] -> w587
              tunnel: w586 -> [_ w601]
              tunnel: w585 -> [_ w597]
              frame False {
                n282 = disable-structure shown="Enabled" {
                  frame Disabled {
                    n283 = Wait Until Next ms Multiple(millisecond multiple=u32 100 ("ms 배수")) -> ()  [unwired: 1 out]
                  }
                  frame Enabled {
                  }
                }
              }
              frame True {
                n284 = local read "Get data"() -> (w598:bool)
                n285 = case shown="True" w598 {
                  tunnel: w602 -> [w603 w611]
                  tunnel: w601 -> [_ w610]
                  tunnel: [w603 w609] -> w600
                  tunnel: [_ w608] -> w599
                  tunnel: w597 -> [_ w606]
                  frame False {
                  }
                  frame True {
                    n286 = Dequeue Element(queue=w606) -> (element=w605:dbl)  [unwired: 2 in, 3 out]
                    n287 = Build Array(w605) -> (w604:dbl[])
                    n288 = TDMS Write(0:w611, 5:w610, 9:w604) -> (4:w609:refnum<k34>, 15:w608:errorcluster)  [unwired: 3 in, 2 out]
                    n289 = local write "Get data"(FALSE ("Acquire")) -> ()
                  }
                }
              }
            }
          }
        }
        n290 = local read "Completed"() -> (w573:bool)
        n291 = local read "Exit"() -> (w572:bool)
        n292 = Compound Arithmetic op=OR(w573, w572) -> (w571:bool)
        "No.data" <- w579
      }
      n293 = Release Queue(queue=w554) -> ()  [unwired: 2 in, 3 out]
      n294 = while {
        stop <- w764 stop-if-true
        n295 = event shown="[2] \"Max\", \"Min\", \"ColorMapAutoScale\": Value Change" {
          selector: _ -> [_ _ _]
          dyn-events: _ -> [_ _ _]
          timeout: _ -> [_ _ _]
          tunnel: [_ w768 _] -> w764
          event "Plot style", "ViewMode": Value Change {
            n296 = event-data() -> ()  [unwired: 1 in, 2 out]
            n297 = local read "3D Surface"() -> (w767:refnum<k7>)
            n298 = property class="CWGraph3D"(reference=w767, "ViewMode"="ViewMode") -> ()  [unwired: 1 in, 2 out]
            n299 = call <vilib>:"Basic Properties.vi"("3D graph"=w767, "plot style"="Plot style") -> ()  [unwired: 12 in, 2 out]
          }
          event "Exit": Value Change {
            n300 = event-data() -> ()  [unwired: 1 in, 1 out]
            n301 = local read "Exit"() -> (w768:bool)
          }
          event "Max", "Min", "ColorMapAutoScale": Value Change {
            n302 = event-data() -> ()  [unwired: 1 in, 5 out]
            n303 = local read "3D Surface"() -> (w769:refnum<k7>)
            n304 = call "Surface_ColorScale.vi"("ColorMapAutoScale"="ColorMapAutoScale", "Min"="Min", "Max"="Max", "3D Surface_"=w769) -> ("Min 2"=w773:dbl, "Max 2"=w772:dbl)  [unwired: 1 in, 2 out]
            n305 = local write "Max"(w772) -> ()
            n306 = local write "Min"(w773) -> ()
          }
        }
      }
      n307 = while {
        tunnel: w553 -> [w674]
        stop <- w673 stop-if-true
        n308 = call "CSV Save.vi"("Array"=w674, "Save Button"="Save Scan mode") -> ()  [unwired: 9 in, 1 out]
        n309 = Wait Until Next ms Multiple(millisecond multiple=u32 100 ("ms 배수")) -> ()  [unwired: 1 out]
        n310 = local read "Exit"() -> (w673:bool)
      }
      n311 = Release Queue(queue=w558) -> ()  [unwired: 2 in, 3 out]
      n312 = TDMS Close(8:w561, 11:w562) -> (0:w559:errorcluster)  [unwired: 1 out]
      n313 = call <vilib>:"Simple Error Handler.vi"("error in (no error)"=w559) -> ()  [unwired: 2 in, 7 out]
    }
    frame "LIFT-OFF MEASUREMENT" {
      n314 = while {
        shift-right: [w809] -> _
        shift-left: "2D Array In" -> [w810]
        stop <- w814 stop-if-true
        n315 = call "CSV Open.vi"("2D Array In"=w810, "Open"="Open") -> ("2D Array Out"=w809:dbl[][])  [unwired: 9 in]
        n316 = Delete From Array(array=w809, index (col)=0 ("disabled index (col)")) -> (array with subset deleted=w811:dbl[][])  [unwired: 2 in, 1 out]
        n317 = Subtract(x=w811, y=w809) -> (x-y=w807:dbl[][])
        n318 = Transpose 2D Array(2D array=w807) -> (transposed array=w804:dbl[][])
        n319 = call "Filter_Lowpass - 2D.vi"("Filter"="Filter lf", "Input 2D"=w804, "low cutoff freq: fl"="Low cutoff freq: fl") -> ("Output"=w806:dbl[][])  [unwired: 6 in]
        n320 = Transpose 2D Array(2D array=w806) -> (transposed array=w803:dbl[][])
        n321 = Select(t=w803, s="View Mode", f=w809) -> (s? t:f=→"Hall sensors signal lf":dbl[][])
        n322 = local read "Exit"() -> (w814:bool)
      }
    }
    frame "TEST MODE           " {
      n323 = while {
        tunnel: w823 -> [w833]
        tunnel: w822 -> [w832]
        tunnel: [w831] -> w821
        tunnel: [w830] -> w820
        tunnel: w819 -> [w829]
        tunnel: [w828] -> w816
        tunnel: w818 -> [w828]
        tunnel: [w827] -> w815
        tunnel: w817 -> [w827]
        stop <- w848 stop-if-true
        n324 = VISA Write(VISA resource name=w833, write buffer="SNAP? 2,3\n", error in (no error)=w832) -> (VISA resource name out=w842:refnum<visa-resource-name>, error out=w841:errorcluster)  [unwired: 1 out]
        n325 = flat-sequence {
          tunnel: w842 -> [w850]
          tunnel: [w850] -> w844
          tunnel: w841 -> [w849]
          tunnel: [w849] -> w843
          frame #0 {
            n326 = Wait (ms)(milliseconds to wait=u32 10) -> ()  [unwired: 1 out]
          }
        }
        n327 = VISA Read(VISA resource name=w844, byte count=u32 1024, error in (no error)=w843) -> (VISA resource name out=w831:refnum<visa-resource-name>, read buffer=w839:string, error out=w830:errorcluster)  [unwired: 1 out]
        n328 = Match Pattern(string=w839, regular expression=",") -> (before substring=w837:string, after substring=w836:string)  [unwired: 1 in, 2 out]
        n329 = Fract/Exp String To Number(string=w836) -> ()  [unwired: 3 in, 2 out]
        n330 = Fract/Exp String To Number(string=w837) -> (number=w835:dbl)  [unwired: 3 in, 1 out]
        n331 = Enqueue Element(queue=w829, element=w835, timeout in ms (-1)=1000) -> ()  [unwired: 1 in, 3 out]
        n332 = local read "Exit"() -> (w846:bool)
        n333 = Unbundle By Name(w830) -> ("status"=w847:bool)
        n334 = Or(x=w847, y=w846) -> (x .or. y?=w848:bool)
      }
      n335 = while {
        tunnel: w819 -> [w826]
        stop <- w824 stop-if-true
        n336 = Dequeue Element(queue=w826) -> (element=→"Waveform Chart":dbl)  [unwired: 2 in, 3 out]
        n337 = local read "Exit"() -> (w824:bool)
      }
    }
  }
  n338 = call-dynamic "Shutdown.vi"("error in"=w43, "Modbus master in"=w42) -> ()  [unwired: 9 in, 1 out]
  n339 = call-dynamic "Shutdown.vi"("error in"=w44, "Modbus master in"=w45) -> ()  [unwired: 9 in, 1 out]
  n340 = VISA Close(VISA resource name=w40, error in (no error)=w41) -> (error out=w39:errorcluster)
  n341 = call <vilib>:"DAQmx Clear Task.vi"("task in"=w10, "error in"=w9) -> ("error out"=w20:errorcluster)  [unwired: 13 in]
  n342 = call <vilib>:"Simple Error Handler.vi"("error in (no error)"=w20) -> ()  [unwired: 4 in, 5 out]
  n343 = call <vilib>:"Simple Error Handler.vi"("error in (no error)"=w39) -> ()  [unwired: 4 in, 5 out]
  n344 = call <vilib>:"Simple Error Handler.vi"() -> ()  [unwired: 5 in, 5 out]
  "Init pulses" <- 0 ("Init pulses")
